vi "Lab Panel V2.8.vi"() -> ()   [LabVIEW 2013]
uses:
  <vilib>/Platform/TimedLoop/XDataNode/timing_clust.ctl
  <vilib>/Platform/TimedLoop/XDataNode/nitl_modes.ctl
  <vilib>/Platform/TimedLoop/XDataNode/wakeup.ctl
  <vilib>/platform/TimedLoop/XDataNode/XDataNode.xnode
  <vilib>/Platform/TimedLoop/XDataNode/XDNodeRunTimeDep.lvlib
panel:
  out "TEMP update":bool
  out "AI update":bool
  in  "stop":bool
  in  "Tab Control 2":T1(tab)
  out "LAB05-2 (SIG)":T2 {"PF" format="%.2f"; "AMPS" format="%.1f"}
  out "LAB05-1 (SIG)":T2 {"PF" format="%.2f"; "AMPS" format="%.1f"}
  out "LAB04-2 (SIG)":T2 {"PF" format="%.2f"; "AMPS" format="%.1f"}
  out "LAB04-1 (SIG)":T2 {"PF" format="%.2f"; "AMPS" format="%.1f"}
  out "LAB03-2 (SIG)":T2 {"PF" format="%.2f"; "AMPS" format="%.1f"}
  out "LAB03-1 (SIG)":T2 {"PF" format="%.2f"; "AMPS" format="%.1f"}
  out "LAB02-2 (SIG)":T2 {"PF" format="%.2f"; "AMPS" format="%.1f"}
  in  "LAB01-1RUN":bool
  in  "LAB05-1 (O/I)":bool
  in  "LAB05-2 (O/I)":bool
  in  "LAB04-1 (O/I)":bool
  in  "LAB04-2 (O/I)":bool
  in  "LAB02-1 (O/I)":bool
  in  "LAB02-2 (O/I)":bool
  in  "LAB01-2 (O/I)":bool
  in  "LAB01-1 (O/I)":bool
  in  "LAB03-1 (O/I)":bool
  in  "LAB05-2 RUN":bool
  in  "LAB05-1 RUN":bool
  in  "LAB04-2 RUN":bool
  in  "LAB04-1 RUN":bool
  in  "LAB03-2 RUN":bool
  in  "LAB03-1 RUN":bool
  in  "LAB02-2 RUN":bool
  in  "LAB02-1 RUN":bool
  in  "LAB01-2 RUN":bool
  in  "LAB05-2 SELECT":T3(radio)
  in  "LAB05-1 SELECT":T3(radio)
  in  "LAB04-2 SELECT":T3(radio)
  in  "LAB04-1 SELECT":T3(radio)
  in  "LAB03-2 SELECT":T3(radio)
  in  "LAB03-1 SELECT":T3(radio)
  in  "LAB02-2 SELECT":T3(radio)
  in  "LAB02-1 SELECT":T3(radio)
  in  "LAB01-2 SELECT":T3(radio)
  in  "LAB01-1 SELECT":T3(radio)
  in  "LAB03-2 (O/I)":bool
  out "LAB01-1 (SIG)":T2 {"PF" format="%.2f"; "AMPS" format="%.1f"}
  out "LAB01-2 (SIG)":T2 {"PF" format="%.2f"; "AMPS" format="%.1f"}
  out "LAB02-1 (SIG)":T2 {"PF" format="%.2f"; "AMPS" format="%.1f"}
  out "LAB05-2 (DISP)":T4 {"MINS" format="%.2g"}
  out "LAB05-1 (DISP)":T4 {"MINS" format="%.2g"}
  out "LAB04-2 (DISP)":T4 {"MINS" format="%.2g"}
  out "LAB04-1 (DISP)":T4 {"MINS" format="%.2g"}
  out "LAB03-2 (DISP)":T4 {"MINS" format="%.2g"}
  out "LAB03-1 (DISP)":T4 {"MINS" format="%.2g"}
  in  "LAB05-2 (SET)":T5
  in  "LAB05-1 (SET)":T5
  in  "LAB04-2 (SET)":T5
  in  "LAB04-1 (SET)":T5
  in  "LAB03-2 (SET)":T5
  in  "LAB03-1 (SET)":T5
  out "LAB02-2 (DISP)":T4 {"MINS" format="%.2g"}
  out "LAB02-1 (DISP)":T4 {"MINS" format="%.2g"}
  in  "LAB02-2 (SET)":T5
  in  "LAB02-1 (SET)":T5
  out "LAB05-2 (RESULT)":bool
  out "LAB05-1 (RESULT)":bool
  out "LAB04-2 (RESULT)":bool
  out "LAB04-1 (RESULT)":bool
  out "LAB03-2 (RESULT)":bool
  out "LAB03-1 (RESULT)":bool
  out "LAB02-2 (RESULT)":bool
  out "LAB02-1 (RESULT)":bool
  out "LAB01-2 (RESULT)":bool
  out "LAB01-1 (RESULT)":bool
  in  "LAB01-1 (SET)":T5
  in  "LAB01-2(SET)":T5
  out "LAB01-1 (DISP)":T4 {"MINS" format="%.2g"}
  out "LAB01-2 (DISP)":T4 {"MINS" format="%.2f"}
  out "LAB05-2 (TEMP START)":cluster{"TL":dbl, "TN":dbl}
  out "LAB04-2 (TEMP START)":cluster{"TL":dbl, "TN":dbl}
  out "LAB03-2 (TEMP START)":cluster{"TL":dbl, "TN":dbl}
  out "LAB02-2 (TEMP START)":cluster{"TL":dbl, "TN":dbl}
  out "LAB01-2 (TEMP START)":cluster{"TL":dbl, "TN":dbl}
  out "LAB05-1 (TEMP START)":cluster{"TL":dbl, "TN":dbl}
  out "LAB04-1 (TEMP START)":cluster{"TL":dbl, "TN":dbl}
  out "LAB03-1 (TEMP START)":cluster{"TL":dbl, "TN":dbl}
  out "LAB02-1 (TEMP START)":cluster{"TL":dbl, "TN":dbl}
  out "LAB01-1 (TEMP START)":cluster{"TL":dbl, "TN":dbl}
  in  "JIG ON TIME (S)":dbl=1.0 min=1.0 max=10.0 step=0.5 format="%.1g"
  in  "JIG OFF TIME (S)":dbl=2.0 min=2.0 max=10.0 step=0.5 format="%.1g"
  out "LAB01-1 (JIG)":bool
  out "LAB01-2 (JIG)":bool
  out "LAB02-1 (JIG)":bool
  out "LAB02-2 (JIG)":bool
  out "LAB03-1 (JIG)":bool
  out "LAB03-2 (JIG)":bool
  out "LAB04-1 (JIG)":bool
  out "LAB04-2 (JIG)":bool
  out "LAB05-1 (JIG)":bool
  out "LAB05-2 (JIG)":bool
  out "LAB01 (CAL)":T6 {"2 (TN) cal" min=0.0 step=0.01 format="%.2f"; "2 (TL) cal" min=0.0 step=0.01 format="%.2f"; "2 (PF) cal" min=0.0 step=0.01 format="%.2f"; "2 (V) cal" min=0.0 step=0.01 format="%.2f"; "2 (A) cal" min=0.0 step=0.01 format="%.2f"; "1 (TN) cal" min=0.0 step=0.01 format="%.2f"; "1 (TL) cal" min=0.0 step=0.01 format="%.2f"; "1 (PF) cal" min=0.0 step=0.01 format="%.2f"; "1 (V) cal" min=0.0 step=0.01 format="%.2f"; "1  (A) cal" min=0.0 step=0.01 format="%.2f"}
  out "LAB03 (CAL)":T6 {"2 (TN) cal" min=0.0 step=0.01 format="%.2f"; "2 (TL) cal" min=0.0 step=0.01 format="%.2f"; "2 (PF) cal" min=0.0 step=0.01 format="%.2f"; "2 (V) cal" min=0.0 step=0.01 format="%.2f"; "2 (A) cal" min=0.0 step=0.01 format="%.2f"; "1 (TN) cal" min=0.0 step=0.01 format="%.2f"; "1 (TL) cal" min=0.0 step=0.01 format="%.2f"; "1 (PF) cal" min=0.0 step=0.01 format="%.2f"; "1 (V) cal" min=0.0 step=0.01 format="%.2f"; "1  (A) cal" min=0.0 step=0.01 format="%.2f"}
  out "LAB02 (CAL)":T7 {"2 (TN) cal" min=0.0 step=0.01 format="%.2f"; "2 (TL) cal" min=0.0 step=0.01 format="%.2f"; "2 (PF) cal" min=0.0 step=0.01 format="%.2f"; "2 (V) cal" min=0.0 step=0.01 format="%.2f"; "2 (A) cal" min=0.0 step=0.01 format="%.2f"; "1 (TN) cal" min=0.0 step=0.01 format="%.2f"; "1 (TL) cal" min=0.0 step=0.01 format="%.2f"; "1 (PF) cal" min=0.0 step=0.01 format="%.2f"; "1 (V) cal" min=0.0 step=0.01 format="%.2f"; "1 (A) cal" min=0.0 step=0.01 format="%.2f"}
  out "LAB05 (CAL)":T6 {"2 (TN) cal" min=0.0 step=0.01 format="%.2f"; "2 (TL) cal" min=0.0 step=0.01 format="%.2f"; "2 (PF) cal" min=0.0 step=0.01 format="%.2f"; "2 (V) cal" min=0.0 step=0.01 format="%.2f"; "2 (A) cal" min=0.0 step=0.01 format="%.2f"; "1 (TN) cal" min=0.0 step=0.01 format="%.2f"; "1 (TL) cal" min=0.0 step=0.01 format="%.2f"; "1 (PF) cal" min=0.0 step=0.01 format="%.2f"; "1 (V) cal" min=0.0 step=0.01 format="%.2f"; "1  (A) cal" min=0.0 step=0.01 format="%.2f"}
  out "LAB04 (CAL)":T6 {"2 (TN) cal" min=0.0 step=0.01 format="%.2f"; "2 (TL) cal" min=0.0 step=0.01 format="%.2f"; "2 (PF) cal" min=0.0 step=0.01 format="%.2f"; "2 (V) cal" min=0.0 step=0.01 format="%.2f"; "2 (A) cal" min=0.0 step=0.01 format="%.2f"; "1 (TN) cal" min=0.0 step=0.01 format="%.2f"; "1 (TL) cal" min=0.0 step=0.01 format="%.2f"; "1 (PF) cal" min=0.0 step=0.01 format="%.2f"; "1 (V) cal" min=0.0 step=0.01 format="%.2f"; "1  (A) cal" min=0.0 step=0.01 format="%.2f"}
  out "calibration file error out":errorcluster
  in  "CALIBRATE":bool
  out "LAB01-1 (FAIL HI)":dbl
  out "LAB01-1 (FAIL LO)":dbl
  in  "Amps fail level":dbl=1.0 min=1.0 max=100.0 step=1.0
  in  "Tab Control":T8(tab)
  out "LAB01-2 (GRAPH)":dynamicdata(graph)
  out "LAB01-1 (GRAPH)":dynamicdata(graph)
  out "LAB02-2 (GRAPH)":dynamicdata(graph)
  out "LAB02-1 (GRAPH)":dynamicdata(graph)
  out "LAB03-2 (GRAPH)":dynamicdata(graph)
  out "LAB03-1 (GRAPH)":dynamicdata(graph)
  out "LAB04-2 (GRAPH)":dynamicdata(graph)
  out "LAB04-1 (GRAPH)":dynamicdata(graph)
  out "LAB05-2 (GRAPH)":dynamicdata(graph)
  out "LAB05-1 (GRAPH)":dynamicdata(graph)
  out "LAB05 TEMP":T9
  out "LAB04 TEMP":T9
  out "LAB02 TEMP":T9
  out "LAB01 TEMP":T9
  out "LAB03 TEMP":T9
  out "Analog Error Array":errorcluster[](array[cluster])
  out "AI loop time":dbl format="%.6g"
  out "loops":dbl
  in  "loop  delay(mS)":dbl
  out "on loops":dbl
  out "off loops":dbl
  out "jig cycle":dbl
  out "LAB01-1 (TDMS)":refnum<k34>
  out "data file error":errorcluster
  out "LAB02-1 (TDMS)":refnum<k34>
  out "LAB01-2 (TDMS)":refnum<k34>
  out "LAB02-2 (TDMS)":refnum<k34>
  out "LAB03-1 (TDMS)":refnum<k34>
  out "LAB03-2 (TDMS)":refnum<k34>
  out "LAB04-1 (TDMS)":refnum<k34>
  out "LAB04-2 (TDMS)":refnum<k34>
  out "LAB05-1 (TDMS)":refnum<k34>
  out "LAB05-2 (TDMS)":refnum<k34>
  # "LAB01"
  # "LAB02"
  # "LAB05"
  # "LAB03"
  # "LAB04"
  # "LAB01"
  # "LAB02"
  # "LAB03"
  # "LAB04"
  # "LAB05"
  # "JIG SET"
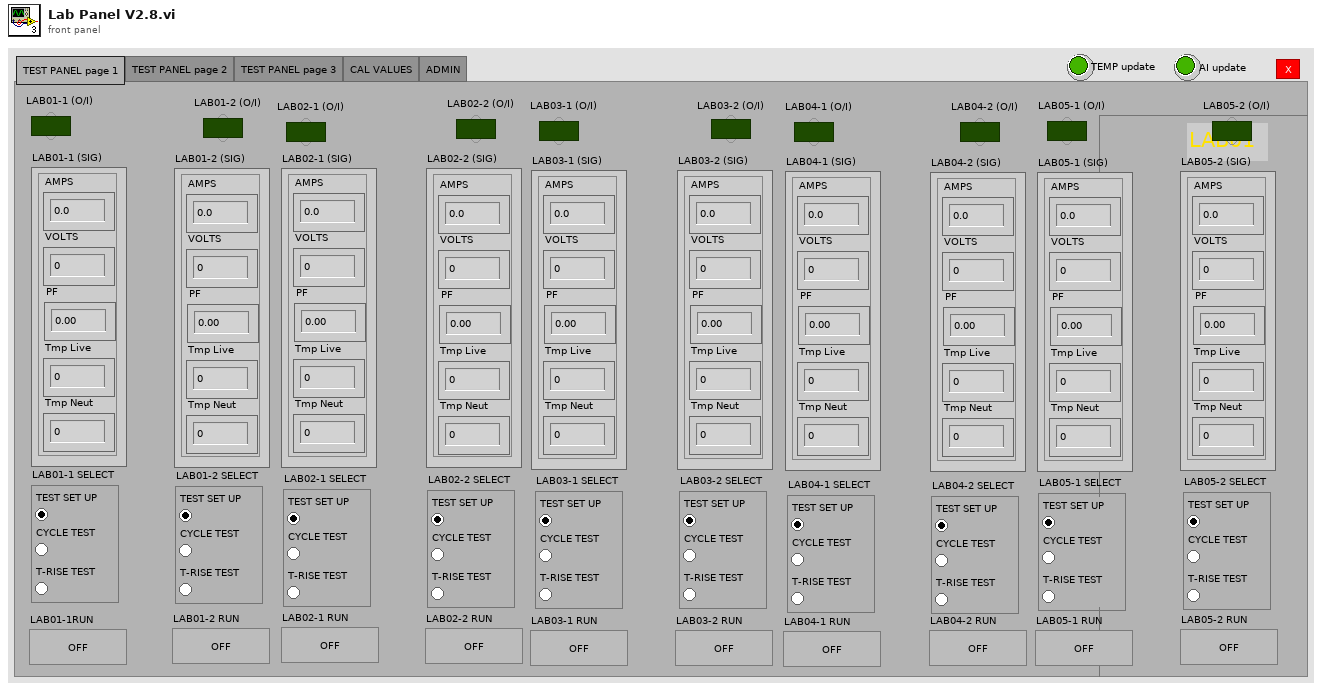
[diagram p1: front panel]
types:
  T1 = enum32{"TEST PANEL page 1", "TEST PANEL page 2", "TEST PANEL page 3", "CAL VALUES", "ADMIN"}
  T2 = cluster{"AMPS":dbl, "VOLTS":dbl, "PF":dbl, "Tmp Live":dbl, "Tmp Neut":dbl}
  T3 = enum32{"TEST SET UP", "CYCLE TEST", "T-RISE TEST"}
  T4 = cluster{"CYCLE":dbl, "MINS":dbl, "STATUS":string}
  T5 = cluster{"NAME":string, "DESCRIPTION":string, "CYCLES":dbl, "T-RISE mins":dbl, "T-RISE deg C":dbl}
  T6 = cluster{"1  (A) cal":dbl, "1 (V) cal":dbl, "1 (PF) cal":dbl, "1 (TL) cal":dbl, "1 (TN) cal":dbl, "2 (A) cal":dbl, "2 (V) cal":dbl, "2 (PF) cal":dbl, "2 (TL) cal":dbl, "2 (TN) cal":dbl}
  T7 = cluster{"1 (A) cal":dbl, "1 (V) cal":dbl, "1 (PF) cal":dbl, "1 (TL) cal":dbl, "1 (TN) cal":dbl, "2 (A) cal":dbl, "2 (V) cal":dbl, "2 (PF) cal":dbl, "2 (TL) cal":dbl, "2 (TN) cal":dbl}
  T8 = enum32{"LAB01", "LAB02", "LAB03", "LAB04", "LAB05", "TEMPERATURE", "ERROR"}
  T9 = cluster{"T1 Live":dbl, "T1 Neut":dbl, "T2 Live":dbl, "T2 Neut":dbl, "ID":dbl, "ER":dbl}
  T10 = typedef "XDNodeRunTimeDep.lvlib/timing_clust.ctl" = cluster{"Expected End [f-1]":u64, "Actual End [f-1]":u64, "Finished Late? [f-1]":bool, "Expected End [i-1]":u64, "Actual End [i-1]":u64, "Finished Late? [i-1]":bool, "Expected Start [i]":u64, "Actual Start [i]":u64, "Expected Start [f]":u64, "Actual Start [f]":u64, "Source Name":string, "Structure Name":string, "Period":i64, "Deadline":i64, "Offset":i64, "Start":i64, "Priority":i32, "Timeout":i32, "Mode":T11, "Wakeup Reason":T12, "Error":errorcluster, "Source Type":string, "Secondary Source Type":string, "Global End Time":u64, "Global Start Time":u64, "Frame Duration":u64, "Iteration Duration":u64, "Assigned CPU":i32, "I/O Scan Engine Mode":u32}
  T11 = typedef "XDNodeRunTimeDep.lvlib/nitl_modes.ctl" = enum32{"No Change", "Process missed periods, maintain original phase", "Discard missed periods, maintain original phase", "Process missed periods, ignore original phase", "Discard missed periods, ignore original phase"}
  T12 = typedef "XDNodeRunTimeDep.lvlib/wakeup.ctl" = enum32{"Normal", "Aborted", "Asynchronous wakeup", "Timing source error", "Timed loop error", "Timeout"}
  T13 = enum16{"open", "open or create", "create or replace", "create", "open (read-only)"}
  T14 = cluster{"T1":dbl, "T2":dbl, "T3":dbl, "T4":dbl, "ID":dbl, "ER":dbl}
  T15 = cluster{"LAB01-1 (A)":dbl, "LAB01-1 (V)":dbl, "LAB01-1 (PF)":dbl, "LAB01-2 (A)":dbl, "LAB01-2 (V)":dbl, "LAB01-2 (PF)":dbl}
  T16 = cluster{"LAB02-1 (A)":dbl, "LAB02-1 (V)":dbl, "LAB02-1 (PF)":dbl, "LAB02-2 (A)":dbl, "LAB02-2 (V)":dbl, "LAB02-2 (PF)":dbl}
  T17 = cluster{"LAB03-1 (A)":dbl, "LAB03-1 (V)":dbl, "LAB03-1 (PF)":dbl, "LAB03-2 (A)":dbl, "LAB03-2 (V)":dbl, "LAB03-2 (PF)":dbl}
  T18 = cluster{"LAB04-1 (A)":dbl, "LAB04-1 (V)":dbl, "LAB04-1 (PF)":dbl, "LAB04-2 (A)":dbl, "LAB04-2 (V)":dbl, "LAB04-2 (PF)":dbl}
  T19 = cluster{"LAB05-1 (A)":dbl, "LAB05-1 (V)":dbl, "LAB05-1 (PF)":dbl, "LAB05-2 (A)":dbl, "LAB05-2 (V)":dbl, "LAB05-2 (PF)":dbl}
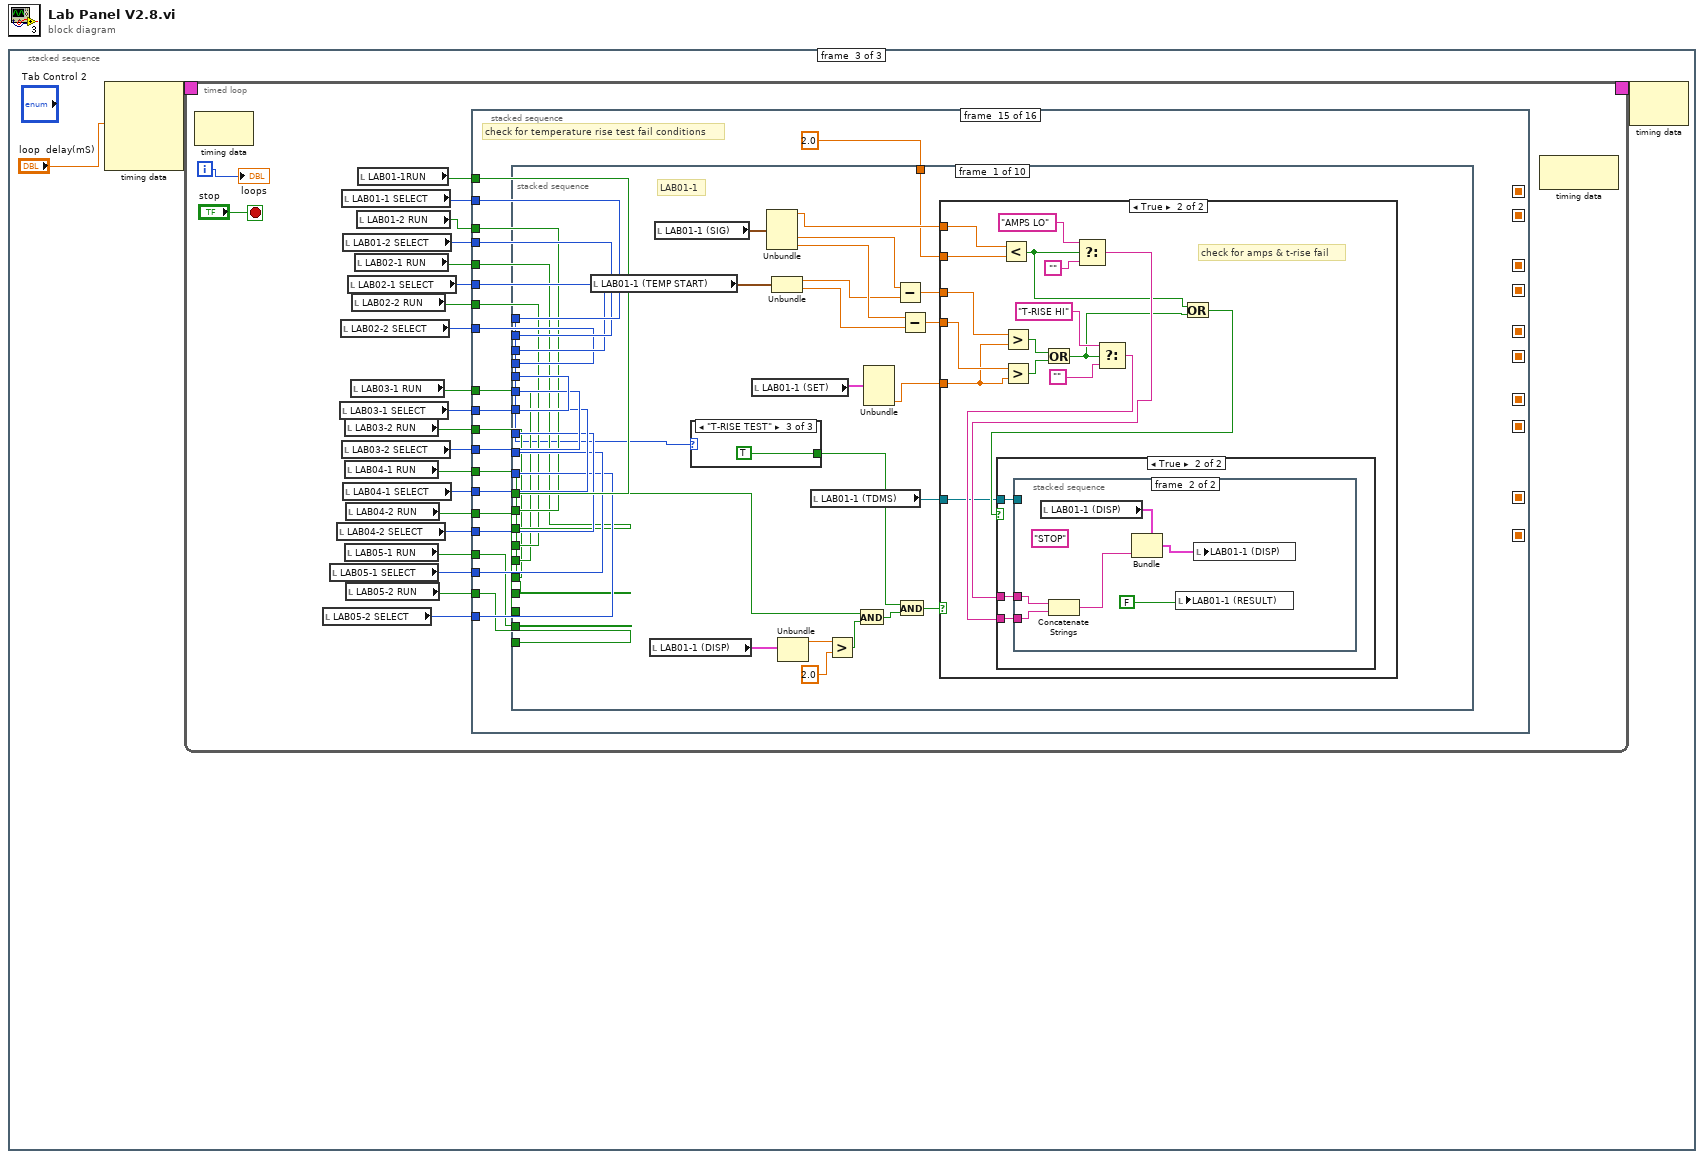
[diagram p0: block diagram]
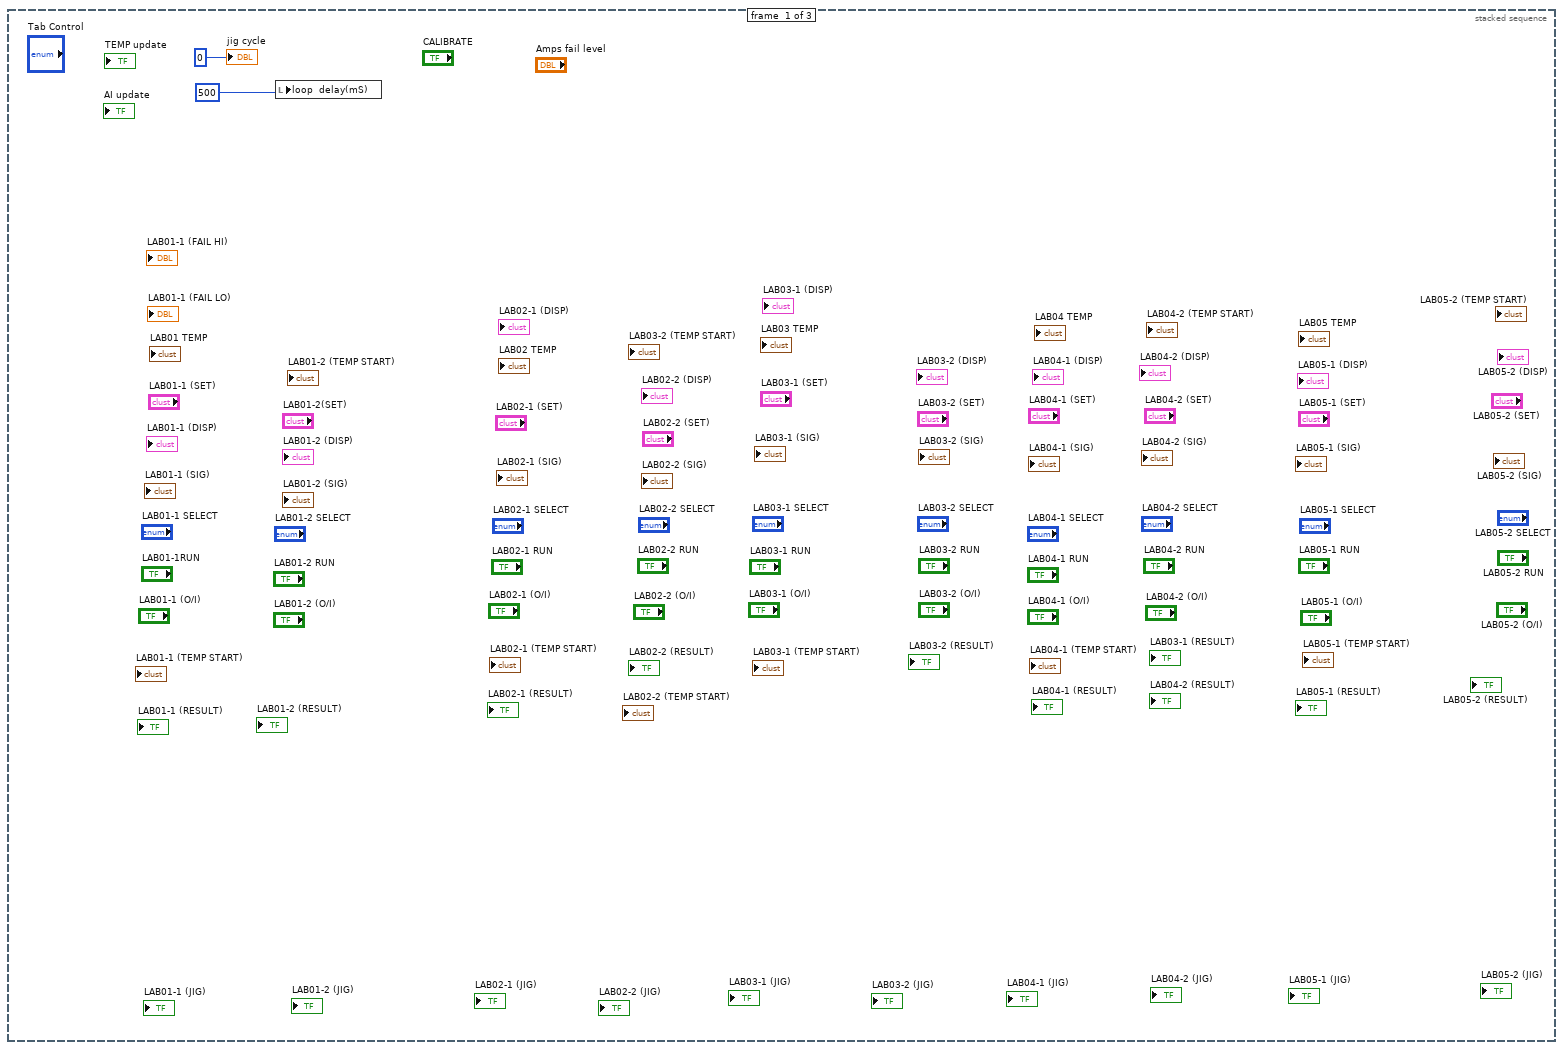
[diagram p2: hidden frame]
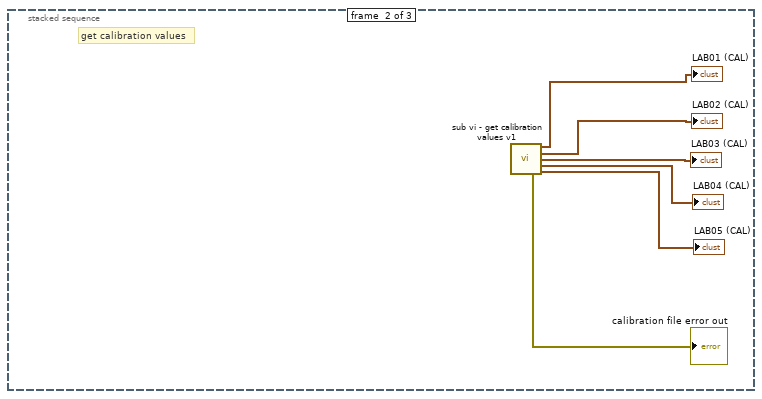
[diagram p3: hidden frame]
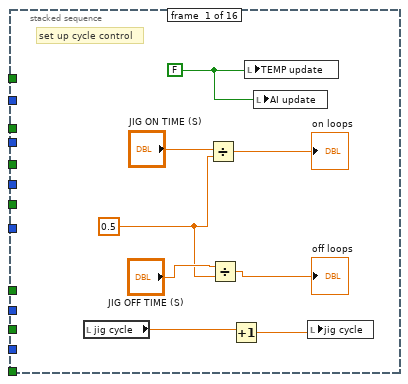
[diagram p4: hidden frame]
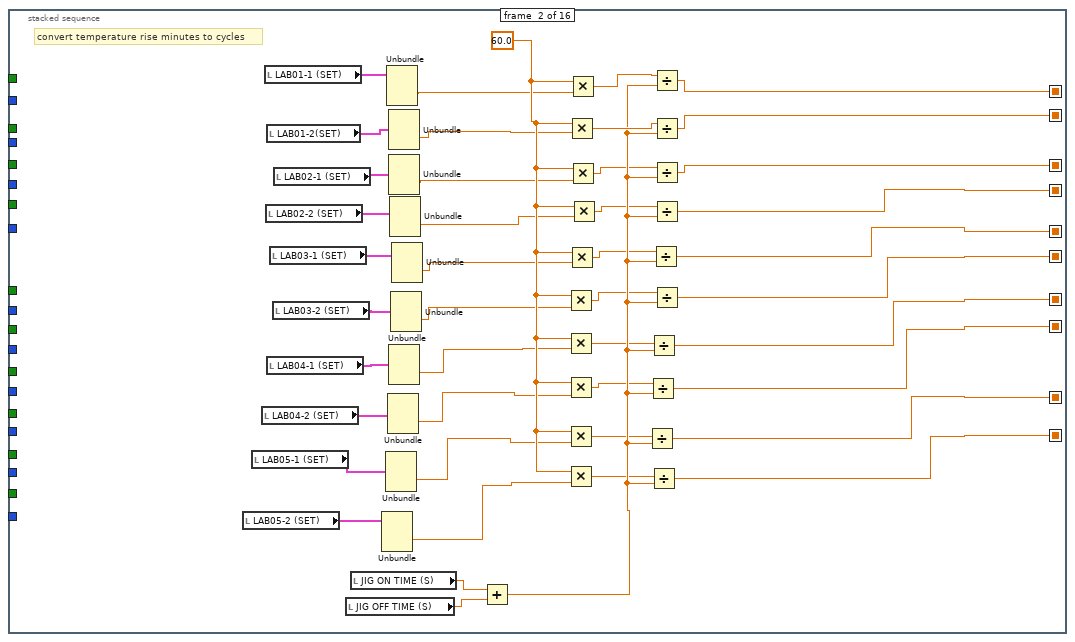
[diagram p5: hidden frame]
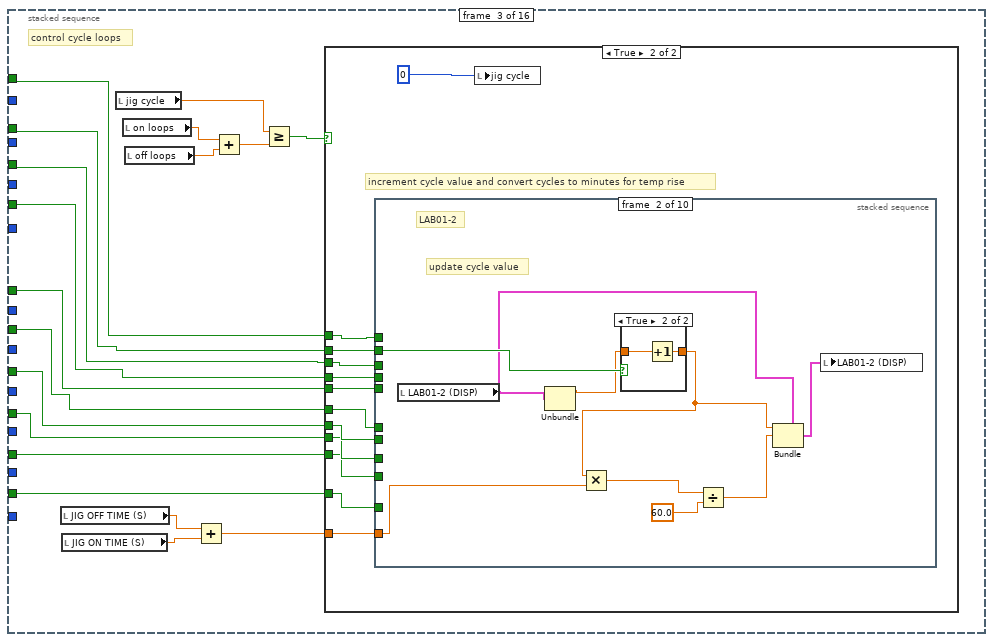
[diagram p6: hidden frame]
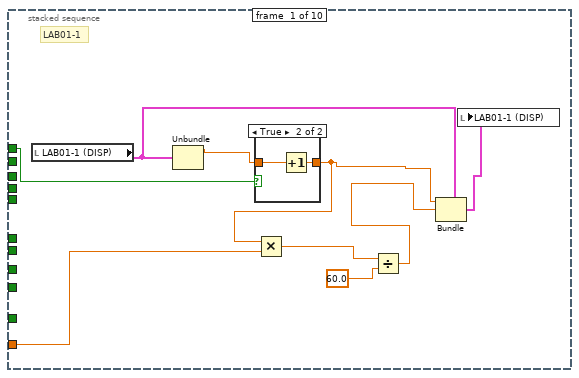
[diagram p8: hidden frame]
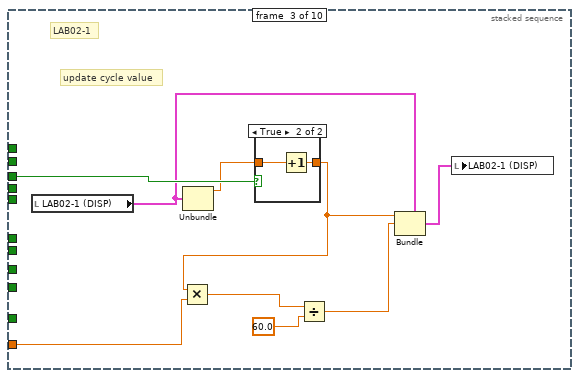
[diagram p11: hidden frame]
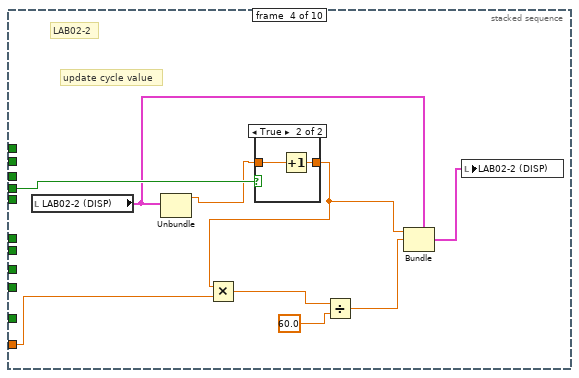
[diagram p13: hidden frame]
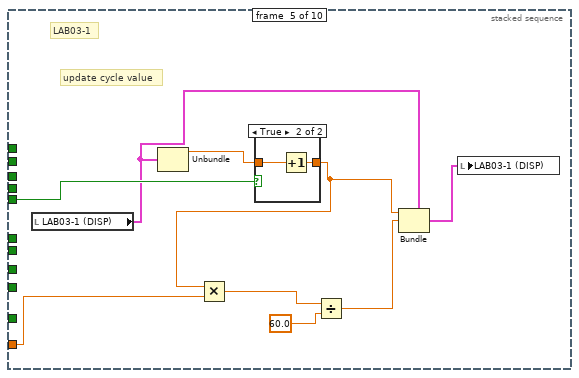
[diagram p15: hidden frame]
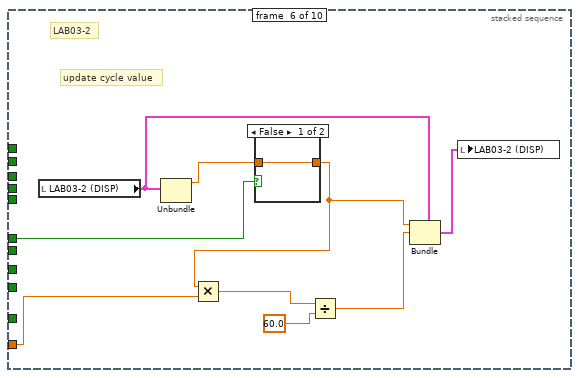
[diagram p17: hidden frame]
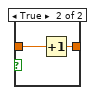
[diagram p18: hidden frame]
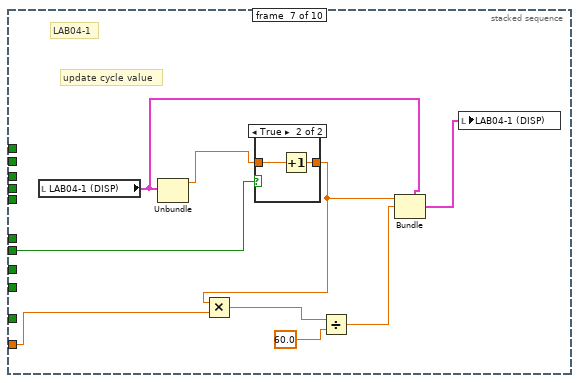
[diagram p19: hidden frame]
diagram:
  n1 = stacked-sequence {
    frame #0 {
      n2 = local write "loop  delay(mS)"(500) -> ()
      "jig cycle" <- 0
    }
    frame #1 {
      # "get calibration values"
      n3 = call "sub vi - get calibration values v1.vi"() -> ("LAB01 (CAL)"=→"LAB01 (CAL)":T6, "LAB02 (CAL)"=→"LAB02 (CAL)":T7, "LAB03 (CAL)"=→"LAB03 (CAL)":T6, "LAB04 (CAL)"=→"LAB04 (CAL)":T6, "calibration file error out"=→"calibration file error out":errorcluster, "LAB05 (CAL)"=→"LAB05 (CAL)":T6)  [unwired: 10 in]
    }
    frame #2 {
      n4 = node-c288("loop  delay(mS)") -> (w11:T10)  [unwired: 3 in]
      n5 = timed-loop {
        timing: w11 -> [_]
        timing-out: [_] -> w10
        i -> [w33]
        stop <- "stop" stop-if-true
        n6 = node-c288() -> ()  [unwired: 1 in, 1 out]
        n7 = local read "LAB05-2 SELECT"() -> (w12:T3)
        n8 = local read "LAB05-1 SELECT"() -> (w13:T3)
        n9 = local read "LAB04-2 SELECT"() -> (w14:T3)
        n10 = local read "LAB03-1 SELECT"() -> (w17:T3)
        n11 = local read "LAB02-2 SELECT"() -> (w18:T3)
        n12 = local read "LAB01-1 SELECT"() -> (w21:T3)
        n13 = local read "LAB03-2 SELECT"() -> (w16:T3)
        n14 = local read "LAB01-2 SELECT"() -> (w20:T3)
        n15 = local read "LAB04-1 SELECT"() -> (w15:T3)
        n16 = local read "LAB03-2 RUN"() -> (w26:bool)
        n17 = local read "LAB04-1 RUN"() -> (w25:bool)
        n18 = local read "LAB05-1 RUN"() -> (w23:bool)
        n19 = local read "LAB04-2 RUN"() -> (w24:bool)
        n20 = local read "LAB05-2 RUN"() -> (w22:bool)
        n21 = local read "LAB02-1 SELECT"() -> (w19:T3)
        n22 = local read "LAB03-1 RUN"() -> (w27:bool)
        n23 = local read "LAB02-2 RUN"() -> (w28:bool)
        n24 = local read "LAB02-1 RUN"() -> (w29:bool)
        n25 = local read "LAB01-2 RUN"() -> (w30:bool)
        n26 = local read "LAB01-1RUN"() -> (w31:bool)
        n27 = stacked-sequence {
          seq-local: [_ w85 _ _ _ _ _ _ _ _ _ _ _ _ _ _] -> [_ _ _ _ _ w1464 _ _ _ _ _ _ _ _ _ _]
          seq-local: [_ w84 _ _ _ _ _ _ _ _ _ _ _ _ _ _] -> [_ _ _ _ _ _ _ _ _ _ _ _ _ _ _ _]
          seq-local: [_ w71 _ _ _ _ _ _ _ _ _ _ _ _ _ _] -> [_ _ _ _ _ _ _ _ _ _ _ _ _ _ _ _]
          seq-local: [_ w70 _ _ _ _ _ _ _ _ _ _ _ _ _ _] -> [_ _ _ _ _ _ _ _ _ _ _ _ _ _ _ _]
          seq-local: [_ w69 _ _ _ _ _ _ _ _ _ _ _ _ _ _] -> [_ _ _ _ _ _ _ _ _ _ _ _ _ _ _ _]
          seq-local: [_ w68 _ _ _ _ _ _ _ _ _ _ _ _ _ _] -> [_ _ _ _ _ _ _ _ _ _ _ _ _ _ _ _]
          seq-local: [_ w67 _ _ _ _ _ _ _ _ _ _ _ _ _ _] -> [_ _ _ _ _ _ _ _ _ _ _ _ _ _ _ _]
          seq-local: [_ w66 _ _ _ _ _ _ _ _ _ _ _ _ _ _] -> [_ _ _ _ _ _ _ _ _ _ _ _ _ _ _ _]
          seq-local: [_ w65 _ _ _ _ _ _ _ _ _ _ _ _ _ _] -> [_ _ _ _ _ _ _ _ _ _ _ _ _ _ _ _]
          seq-local: [_ w64 _ _ _ _ _ _ _ _ _ _ _ _ _ _] -> [_ _ _ _ _ _ _ _ _ _ _ _ _ _ _ _]
          tunnel: w31 -> [_ _ w101 w257 w1064 w1475 w1785 w1848 _ _ _ _ w2351 w2840 w3390 _]
          tunnel: w30 -> [_ _ w100 w255 w1063 w1474 w1784 _ _ _ _ _ w2350 w2838 w3380 _]
          tunnel: w29 -> [_ _ w99 w253 w1062 w1473 w1783 _ _ _ _ _ w2349 w2836 w3379 _]
          tunnel: w28 -> [_ _ w98 w251 w1061 w1472 w1782 _ _ _ _ _ w2348 w2834 w3378 _]
          tunnel: w27 -> [_ _ w97 w249 w1060 w1471 w1781 _ _ _ _ _ w2347 w2832 w3377 _]
          tunnel: w26 -> [_ _ w96 w247 w1059 w1470 w1780 _ _ _ _ _ w2346 w2830 w3376 _]
          tunnel: w25 -> [_ _ w95 w245 w1058 w1469 w1779 _ _ _ _ _ w2345 w2828 w3372 _]
          tunnel: w24 -> [_ _ w94 w243 w1057 w1468 w1778 _ _ _ _ _ w2344 w2826 w3375 _]
          tunnel: w23 -> [_ _ w93 w241 w1056 w1467 w1777 _ _ _ _ _ w2343 w2824 w3374 _]
          tunnel: w22 -> [_ _ w92 w239 w1055 w1466 w1776 _ _ _ _ _ w2342 w2822 w3373 _]
          tunnel: w21 -> [_ _ _ w256 w1054 w1465 _ _ _ _ _ _ _ w2842 w3391 _]
          tunnel: w20 -> [_ _ _ w254 w1053 w1463 _ _ _ _ _ _ _ w2837 w3389 _]
          tunnel: w19 -> [_ _ _ w252 w1052 w1462 _ _ _ _ _ _ _ w2835 w3388 _]
          tunnel: w18 -> [_ _ _ w250 w1051 w1461 _ _ _ _ _ _ _ w2833 w3387 _]
          tunnel: w17 -> [_ _ _ w248 w1050 w1460 _ _ _ _ _ _ _ w2831 w3386 _]
          tunnel: w16 -> [_ _ _ w246 w1049 w1459 _ _ _ _ _ _ _ w2829 w3385 _]
          tunnel: w15 -> [_ _ _ w244 w1048 w1458 _ _ _ _ _ _ _ w2827 w3384 _]
          tunnel: w14 -> [_ _ _ w242 w1047 w1457 _ _ _ _ _ _ _ w2825 w3383 _]
          tunnel: w13 -> [_ _ _ w240 w1046 w1456 _ _ _ _ _ _ _ w2823 w3382 _]
          tunnel: w12 -> [_ _ _ w238 w1045 w1455 _ _ _ _ _ _ _ w2821 w3381 _]
          frame #0 {
            w36 = FALSE
            w41 = 0.5
            # "set up cycle control"
            n28 = local read "jig cycle"() -> (w40:dbl)
            n29 = Divide(x="JIG ON TIME (S)", y=w41) -> (x/y=→"on loops":dbl)
            n30 = Divide(x="JIG OFF TIME (S)", y=w41) -> (x/y=→"off loops":dbl)
            n31 = Increment(x=w40) -> (x+1=w39:dbl)
            n32 = local write "TEMP update"(w36) -> ()
            n33 = local write "AI update"(w36) -> ()
            n34 = local write "jig cycle"(w39) -> ()
          }
          frame #1 {
            w81 = 60.0
            # "convert temperature rise minutes to cycles"
            n35 = local read "LAB05-2 (SET)"() -> (w45:T5)
            n36 = local read "LAB05-1 (SET)"() -> (w47:T5)
            n37 = local read "LAB04-2 (SET)"() -> (w49:T5)
            n38 = local read "LAB01-1 (SET)"() -> (w63:T5)
            n39 = local read "LAB02-2 (SET)"() -> (w57:T5)
            n40 = local read "LAB01-2(SET)"() -> (w61:T5)
            n41 = local read "LAB04-1 (SET)"() -> (w51:T5)
            n42 = local read "LAB03-1 (SET)"() -> (w55:T5)
            n43 = local read "LAB03-2 (SET)"() -> (w53:T5)
            n44 = local read "LAB02-1 (SET)"() -> (w59:T5)
            n45 = local read "JIG OFF TIME (S)"() -> (w86:dbl)
            n46 = local read "JIG ON TIME (S)"() -> (w87:dbl)
            n47 = Unbundle(w45) -> ("T-RISE mins"=w44:dbl)  [unwired: 4 out]
            n48 = Unbundle(w47) -> ("T-RISE mins"=w46:dbl)  [unwired: 4 out]
            n49 = Unbundle(w63) -> ("T-RISE mins"=w62:dbl)  [unwired: 4 out]
            n50 = Unbundle(w49) -> ("T-RISE mins"=w48:dbl)  [unwired: 4 out]
            n51 = Unbundle(w61) -> ("T-RISE mins"=w60:dbl)  [unwired: 4 out]
            n52 = Unbundle(w59) -> ("T-RISE mins"=w58:dbl)  [unwired: 4 out]
            n53 = Unbundle(w51) -> ("T-RISE mins"=w50:dbl)  [unwired: 4 out]
            n54 = Unbundle(w57) -> ("T-RISE mins"=w56:dbl)  [unwired: 4 out]
            n55 = Unbundle(w53) -> ("T-RISE mins"=w52:dbl)  [unwired: 4 out]
            n56 = Unbundle(w55) -> ("T-RISE mins"=w54:dbl)  [unwired: 4 out]
            n57 = Add(x=w87, y=w86) -> (x+y=w80:dbl)
            n58 = Multiply(x=w81, y=w52) -> (x*y=w76:dbl)
            n59 = Multiply(x=w81, y=w50) -> (x*y=w75:dbl)
            n60 = Multiply(x=w81, y=w48) -> (x*y=w74:dbl)
            n61 = Multiply(x=w81, y=w46) -> (x*y=w73:dbl)
            n62 = Multiply(x=w81, y=w44) -> (x*y=w72:dbl)
            n63 = Multiply(x=w81, y=w60) -> (x*y=w82:dbl)
            n64 = Multiply(x=w81, y=w54) -> (x*y=w77:dbl)
            n65 = Multiply(x=w81, y=w62) -> (x*y=w83:dbl)
            n66 = Multiply(x=w81, y=w58) -> (x*y=w79:dbl)
            n67 = Multiply(x=w81, y=w56) -> (x*y=w78:dbl)
            n68 = Divide(x=w73, y=w80) -> (x/y=w65:dbl)
            n69 = Divide(x=w74, y=w80) -> (x/y=w66:dbl)
            n70 = Divide(x=w75, y=w80) -> (x/y=w67:dbl)
            n71 = Divide(x=w72, y=w80) -> (x/y=w64:dbl)
            n72 = Divide(x=w77, y=w80) -> (x/y=w69:dbl)
            n73 = Divide(x=w83, y=w80) -> (x/y=w85:dbl)
            n74 = Divide(x=w82, y=w80) -> (x/y=w84:dbl)
            n75 = Divide(x=w79, y=w80) -> (x/y=w71:dbl)
            n76 = Divide(x=w78, y=w80) -> (x/y=w70:dbl)
            n77 = Divide(x=w76, y=w80) -> (x/y=w68:dbl)
          }
          frame #2 {
            # "control cycle loops"
            n78 = local read "JIG OFF TIME (S)"() -> (w90:dbl)
            n79 = local read "JIG ON TIME (S)"() -> (w89:dbl)
            n80 = local read "jig cycle"() -> (w103:dbl)
            n81 = local read "on loops"() -> (w105:dbl)
            n82 = local read "off loops"() -> (w104:dbl)
            n83 = Add(x=w90, y=w89) -> (x+y=w88:dbl)
            n84 = Add(x=w105, y=w104) -> (x+y=w91:dbl)
            n85 = Greater Or Equal?(x=w103, y=w91) -> (x >= y?=w102:bool)
            n86 = case shown="True" w102 {
              tunnel: w101 -> [_ w116]
              tunnel: w100 -> [_ w115]
              tunnel: w99 -> [_ w114]
              tunnel: w98 -> [_ w113]
              tunnel: w97 -> [_ w112]
              tunnel: w96 -> [_ w111]
              tunnel: w95 -> [_ w110]
              tunnel: w94 -> [_ w109]
              tunnel: w93 -> [_ w108]
              tunnel: w92 -> [_ w107]
              tunnel: w88 -> [_ w106]
              frame False {
              }
              frame True {
                # "increment cycle value and convert cycles to minutes for temp rise"
                n87 = stacked-sequence {
                  tunnel: w116 -> [w126 _ _ _ _ _ _ _ _ _]
                  tunnel: w115 -> [_ w138 _ _ _ _ _ _ _ _]
                  tunnel: w114 -> [_ _ w150 _ _ _ _ _ _ _]
                  tunnel: w113 -> [_ _ _ w162 _ _ _ _ _ _]
                  tunnel: w112 -> [_ _ _ _ w174 _ _ _ _ _]
                  tunnel: w111 -> [_ _ _ _ _ w186 _ _ _ _]
                  tunnel: w110 -> [_ _ _ _ _ _ w198 _ _ _]
                  tunnel: w109 -> [_ _ _ _ _ _ _ w210 _ _]
                  tunnel: w108 -> [_ _ _ _ _ _ _ _ w222 _]
                  tunnel: w107 -> [_ _ _ _ _ _ _ _ _ w234]
                  tunnel: w106 -> [w123 w135 w147 w159 w171 w183 w195 w207 w219 w231]
                  frame #0 {
                    # "LAB01-1"
                    n88 = local read "LAB01-1 (DISP)"() -> (w121:T4)
                    n89 = Unbundle(w121) -> ("CYCLE"=w122:dbl)  [unwired: 2 out]
                    n90 = case shown="True" w126 {
                      tunnel: w122 -> [w127 w129]
                      tunnel: [w127 w128] -> w120
                      frame False {
                      }
                      frame True {
                        n91 = Increment(x=w129) -> (x+1=w128:dbl)
                      }
                    }
                    n92 = Multiply(x=w120, y=w123) -> (x*y=w124:dbl)
                    n93 = Divide(x=w124, y=60.0) -> (x/y=w119:dbl)
                    n94 = Bundle(cluster=w121, "CYCLE"=w120, "MINS"=w119) -> (w118:T4)  [unwired: 1 in]
                    n95 = local write "LAB01-1 (DISP)"(w118) -> ()
                  }
                  frame #1 {
                    # "update cycle value"
                    # "LAB01-2"
                    n96 = local read "LAB01-2 (DISP)"() -> (w133:T4)
                    n97 = Unbundle(w133) -> ("CYCLE"=w134:dbl)  [unwired: 2 out]
                    n98 = case shown="True" w138 {
                      tunnel: w134 -> [w139 w141]
                      tunnel: [w139 w140] -> w131
                      frame False {
                      }
                      frame True {
                        n99 = Increment(x=w141) -> (x+1=w140:dbl)
                      }
                    }
                    n100 = Multiply(x=w131, y=w135) -> (x*y=w136:dbl)
                    n101 = Divide(x=w136, y=60.0) -> (x/y=w130:dbl)
                    n102 = Bundle(cluster=w133, "CYCLE"=w131, "MINS"=w130) -> (w132:T4)  [unwired: 1 in]
                    n103 = local write "LAB01-2 (DISP)"(w132) -> ()
                  }
                  frame #2 {
                    # "update cycle value"
                    # "LAB02-1"
                    n104 = local read "LAB02-1 (DISP)"() -> (w145:T4)
                    n105 = Unbundle(w145) -> ("CYCLE"=w146:dbl)  [unwired: 2 out]
                    n106 = case shown="True" w150 {
                      tunnel: [w151 w153] -> w143
                      tunnel: w146 -> [w151 w152]
                      frame False {
                      }
                      frame True {
                        n107 = Increment(x=w152) -> (x+1=w153:dbl)
                      }
                    }
                    n108 = Multiply(x=w143, y=w147) -> (x*y=w148:dbl)
                    n109 = Divide(x=w148, y=60.0) -> (x/y=w142:dbl)
                    n110 = Bundle(cluster=w145, "CYCLE"=w143, "MINS"=w142) -> (w144:T4)  [unwired: 1 in]
                    n111 = local write "LAB02-1 (DISP)"(w144) -> ()
                  }
                  frame #3 {
                    # "update cycle value"
                    # "LAB02-2"
                    n112 = local read "LAB02-2 (DISP)"() -> (w157:T4)
                    n113 = Unbundle(w157) -> ("CYCLE"=w158:dbl)  [unwired: 2 out]
                    n114 = case shown="True" w162 {
                      tunnel: [w163 w165] -> w156
                      tunnel: w158 -> [w163 w164]
                      frame False {
                      }
                      frame True {
                        n115 = Increment(x=w164) -> (x+1=w165:dbl)
                      }
                    }
                    n116 = Multiply(x=w156, y=w159) -> (x*y=w160:dbl)
                    n117 = Divide(x=w160, y=60.0) -> (x/y=w155:dbl)
                    n118 = Bundle(cluster=w157, "CYCLE"=w156, "MINS"=w155) -> (w154:T4)  [unwired: 1 in]
                    n119 = local write "LAB02-2 (DISP)"(w154) -> ()
                  }
                  frame #4 {
                    # "update cycle value"
                    # "LAB03-1"
                    n120 = local read "LAB03-1 (DISP)"() -> (w169:T4)
                    n121 = Unbundle(w169) -> ("CYCLE"=w170:dbl)  [unwired: 2 out]
                    n122 = case shown="True" w174 {
                      tunnel: [w175 w177] -> w166
                      tunnel: w170 -> [w175 w176]
                      frame False {
                      }
                      frame True {
                        n123 = Increment(x=w176) -> (x+1=w177:dbl)
                      }
                    }
                    n124 = Multiply(x=w166, y=w171) -> (x*y=w172:dbl)
                    n125 = Divide(x=w172, y=60.0) -> (x/y=w167:dbl)
                    n126 = Bundle(cluster=w169, "CYCLE"=w166, "MINS"=w167) -> (w168:T4)  [unwired: 1 in]
                    n127 = local write "LAB03-1 (DISP)"(w168) -> ()
                  }
                  frame #5 {
                    # "update cycle value"
                    # "LAB03-2"
                    n128 = local read "LAB03-2 (DISP)"() -> (w181:T4)
                    n129 = Unbundle(w181) -> ("CYCLE"=w182:dbl)  [unwired: 2 out]
                    n130 = case shown="False" w186 {
                      tunnel: [w187 w189] -> w180
                      tunnel: w182 -> [w187 w188]
                      frame False {
                      }
                      frame True {
                        n131 = Increment(x=w188) -> (x+1=w189:dbl)
                      }
                    }
                    n132 = Multiply(x=w180, y=w183) -> (x*y=w184:dbl)
                    n133 = Divide(x=w184, y=60.0) -> (x/y=w179:dbl)
                    n134 = Bundle(cluster=w181, "CYCLE"=w180, "MINS"=w179) -> (w178:T4)  [unwired: 1 in]
                    n135 = local write "LAB03-2 (DISP)"(w178) -> ()
                  }
                  frame #6 {
                    # "update cycle value"
                    # "LAB04-1"
                    n136 = local read "LAB04-1 (DISP)"() -> (w193:T4)
                    n137 = Unbundle(w193) -> ("CYCLE"=w194:dbl)  [unwired: 2 out]
                    n138 = case shown="True" w198 {
                      tunnel: [w199 w201] -> w191
                      tunnel: w194 -> [w199 w200]
                      frame False {
                      }
                      frame True {
                        n139 = Increment(x=w200) -> (x+1=w201:dbl)
                      }
                    }
                    n140 = Multiply(x=w191, y=w195) -> (x*y=w196:dbl)
                    n141 = Divide(x=w196, y=60.0) -> (x/y=w190:dbl)
                    n142 = Bundle(cluster=w193, "CYCLE"=w191, "MINS"=w190) -> (w192:T4)  [unwired: 1 in]
                    n143 = local write "LAB04-1 (DISP)"(w192) -> ()
                  }
                  frame #7 {
                    # "update cycle value"
                    # "LAB04-2"
                    n144 = local read "LAB04-2 (DISP)"() -> (w205:T4)
                    n145 = Unbundle(w205) -> ("CYCLE"=w206:dbl)  [unwired: 2 out]
                    n146 = case shown="True" w210 {
                      tunnel: [w211 w213] -> w203
                      tunnel: w206 -> [w211 w212]
                      frame False {
                      }
                      frame True {
                        n147 = Increment(x=w212) -> (x+1=w213:dbl)
                      }
                    }
                    n148 = Multiply(x=w203, y=w207) -> (x*y=w209:dbl)
                    n149 = Divide(x=w209, y=60.0) -> (x/y=w202:dbl)
                    n150 = Bundle(cluster=w205, "CYCLE"=w203, "MINS"=w202) -> (w204:T4)  [unwired: 1 in]
                    n151 = local write "LAB04-2 (DISP)"(w204) -> ()
                  }
                  frame #8 {
                    # "update cycle value"
                    # "LAB05-1"
                    n152 = local read "LAB05-1 (DISP)"() -> (w217:T4)
                    n153 = Unbundle(w217) -> ("CYCLE"=w218:dbl)  [unwired: 2 out]
                    n154 = case shown="True" w222 {
                      tunnel: [w223 w225] -> w215
                      tunnel: w218 -> [w223 w224]
                      frame False {
                      }
                      frame True {
                        n155 = Increment(x=w224) -> (x+1=w225:dbl)
                      }
                    }
                    n156 = Multiply(x=w215, y=w219) -> (x*y=w220:dbl)
                    n157 = Divide(x=w220, y=60.0) -> (x/y=w214:dbl)
                    n158 = Bundle(cluster=w217, "CYCLE"=w215, "MINS"=w214) -> (w216:T4)  [unwired: 1 in]
                    n159 = local write "LAB05-1 (DISP)"(w216) -> ()
                  }
                  frame #9 {
                    # "update cycle value"
                    # "LAB05-2"
                    n160 = local read "LAB05-2 (DISP)"() -> (w230:T4)
                    n161 = Unbundle(w230) -> ("CYCLE"=w229:dbl)  [unwired: 2 out]
                    n162 = case shown="True" w234 {
                      tunnel: [w235 w237] -> w228
                      tunnel: w229 -> [w235 w236]
                      frame False {
                      }
                      frame True {
                        n163 = Increment(x=w236) -> (x+1=w237:dbl)
                      }
                    }
                    n164 = Multiply(x=w228, y=w231) -> (x*y=w232:dbl)
                    n165 = Divide(x=w232, y=60.0) -> (x/y=w227:dbl)
                    n166 = Bundle(cluster=w230, "CYCLE"=w228, "MINS"=w227) -> (w226:T4)  [unwired: 1 in]
                    n167 = local write "LAB05-2 (DISP)"(w226) -> ()
                  }
                }
                n168 = local write "jig cycle"(0) -> ()
              }
            }
          }
          frame #3 {
            # "START & STOP test RUN switch change, start test if true and stop test if false"
            n169 = Get Date/Time In Seconds() -> (seconds since 1Jan1904=w260:timestamp)
            n170 = Format Date/Time String(time format string (%c)="%Y%m%d", seconds (now)=w260) -> (date/time string=w261:string)  [unwired: 1 in]
            n171 = Format Date/Time String(time format string (%c)="%H%M", seconds (now)=w260) -> (date/time string=w258:string)  [unwired: 1 in]
            n172 = event shown="[1] \"LAB01-1RUN\": Value Change" {
              selector: _ -> [_ _ _ _ _ _ _ _ _ _ _]
              dyn-events: _ -> [_ _ _ _ _ _ _ _ _ _ _]
              timeout: 10 -> [_ _ _ _ _ _ _ _ _ _ _]
              tunnel: "c:\\crabtree\\Test Data\\" -> [_ w269 w347 w425 w503 w581 w659 w737 w815 w893 w971]
              tunnel: w261 -> [_ w268 w346 w424 w502 w580 w658 w736 w814 w892 w970]
              tunnel: w258 -> [_ w266 w345 w423 w501 w579 w657 w735 w813 w891 w969]
              tunnel: w256 -> [_ w267 _ _ _ _ _ _ _ _ _]
              tunnel: w257 -> [_ _ _ _ _ _ _ _ _ _ _]
              tunnel: w255 -> [_ _ w344 _ _ _ _ _ _ _ _]
              tunnel: w254 -> [_ _ w343 _ _ _ _ _ _ _ _]
              tunnel: w253 -> [_ _ _ w422 _ _ _ _ _ _ _]
              tunnel: w252 -> [_ _ _ w421 _ _ _ _ _ _ _]
              tunnel: w251 -> [_ _ _ _ w500 _ _ _ _ _ _]
              tunnel: w250 -> [_ _ _ _ w499 _ _ _ _ _ _]
              tunnel: w249 -> [_ _ _ _ _ w578 _ _ _ _ _]
              tunnel: w248 -> [_ _ _ _ _ w577 _ _ _ _ _]
              tunnel: w247 -> [_ _ _ _ _ _ w656 _ _ _ _]
              tunnel: w246 -> [_ _ _ _ _ _ w655 _ _ _ _]
              tunnel: w245 -> [_ _ _ _ _ _ _ w734 _ _ _]
              tunnel: w244 -> [_ _ _ _ _ _ _ w733 _ _ _]
              tunnel: w243 -> [_ _ _ _ _ _ _ _ w812 _ _]
              tunnel: w242 -> [_ _ _ _ _ _ _ _ w811 _ _]
              tunnel: w241 -> [_ _ _ _ _ _ _ _ _ w890 _]
              tunnel: w240 -> [_ _ _ _ _ _ _ _ _ w889 _]
              tunnel: w239 -> [_ _ _ _ _ _ _ _ _ _ w968]
              tunnel: w238 -> [_ _ _ _ _ _ _ _ _ _ w967]
              event Timeout {
                n173 = event-data() -> ()  [unwired: 1 in, 3 out]
              }
              event "LAB01-1RUN": Value Change {
                n174 = event-data() -> ("NewVal"=w265:bool)  [unwired: 1 in, 5 out]
                n175 = case shown="False" w265 {
                  tunnel: w269 -> [_ w291]
                  tunnel: w268 -> [_ w290]
                  tunnel: w267 -> [w270 w289]
                  tunnel: w266 -> [_ w288]
                  frame False {
                    # "stop test"
                    n176 = stacked-sequence {
                      tunnel: w270 -> [w276 _]
                      frame #0 {
                        n177 = local read "LAB01-1 (DISP)"() -> (w275:T4)
                        n178 = Unbundle(w275) -> ("CYCLE"=w273:dbl, "MINS"=w274:dbl)  [unwired: 1 out]
                        n179 = case shown="\"CYCLE TEST\"" w276 {
                          tunnel: w274 -> [_ _ w283]
                          tunnel: w273 -> [w281 w282 _]
                          tunnel: [w281 w282 w283] -> w272
                          frame "TEST SET UP", Default {
                          }
                          frame "CYCLE TEST" {
                          }
                          frame "T-RISE TEST" {
                          }
                        }
                        n180 = local read "LAB01-1 (TDMS)"() -> (w280:refnum<k34>)
                        n181 = Build Array("STOPPED") -> (w277:string[])
                        n182 = Build Array(w272) -> (w271:dbl[])
                        n183 = TDMS Write(0:w280, 5:"TEST RESULT", 7:w277, 9:w271) -> ()  [unwired: 2 in, 4 out]
                      }
                      frame #1 {
                        n184 = local read "LAB01-1 (DISP)"() -> (w287:T4)
                        n185 = Bundle(cluster=w287, "STATUS"="STOP") -> (w285:T4)  [unwired: 2 in]
                        n186 = local write "LAB01-1 (RESULT)"(FALSE) -> ()
                        n187 = local write "LAB01-1 (DISP)"(w285) -> ()
                      }
                    }
                  }
                  frame True {
                    # "start new test and create test file"
                    n188 = stacked-sequence {
                      seq-local: [w297 _ _ _ _] -> [_ w316 _ _ _]
                      tunnel: w291 -> [w306 _ _ _ _]
                      tunnel: w290 -> [w304 _ _ _ _]
                      tunnel: w289 -> [w303 _ _ _ _]
                      tunnel: w288 -> [w294 _ _ _ _]
                      frame #0 {
                        n189 = local read "LAB01-1 (SET)"() -> (w296:T5)
                        n190 = case shown="\"TEST SET UP\", Default" w303 {
                          tunnel: ["TEST SET UP-" "CYCLE TEST-" "T-RISE TEST-"] -> w299
                          frame "TEST SET UP", Default {
                          }
                          frame "CYCLE TEST" {
                          }
                          frame "T-RISE TEST" {
                          }
                        }
                        n191 = Unbundle(w296) -> ("DESCRIPTION"=w295:string)  [unwired: 4 out]
                        n192 = Concatenate Strings(w306, "LAB01-1\\", w304, "\\") -> (w300:string)
                        n193 = String To Path(string=w300) -> (path=w302:path)
                        n194 = Concatenate Strings(w300, w299, w295, "-", w294, ".tdms") -> (w297:string)
                        n195 = Create Folder(path (use dialog)=w302) -> (error out=w301:errorcluster)  [unwired: 2 in, 2 out]
                        n196 = call <vilib>:"Clear Errors.vi"("error in (no error)"=w301) -> ()  [unwired: 6 in, 1 out]
                      }
                      frame #1 {
                        n197 = String To Path(string=w316) -> (path=w310:path)
                        n198 = TDMS Open(5:FALSE, 6:FALSE, 10:T13."create or replace" ("operation (0:open)"), 11:w310) -> (0:w312:errorcluster, 3:→"LAB01-1 (TDMS)":refnum<k34>)  [unwired: 3 in]
                        n199 = local write "data file error"(w312) -> ()
                      }
                      frame #2 {
                        n200 = local read "LAB01-1 (SET)"() -> (w322:T5)
                        n201 = local read "LAB01-1 (TDMS)"() -> (w333:refnum<k34>)
                        n202 = Build Array("Testers Name", "Description", "Set Test Cycles", "T-Rise minutes", "T-Rise Deg C") -> (w323:string[])
                        n203 = Unbundle(w322) -> ("NAME"=w321:string, "DESCRIPTION"=w320:string, "CYCLES"=w319:dbl, "T-RISE mins"=w318:dbl, "T-RISE deg C"=w317:dbl)
                        n204 = Number To Decimal String(number=w319) -> (decimal integer string=w332:string)  [unwired: 1 in]
                        n205 = Number To Decimal String(number=w318) -> (decimal integer string=w331:string)  [unwired: 1 in]
                        n206 = Number To Decimal String(number=w317) -> (decimal integer string=w330:string)  [unwired: 1 in]
                        n207 = Build Array(w321, w320, w332, w331, w330) -> (w329:string[])
                        n208 = TDMS Set Properties(5:w329, 7:w323, 11:w333) -> ()  [unwired: 3 in, 4 out]
                      }
                      frame #3 {
                        w334 = 0.0
                        n209 = local read "LAB01-1 (DISP)"() -> (w337:T4)
                        n210 = Bundle(cluster=w337, "CYCLE"=w334, "MINS"=w334, "STATUS"="RUN") -> (w336:T4)
                        n211 = local write "LAB01-1 (FAIL LO)"(w334) -> ()
                        n212 = local write "LAB01-1 (FAIL HI)"(w334) -> ()
                        n213 = local write "LAB01-1 (DISP)"(w336) -> ()
                      }
                      frame #4 {
                        n214 = local read "LAB01-1 (SIG)"() -> (w340:T2)
                        n215 = local read "LAB01-1 (TEMP START)"() -> (w342:cluster{"TL":dbl, "TN":dbl})
                        n216 = Unbundle(w340) -> ("Tmp Live"=w339:dbl, "Tmp Neut"=w338:dbl)  [unwired: 3 out]
                        n217 = Bundle(cluster=w342, "TL"=w339, "TN"=w338) -> (w341:cluster{"TL":dbl, "TN":dbl})
                        n218 = local write "LAB01-1 (TEMP START)"(w341) -> ()
                      }
                    }
                  }
                }
              }
              event "LAB01-2 RUN": Value Change {
                n219 = event-data() -> ()  [unwired: 1 in, 6 out]
                n220 = case shown="True" w344 {
                  tunnel: w347 -> [_ w369]
                  tunnel: w346 -> [_ w368]
                  tunnel: w343 -> [w348 w367]
                  tunnel: w345 -> [_ w366]
                  frame False {
                    # "stop test"
                    n221 = stacked-sequence {
                      tunnel: w348 -> [w354 _]
                      frame #0 {
                        n222 = local read "LAB01-2 (DISP)"() -> (w353:T4)
                        n223 = Unbundle(w353) -> ("CYCLE"=w351:dbl, "MINS"=w352:dbl)  [unwired: 1 out]
                        n224 = case shown="\"CYCLE TEST\"" w354 {
                          tunnel: w352 -> [_ _ w361]
                          tunnel: w351 -> [w359 w360 _]
                          tunnel: [w359 w360 w361] -> w350
                          frame "TEST SET UP", Default {
                          }
                          frame "CYCLE TEST" {
                          }
                          frame "T-RISE TEST" {
                          }
                        }
                        n225 = local read "LAB01-2 (TDMS)"() -> (w358:refnum<k34>)
                        n226 = Build Array("STOPPED") -> (w355:string[])
                        n227 = Build Array(w350) -> (w349:dbl[])
                        n228 = TDMS Write(0:w358, 5:"TEST RESULT", 7:w355, 9:w349) -> ()  [unwired: 2 in, 4 out]
                      }
                      frame #1 {
                        n229 = local read "LAB01-2 (DISP)"() -> (w365:T4)
                        n230 = Bundle(cluster=w365, "STATUS"="STOP") -> (w363:T4)  [unwired: 2 in]
                        n231 = local write "LAB01-2 (RESULT)"(FALSE) -> ()
                        n232 = local write "LAB01-2 (DISP)"(w363) -> ()
                      }
                    }
                  }
                  frame True {
                    # "start new test and create test file"
                    n233 = stacked-sequence {
                      seq-local: [w375 _ _ _ _] -> [_ w394 _ _ _]
                      tunnel: w369 -> [w384 _ _ _ _]
                      tunnel: w368 -> [w382 _ _ _ _]
                      tunnel: w367 -> [w381 _ _ _ _]
                      tunnel: w366 -> [w372 _ _ _ _]
                      frame #0 {
                        n234 = local read "LAB01-2(SET)"() -> (w374:T5)
                        n235 = case shown="\"TEST SET UP\", Default" w381 {
                          tunnel: ["TEST SET UP-" "CYCLE TEST-" "T-RISE TEST-"] -> w377
                          frame "TEST SET UP", Default {
                          }
                          frame "CYCLE TEST" {
                          }
                          frame "T-RISE TEST" {
                          }
                        }
                        n236 = Unbundle(w374) -> ("DESCRIPTION"=w373:string)  [unwired: 4 out]
                        n237 = Concatenate Strings(w384, "LAB01-2\\", w382, "\\") -> (w378:string)
                        n238 = String To Path(string=w378) -> (path=w380:path)
                        n239 = Concatenate Strings(w378, w377, w373, "-", w372, ".tdms") -> (w375:string)
                        n240 = Create Folder(path (use dialog)=w380) -> (error out=w379:errorcluster)  [unwired: 2 in, 2 out]
                        n241 = call <vilib>:"Clear Errors.vi"("error in (no error)"=w379) -> ()  [unwired: 6 in, 1 out]
                      }
                      frame #1 {
                        n242 = String To Path(string=w394) -> (path=w388:path)
                        n243 = TDMS Open(5:FALSE, 6:FALSE, 10:T13."create or replace" ("operation (0:open)"), 11:w388) -> (0:w390:errorcluster, 3:→"LAB01-2 (TDMS)":refnum<k34>)  [unwired: 3 in]
                        n244 = local write "data file error"(w390) -> ()
                      }
                      frame #2 {
                        n245 = local read "LAB01-2(SET)"() -> (w400:T5)
                        n246 = local read "LAB01-2 (TDMS)"() -> (w411:refnum<k34>)
                        n247 = Build Array("Testers Name", "Description", "Set Test Cycles", "T-Rise minutes", "T-Rise Deg C") -> (w401:string[])
                        n248 = Unbundle(w400) -> ("NAME"=w399:string, "DESCRIPTION"=w398:string, "CYCLES"=w397:dbl, "T-RISE mins"=w396:dbl, "T-RISE deg C"=w395:dbl)
                        n249 = Number To Decimal String(number=w397) -> (decimal integer string=w410:string)  [unwired: 1 in]
                        n250 = Number To Decimal String(number=w396) -> (decimal integer string=w409:string)  [unwired: 1 in]
                        n251 = Number To Decimal String(number=w395) -> (decimal integer string=w408:string)  [unwired: 1 in]
                        n252 = Build Array(w399, w398, w410, w409, w408) -> (w407:string[])
                        n253 = TDMS Set Properties(5:w407, 7:w401, 11:w411) -> ()  [unwired: 3 in, 4 out]
                      }
                      frame #3 {
                        w413 = 0.0
                        n254 = local read "LAB01-2 (DISP)"() -> (w415:T4)
                        n255 = Bundle(cluster=w415, "CYCLE"=w413, "MINS"=w413, "STATUS"="RUN") -> (w414:T4)
                        n256 = local write "LAB01-2 (DISP)"(w414) -> ()
                      }
                      frame #4 {
                        n257 = local read "LAB01-2 (SIG)"() -> (w418:T2)
                        n258 = local read "LAB01-2 (TEMP START)"() -> (w420:cluster{"TL":dbl, "TN":dbl})
                        n259 = Unbundle(w418) -> ("Tmp Live"=w417:dbl, "Tmp Neut"=w416:dbl)  [unwired: 3 out]
                        n260 = Bundle(cluster=w420, "TL"=w417, "TN"=w416) -> (w419:cluster{"TL":dbl, "TN":dbl})
                        n261 = local write "LAB01-2 (TEMP START)"(w419) -> ()
                      }
                    }
                  }
                }
              }
              event "LAB02-1 RUN": Value Change {
                n262 = event-data() -> ()  [unwired: 1 in, 6 out]
                n263 = case shown="True" w422 {
                  tunnel: w425 -> [_ w447]
                  tunnel: w424 -> [_ w446]
                  tunnel: w421 -> [w426 w445]
                  tunnel: w423 -> [_ w444]
                  frame False {
                    # "stop test"
                    n264 = stacked-sequence {
                      tunnel: w426 -> [w432 _]
                      frame #0 {
                        n265 = local read "LAB02-1 (DISP)"() -> (w431:T4)
                        n266 = Unbundle(w431) -> ("CYCLE"=w429:dbl, "MINS"=w430:dbl)  [unwired: 1 out]
                        n267 = case shown="\"CYCLE TEST\"" w432 {
                          tunnel: w430 -> [_ _ w439]
                          tunnel: w429 -> [w437 w438 _]
                          tunnel: [w437 w438 w439] -> w428
                          frame "TEST SET UP", Default {
                          }
                          frame "CYCLE TEST" {
                          }
                          frame "T-RISE TEST" {
                          }
                        }
                        n268 = local read "LAB02-1 (TDMS)"() -> (w436:refnum<k34>)
                        n269 = Build Array("STOPPED") -> (w433:string[])
                        n270 = Build Array(w428) -> (w427:dbl[])
                        n271 = TDMS Write(0:w436, 5:"TEST RESULT", 7:w433, 9:w427) -> ()  [unwired: 2 in, 4 out]
                      }
                      frame #1 {
                        n272 = local read "LAB02-1 (DISP)"() -> (w443:T4)
                        n273 = Bundle(cluster=w443, "STATUS"="STOPPED") -> (w441:T4)  [unwired: 2 in]
                        n274 = local write "LAB02-1 (RESULT)"(FALSE) -> ()
                        n275 = local write "LAB02-1 (DISP)"(w441) -> ()
                      }
                    }
                  }
                  frame True {
                    # "start new test and create test file"
                    n276 = stacked-sequence {
                      seq-local: [w453 _ _ _ _] -> [_ w472 _ _ _]
                      tunnel: w447 -> [w462 _ _ _ _]
                      tunnel: w446 -> [w460 _ _ _ _]
                      tunnel: w445 -> [w459 _ _ _ _]
                      tunnel: w444 -> [w450 _ _ _ _]
                      frame #0 {
                        n277 = local read "LAB02-1 (SET)"() -> (w452:T5)
                        n278 = case shown="\"TEST SET UP\", Default" w459 {
                          tunnel: ["TEST SET UP-" "CYCLE TEST-" "T-RISE TEST-"] -> w455
                          frame "TEST SET UP", Default {
                          }
                          frame "CYCLE TEST" {
                          }
                          frame "T-RISE TEST" {
                          }
                        }
                        n279 = Unbundle(w452) -> ("DESCRIPTION"=w451:string)  [unwired: 4 out]
                        n280 = Concatenate Strings(w462, "LAB02-1\\", w460, "\\") -> (w456:string)
                        n281 = String To Path(string=w456) -> (path=w458:path)
                        n282 = Concatenate Strings(w456, w455, w451, "-", w450, ".tdms") -> (w453:string)
                        n283 = Create Folder(path (use dialog)=w458) -> (error out=w457:errorcluster)  [unwired: 2 in, 2 out]
                        n284 = call <vilib>:"Clear Errors.vi"("error in (no error)"=w457) -> ()  [unwired: 6 in, 1 out]
                      }
                      frame #1 {
                        n285 = String To Path(string=w472) -> (path=w466:path)
                        n286 = TDMS Open(5:FALSE, 6:FALSE, 10:T13."create or replace" ("operation (0:open)"), 11:w466) -> (0:w468:errorcluster, 3:→"LAB02-1 (TDMS)":refnum<k34>)  [unwired: 3 in]
                        n287 = local write "data file error"(w468) -> ()
                      }
                      frame #2 {
                        n288 = local read "LAB02-1 (SET)"() -> (w478:T5)
                        n289 = local read "LAB02-1 (TDMS)"() -> (w489:refnum<k34>)
                        n290 = Build Array("Testers Name", "Description", "Set Test Cycles", "T-Rise minutes", "T-Rise Deg C") -> (w479:string[])
                        n291 = Unbundle(w478) -> ("NAME"=w477:string, "DESCRIPTION"=w476:string, "CYCLES"=w475:dbl, "T-RISE mins"=w474:dbl, "T-RISE deg C"=w473:dbl)
                        n292 = Number To Decimal String(number=w475) -> (decimal integer string=w488:string)  [unwired: 1 in]
                        n293 = Number To Decimal String(number=w474) -> (decimal integer string=w487:string)  [unwired: 1 in]
                        n294 = Number To Decimal String(number=w473) -> (decimal integer string=w486:string)  [unwired: 1 in]
                        n295 = Build Array(w477, w476, w488, w487, w486) -> (w485:string[])
                        n296 = TDMS Set Properties(5:w485, 7:w479, 11:w489) -> ()  [unwired: 3 in, 4 out]
                      }
                      frame #3 {
                        w491 = 0.0
                        n297 = local read "LAB02-1 (DISP)"() -> (w493:T4)
                        n298 = Bundle(cluster=w493, "CYCLE"=w491, "MINS"=w491, "STATUS"="RUN") -> (w492:T4)
                        n299 = local write "LAB02-1 (DISP)"(w492) -> ()
                      }
                      frame #4 {
                        n300 = local read "LAB02-1 (SIG)"() -> (w496:T2)
                        n301 = local read "LAB02-1 (TEMP START)"() -> (w498:cluster{"TL":dbl, "TN":dbl})
                        n302 = Unbundle(w496) -> ("Tmp Live"=w495:dbl, "Tmp Neut"=w494:dbl)  [unwired: 3 out]
                        n303 = Bundle(cluster=w498, "TL"=w495, "TN"=w494) -> (w497:cluster{"TL":dbl, "TN":dbl})
                        n304 = local write "LAB02-1 (TEMP START)"(w497) -> ()
                      }
                    }
                  }
                }
              }
              event "LAB02-2 RUN": Value Change {
                n305 = event-data() -> ()  [unwired: 1 in, 6 out]
                n306 = case shown="True" w500 {
                  tunnel: w503 -> [_ w525]
                  tunnel: w502 -> [_ w524]
                  tunnel: w499 -> [w504 w523]
                  tunnel: w501 -> [_ w522]
                  frame False {
                    # "stop test"
                    n307 = stacked-sequence {
                      tunnel: w504 -> [w510 _]
                      frame #0 {
                        n308 = local read "LAB02-2 (DISP)"() -> (w509:T4)
                        n309 = Unbundle(w509) -> ("CYCLE"=w507:dbl, "MINS"=w508:dbl)  [unwired: 1 out]
                        n310 = case shown="\"CYCLE TEST\"" w510 {
                          tunnel: w508 -> [_ _ w517]
                          tunnel: w507 -> [w515 w516 _]
                          tunnel: [w515 w516 w517] -> w506
                          frame "TEST SET UP", Default {
                          }
                          frame "CYCLE TEST" {
                          }
                          frame "T-RISE TEST" {
                          }
                        }
                        n311 = local read "LAB02-2 (TDMS)"() -> (w514:refnum<k34>)
                        n312 = Build Array("STOPPED") -> (w511:string[])
                        n313 = Build Array(w506) -> (w505:dbl[])
                        n314 = TDMS Write(0:w514, 5:"TEST RESULT", 7:w511, 9:w505) -> ()  [unwired: 2 in, 4 out]
                      }
                      frame #1 {
                        n315 = local read "LAB02-2 (DISP)"() -> (w521:T4)
                        n316 = Bundle(cluster=w521, "STATUS"="STOP") -> (w519:T4)  [unwired: 2 in]
                        n317 = local write "LAB02-2 (RESULT)"(FALSE) -> ()
                        n318 = local write "LAB02-2 (DISP)"(w519) -> ()
                      }
                    }
                  }
                  frame True {
                    # "start new test and create test file"
                    n319 = stacked-sequence {
                      seq-local: [w531 _ _ _ _] -> [_ w550 _ _ _]
                      tunnel: w525 -> [w540 _ _ _ _]
                      tunnel: w524 -> [w538 _ _ _ _]
                      tunnel: w523 -> [w537 _ _ _ _]
                      tunnel: w522 -> [w528 _ _ _ _]
                      frame #0 {
                        n320 = local read "LAB02-2 (SET)"() -> (w530:T5)
                        n321 = case shown="\"TEST SET UP\", Default" w537 {
                          tunnel: ["TEST SET UP-" "CYCLE TEST-" "T-RISE TEST-"] -> w533
                          frame "TEST SET UP", Default {
                          }
                          frame "CYCLE TEST" {
                          }
                          frame "T-RISE TEST" {
                          }
                        }
                        n322 = Unbundle(w530) -> ("DESCRIPTION"=w529:string)  [unwired: 4 out]
                        n323 = Concatenate Strings(w540, "LAB02-2\\", w538, "\\") -> (w534:string)
                        n324 = String To Path(string=w534) -> (path=w536:path)
                        n325 = Concatenate Strings(w534, w533, w529, "-", w528, ".tdms") -> (w531:string)
                        n326 = Create Folder(path (use dialog)=w536) -> (error out=w535:errorcluster)  [unwired: 2 in, 2 out]
                        n327 = call <vilib>:"Clear Errors.vi"("error in (no error)"=w535) -> ()  [unwired: 6 in, 1 out]
                      }
                      frame #1 {
                        n328 = String To Path(string=w550) -> (path=w544:path)
                        n329 = TDMS Open(5:FALSE, 6:FALSE, 10:T13."create or replace" ("operation (0:open)"), 11:w544) -> (0:w546:errorcluster, 3:→"LAB02-2 (TDMS)":refnum<k34>)  [unwired: 3 in]
                        n330 = local write "data file error"(w546) -> ()
                      }
                      frame #2 {
                        n331 = local read "LAB02-2 (SET)"() -> (w556:T5)
                        n332 = local read "LAB02-2 (TDMS)"() -> (w567:refnum<k34>)
                        n333 = Build Array("Testers Name", "Description", "Set Test Cycles", "T-Rise minutes", "T-Rise Deg C") -> (w557:string[])
                        n334 = Unbundle(w556) -> ("NAME"=w555:string, "DESCRIPTION"=w554:string, "CYCLES"=w553:dbl, "T-RISE mins"=w552:dbl, "T-RISE deg C"=w551:dbl)
                        n335 = Number To Decimal String(number=w553) -> (decimal integer string=w566:string)  [unwired: 1 in]
                        n336 = Number To Decimal String(number=w552) -> (decimal integer string=w565:string)  [unwired: 1 in]
                        n337 = Number To Decimal String(number=w551) -> (decimal integer string=w564:string)  [unwired: 1 in]
                        n338 = Build Array(w555, w554, w566, w565, w564) -> (w563:string[])
                        n339 = TDMS Set Properties(5:w563, 7:w557, 11:w567) -> ()  [unwired: 3 in, 4 out]
                      }
                      frame #3 {
                        w569 = 0.0
                        n340 = local read "LAB02-2 (DISP)"() -> (w571:T4)
                        n341 = Bundle(cluster=w571, "CYCLE"=w569, "MINS"=w569, "STATUS"="RUN") -> (w570:T4)
                        n342 = local write "LAB02-2 (DISP)"(w570) -> ()
                      }
                      frame #4 {
                        n343 = local read "LAB02-2 (SIG)"() -> (w574:T2)
                        n344 = local read "LAB02-2 (TEMP START)"() -> (w576:cluster{"TL":dbl, "TN":dbl})
                        n345 = Unbundle(w574) -> ("Tmp Live"=w573:dbl, "Tmp Neut"=w572:dbl)  [unwired: 3 out]
                        n346 = Bundle(cluster=w576, "TL"=w573, "TN"=w572) -> (w575:cluster{"TL":dbl, "TN":dbl})
                        n347 = local write "LAB02-2 (TEMP START)"(w575) -> ()
                      }
                    }
                  }
                }
              }
              event "LAB03-1 RUN": Value Change {
                n348 = event-data() -> ()  [unwired: 1 in, 6 out]
                n349 = case shown="True" w578 {
                  tunnel: w581 -> [_ w603]
                  tunnel: w580 -> [_ w602]
                  tunnel: w577 -> [w582 w601]
                  tunnel: w579 -> [_ w600]
                  frame False {
                    # "stop test"
                    n350 = stacked-sequence {
                      tunnel: w582 -> [w588 _]
                      frame #0 {
                        n351 = local read "LAB03-1 (DISP)"() -> (w587:T4)
                        n352 = Unbundle(w587) -> ("CYCLE"=w585:dbl, "MINS"=w586:dbl)  [unwired: 1 out]
                        n353 = case shown="\"CYCLE TEST\"" w588 {
                          tunnel: w586 -> [_ _ w595]
                          tunnel: w585 -> [w593 w594 _]
                          tunnel: [w593 w594 w595] -> w584
                          frame "TEST SET UP", Default {
                          }
                          frame "CYCLE TEST" {
                          }
                          frame "T-RISE TEST" {
                          }
                        }
                        n354 = local read "LAB03-1 (TDMS)"() -> (w592:refnum<k34>)
                        n355 = Build Array("STOPPED") -> (w589:string[])
                        n356 = Build Array(w584) -> (w583:dbl[])
                        n357 = TDMS Write(0:w592, 5:"TEST RESULT", 7:w589, 9:w583) -> ()  [unwired: 2 in, 4 out]
                      }
                      frame #1 {
                        n358 = local read "LAB03-1 (DISP)"() -> (w599:T4)
                        n359 = Bundle(cluster=w599, "STATUS"="STOP") -> (w597:T4)  [unwired: 2 in]
                        n360 = local write "LAB03-1 (RESULT)"(FALSE) -> ()
                        n361 = local write "LAB03-1 (DISP)"(w597) -> ()
                      }
                    }
                  }
                  frame True {
                    # "start new test and create test file"
                    n362 = stacked-sequence {
                      seq-local: [w609 _ _ _ _] -> [_ w628 _ _ _]
                      tunnel: w603 -> [w618 _ _ _ _]
                      tunnel: w602 -> [w616 _ _ _ _]
                      tunnel: w601 -> [w615 _ _ _ _]
                      tunnel: w600 -> [w606 _ _ _ _]
                      frame #0 {
                        n363 = local read "LAB03-1 (SET)"() -> (w608:T5)
                        n364 = case shown="\"TEST SET UP\", Default" w615 {
                          tunnel: ["TEST SET UP-" "CYCLE TEST-" "T-RISE TEST-"] -> w611
                          frame "TEST SET UP", Default {
                          }
                          frame "CYCLE TEST" {
                          }
                          frame "T-RISE TEST" {
                          }
                        }
                        n365 = Unbundle(w608) -> ("DESCRIPTION"=w607:string)  [unwired: 4 out]
                        n366 = Concatenate Strings(w618, "LAB03-1\\", w616, "\\") -> (w612:string)
                        n367 = String To Path(string=w612) -> (path=w614:path)
                        n368 = Concatenate Strings(w612, w611, w607, "-", w606, ".tdms") -> (w609:string)
                        n369 = Create Folder(path (use dialog)=w614) -> (error out=w613:errorcluster)  [unwired: 2 in, 2 out]
                        n370 = call <vilib>:"Clear Errors.vi"("error in (no error)"=w613) -> ()  [unwired: 6 in, 1 out]
                      }
                      frame #1 {
                        n371 = String To Path(string=w628) -> (path=w622:path)
                        n372 = TDMS Open(5:FALSE, 6:FALSE, 10:T13."create or replace" ("operation (0:open)"), 11:w622) -> (0:w624:errorcluster, 3:→"LAB03-1 (TDMS)":refnum<k34>)  [unwired: 3 in]
                        n373 = local write "data file error"(w624) -> ()
                      }
                      frame #2 {
                        n374 = local read "LAB03-1 (SET)"() -> (w634:T5)
                        n375 = local read "LAB03-1 (TDMS)"() -> (w645:refnum<k34>)
                        n376 = Build Array("Testers Name", "Description", "Set Test Cycles", "T-Rise minutes", "T-Rise Deg C") -> (w635:string[])
                        n377 = Unbundle(w634) -> ("NAME"=w633:string, "DESCRIPTION"=w632:string, "CYCLES"=w631:dbl, "T-RISE mins"=w630:dbl, "T-RISE deg C"=w629:dbl)
                        n378 = Number To Decimal String(number=w631) -> (decimal integer string=w644:string)  [unwired: 1 in]
                        n379 = Number To Decimal String(number=w630) -> (decimal integer string=w643:string)  [unwired: 1 in]
                        n380 = Number To Decimal String(number=w629) -> (decimal integer string=w642:string)  [unwired: 1 in]
                        n381 = Build Array(w633, w632, w644, w643, w642) -> (w641:string[])
                        n382 = TDMS Set Properties(5:w641, 7:w635, 11:w645) -> ()  [unwired: 3 in, 4 out]
                      }
                      frame #3 {
                        w647 = 0.0
                        n383 = local read "LAB03-1 (DISP)"() -> (w649:T4)
                        n384 = Bundle(cluster=w649, "CYCLE"=w647, "MINS"=w647, "STATUS"="RUN") -> (w648:T4)
                        n385 = local write "LAB03-1 (DISP)"(w648) -> ()
                      }
                      frame #4 {
                        n386 = local read "LAB03-1 (SIG)"() -> (w652:T2)
                        n387 = local read "LAB03-1 (TEMP START)"() -> (w654:cluster{"TL":dbl, "TN":dbl})
                        n388 = Unbundle(w652) -> ("Tmp Live"=w651:dbl, "Tmp Neut"=w650:dbl)  [unwired: 3 out]
                        n389 = Bundle(cluster=w654, "TL"=w651, "TN"=w650) -> (w653:cluster{"TL":dbl, "TN":dbl})
                        n390 = local write "LAB03-1 (TEMP START)"(w653) -> ()
                      }
                    }
                  }
                }
              }
              event "LAB03-2 RUN": Value Change {
                n391 = event-data() -> ()  [unwired: 1 in, 6 out]
                n392 = case shown="True" w656 {
                  tunnel: w659 -> [_ w681]
                  tunnel: w658 -> [_ w680]
                  tunnel: w655 -> [w660 w679]
                  tunnel: w657 -> [_ w678]
                  frame False {
                    # "stop test"
                    n393 = stacked-sequence {
                      tunnel: w660 -> [w666 _]
                      frame #0 {
                        n394 = local read "LAB03-2 (DISP)"() -> (w665:T4)
                        n395 = Unbundle(w665) -> ("CYCLE"=w663:dbl, "MINS"=w664:dbl)  [unwired: 1 out]
                        n396 = case shown="\"CYCLE TEST\"" w666 {
                          tunnel: w664 -> [_ _ w673]
                          tunnel: w663 -> [w671 w672 _]
                          tunnel: [w671 w672 w673] -> w662
                          frame "TEST SET UP", Default {
                          }
                          frame "CYCLE TEST" {
                          }
                          frame "T-RISE TEST" {
                          }
                        }
                        n397 = local read "LAB03-2 (TDMS)"() -> (w670:refnum<k34>)
                        n398 = Build Array("STOPPED") -> (w667:string[])
                        n399 = Build Array(w662) -> (w661:dbl[])
                        n400 = TDMS Write(0:w670, 5:"TEST RESULT", 7:w667, 9:w661) -> ()  [unwired: 2 in, 4 out]
                      }
                      frame #1 {
                        n401 = local read "LAB03-2 (DISP)"() -> (w677:T4)
                        n402 = Bundle(cluster=w677, "STATUS"="STOP") -> (w675:T4)  [unwired: 2 in]
                        n403 = local write "LAB03-2 (RESULT)"(FALSE) -> ()
                        n404 = local write "LAB03-2 (DISP)"(w675) -> ()
                      }
                    }
                  }
                  frame True {
                    # "start new test and create test file"
                    n405 = stacked-sequence {
                      seq-local: [w687 _ _ _ _] -> [_ w706 _ _ _]
                      tunnel: w681 -> [w696 _ _ _ _]
                      tunnel: w680 -> [w694 _ _ _ _]
                      tunnel: w679 -> [w693 _ _ _ _]
                      tunnel: w678 -> [w684 _ _ _ _]
                      frame #0 {
                        n406 = local read "LAB03-2 (SET)"() -> (w686:T5)
                        n407 = case shown="\"TEST SET UP\", Default" w693 {
                          tunnel: ["TEST SET UP-" "CYCLE TEST-" "T-RISE TEST-"] -> w689
                          frame "TEST SET UP", Default {
                          }
                          frame "CYCLE TEST" {
                          }
                          frame "T-RISE TEST" {
                          }
                        }
                        n408 = Unbundle(w686) -> ("DESCRIPTION"=w685:string)  [unwired: 4 out]
                        n409 = Concatenate Strings(w696, "LAB03-2\\", w694, "\\") -> (w690:string)
                        n410 = String To Path(string=w690) -> (path=w692:path)
                        n411 = Concatenate Strings(w690, w689, w685, "-", w684, ".tdms") -> (w687:string)
                        n412 = Create Folder(path (use dialog)=w692) -> (error out=w691:errorcluster)  [unwired: 2 in, 2 out]
                        n413 = call <vilib>:"Clear Errors.vi"("error in (no error)"=w691) -> ()  [unwired: 6 in, 1 out]
                      }
                      frame #1 {
                        n414 = String To Path(string=w706) -> (path=w700:path)
                        n415 = TDMS Open(5:FALSE, 6:FALSE, 10:T13."create or replace" ("operation (0:open)"), 11:w700) -> (0:w702:errorcluster, 3:→"LAB03-2 (TDMS)":refnum<k34>)  [unwired: 3 in]
                        n416 = local write "data file error"(w702) -> ()
                      }
                      frame #2 {
                        n417 = local read "LAB03-2 (SET)"() -> (w712:T5)
                        n418 = local read "LAB03-2 (TDMS)"() -> (w723:refnum<k34>)
                        n419 = Build Array("Testers Name", "Description", "Set Test Cycles", "T-Rise minutes", "T-Rise Deg C") -> (w713:string[])
                        n420 = Unbundle(w712) -> ("NAME"=w711:string, "DESCRIPTION"=w710:string, "CYCLES"=w709:dbl, "T-RISE mins"=w708:dbl, "T-RISE deg C"=w707:dbl)
                        n421 = Number To Decimal String(number=w709) -> (decimal integer string=w722:string)  [unwired: 1 in]
                        n422 = Number To Decimal String(number=w708) -> (decimal integer string=w721:string)  [unwired: 1 in]
                        n423 = Number To Decimal String(number=w707) -> (decimal integer string=w720:string)  [unwired: 1 in]
                        n424 = Build Array(w711, w710, w722, w721, w720) -> (w719:string[])
                        n425 = TDMS Set Properties(5:w719, 7:w713, 11:w723) -> ()  [unwired: 3 in, 4 out]
                      }
                      frame #3 {
                        w725 = 0.0
                        n426 = local read "LAB03-2 (DISP)"() -> (w727:T4)
                        n427 = Bundle(cluster=w727, "CYCLE"=w725, "MINS"=w725, "STATUS"="RUN") -> (w726:T4)
                        n428 = local write "LAB03-2 (DISP)"(w726) -> ()
                      }
                      frame #4 {
                        n429 = local read "LAB03-2 (SIG)"() -> (w730:T2)
                        n430 = local read "LAB03-2 (TEMP START)"() -> (w732:cluster{"TL":dbl, "TN":dbl})
                        n431 = Unbundle(w730) -> ("Tmp Live"=w729:dbl, "Tmp Neut"=w728:dbl)  [unwired: 3 out]
                        n432 = Bundle(cluster=w732, "TL"=w729, "TN"=w728) -> (w731:cluster{"TL":dbl, "TN":dbl})
                        n433 = local write "LAB03-2 (TEMP START)"(w731) -> ()
                      }
                    }
                  }
                }
              }
              event "LAB04-1 RUN": Value Change {
                n434 = event-data() -> ()  [unwired: 1 in, 6 out]
                n435 = case shown="True" w734 {
                  tunnel: w737 -> [_ w759]
                  tunnel: w736 -> [_ w758]
                  tunnel: w733 -> [w738 w757]
                  tunnel: w735 -> [_ w756]
                  frame False {
                    # "stop test"
                    n436 = stacked-sequence {
                      tunnel: w738 -> [w744 _]
                      frame #0 {
                        n437 = local read "LAB04-1 (DISP)"() -> (w743:T4)
                        n438 = Unbundle(w743) -> ("CYCLE"=w741:dbl, "MINS"=w742:dbl)  [unwired: 1 out]
                        n439 = case shown="\"CYCLE TEST\"" w744 {
                          tunnel: w742 -> [_ _ w751]
                          tunnel: w741 -> [w749 w750 _]
                          tunnel: [w749 w750 w751] -> w740
                          frame "TEST SET UP", Default {
                          }
                          frame "CYCLE TEST" {
                          }
                          frame "T-RISE TEST" {
                          }
                        }
                        n440 = local read "LAB04-1 (TDMS)"() -> (w748:refnum<k34>)
                        n441 = Build Array("STOPPED") -> (w745:string[])
                        n442 = Build Array(w740) -> (w739:dbl[])
                        n443 = TDMS Write(0:w748, 5:"TEST RESULT", 7:w745, 9:w739) -> ()  [unwired: 2 in, 4 out]
                      }
                      frame #1 {
                        n444 = local read "LAB04-1 (DISP)"() -> (w755:T4)
                        n445 = Bundle(cluster=w755, "STATUS"="STOP") -> (w753:T4)  [unwired: 2 in]
                        n446 = local write "LAB04-1 (RESULT)"(FALSE) -> ()
                        n447 = local write "LAB04-1 (DISP)"(w753) -> ()
                      }
                    }
                  }
                  frame True {
                    # "start new test and create test file"
                    n448 = stacked-sequence {
                      seq-local: [w765 _ _ _ _] -> [_ w784 _ _ _]
                      tunnel: w759 -> [w774 _ _ _ _]
                      tunnel: w758 -> [w772 _ _ _ _]
                      tunnel: w757 -> [w771 _ _ _ _]
                      tunnel: w756 -> [w762 _ _ _ _]
                      frame #0 {
                        n449 = local read "LAB04-1 (SET)"() -> (w764:T5)
                        n450 = case shown="\"TEST SET UP\", Default" w771 {
                          tunnel: ["TEST SET UP-" "CYCLE TEST-" "T-RISE TEST-"] -> w767
                          frame "TEST SET UP", Default {
                          }
                          frame "CYCLE TEST" {
                          }
                          frame "T-RISE TEST" {
                          }
                        }
                        n451 = Unbundle(w764) -> ("DESCRIPTION"=w763:string)  [unwired: 4 out]
                        n452 = Concatenate Strings(w774, "LAB04-1\\", w772, "\\") -> (w768:string)
                        n453 = String To Path(string=w768) -> (path=w770:path)
                        n454 = Concatenate Strings(w768, w767, w763, "-", w762, ".tdms") -> (w765:string)
                        n455 = Create Folder(path (use dialog)=w770) -> (error out=w769:errorcluster)  [unwired: 2 in, 2 out]
                        n456 = call <vilib>:"Clear Errors.vi"("error in (no error)"=w769) -> ()  [unwired: 6 in, 1 out]
                      }
                      frame #1 {
                        n457 = String To Path(string=w784) -> (path=w778:path)
                        n458 = TDMS Open(5:FALSE, 6:FALSE, 10:T13."create or replace" ("operation (0:open)"), 11:w778) -> (0:w780:errorcluster, 3:→"LAB04-1 (TDMS)":refnum<k34>)  [unwired: 3 in]
                        n459 = local write "data file error"(w780) -> ()
                      }
                      frame #2 {
                        n460 = local read "LAB04-1 (SET)"() -> (w790:T5)
                        n461 = local read "LAB04-1 (TDMS)"() -> (w801:refnum<k34>)
                        n462 = Build Array("Testers Name", "Description", "Set Test Cycles", "T-Rise minutes", "T-Rise Deg C") -> (w791:string[])
                        n463 = Unbundle(w790) -> ("NAME"=w789:string, "DESCRIPTION"=w788:string, "CYCLES"=w787:dbl, "T-RISE mins"=w786:dbl, "T-RISE deg C"=w785:dbl)
                        n464 = Number To Decimal String(number=w787) -> (decimal integer string=w800:string)  [unwired: 1 in]
                        n465 = Number To Decimal String(number=w786) -> (decimal integer string=w799:string)  [unwired: 1 in]
                        n466 = Number To Decimal String(number=w785) -> (decimal integer string=w798:string)  [unwired: 1 in]
                        n467 = Build Array(w789, w788, w800, w799, w798) -> (w797:string[])
                        n468 = TDMS Set Properties(5:w797, 7:w791, 11:w801) -> ()  [unwired: 3 in, 4 out]
                      }
                      frame #3 {
                        w803 = 0.0
                        n469 = local read "LAB04-1 (DISP)"() -> (w805:T4)
                        n470 = Bundle(cluster=w805, "CYCLE"=w803, "MINS"=w803, "STATUS"="RUN") -> (w804:T4)
                        n471 = local write "LAB04-1 (DISP)"(w804) -> ()
                      }
                      frame #4 {
                        n472 = local read "LAB04-1 (SIG)"() -> (w808:T2)
                        n473 = local read "LAB04-1 (TEMP START)"() -> (w810:cluster{"TL":dbl, "TN":dbl})
                        n474 = Unbundle(w808) -> ("Tmp Live"=w807:dbl, "Tmp Neut"=w806:dbl)  [unwired: 3 out]
                        n475 = Bundle(cluster=w810, "TL"=w807, "TN"=w806) -> (w809:cluster{"TL":dbl, "TN":dbl})
                        n476 = local write "LAB04-1 (TEMP START)"(w809) -> ()
                      }
                    }
                  }
                }
              }
              event "LAB04-2 RUN": Value Change {
                n477 = event-data() -> ()  [unwired: 1 in, 6 out]
                n478 = case shown="True" w812 {
                  tunnel: w815 -> [_ w837]
                  tunnel: w814 -> [_ w836]
                  tunnel: w811 -> [w816 w835]
                  tunnel: w813 -> [_ w834]
                  frame False {
                    # "stop test"
                    n479 = stacked-sequence {
                      tunnel: w816 -> [w822 _]
                      frame #0 {
                        n480 = local read "LAB04-2 (DISP)"() -> (w821:T4)
                        n481 = Unbundle(w821) -> ("CYCLE"=w819:dbl, "MINS"=w820:dbl)  [unwired: 1 out]
                        n482 = case shown="\"CYCLE TEST\"" w822 {
                          tunnel: w820 -> [_ _ w829]
                          tunnel: w819 -> [w827 w828 _]
                          tunnel: [w827 w828 w829] -> w818
                          frame "TEST SET UP", Default {
                          }
                          frame "CYCLE TEST" {
                          }
                          frame "T-RISE TEST" {
                          }
                        }
                        n483 = local read "LAB04-2 (TDMS)"() -> (w826:refnum<k34>)
                        n484 = Build Array("STOPPED") -> (w823:string[])
                        n485 = Build Array(w818) -> (w817:dbl[])
                        n486 = TDMS Write(0:w826, 5:"TEST RESULT", 7:w823, 9:w817) -> ()  [unwired: 2 in, 4 out]
                      }
                      frame #1 {
                        n487 = local read "LAB04-2 (DISP)"() -> (w833:T4)
                        n488 = Bundle(cluster=w833, "STATUS"="STOP") -> (w831:T4)  [unwired: 2 in]
                        n489 = local write "LAB04-2 (RESULT)"(FALSE) -> ()
                        n490 = local write "LAB04-2 (DISP)"(w831) -> ()
                      }
                    }
                  }
                  frame True {
                    # "start new test and create test file"
                    n491 = stacked-sequence {
                      seq-local: [w843 _ _ _ _] -> [_ w862 _ _ _]
                      tunnel: w837 -> [w852 _ _ _ _]
                      tunnel: w836 -> [w850 _ _ _ _]
                      tunnel: w835 -> [w849 _ _ _ _]
                      tunnel: w834 -> [w840 _ _ _ _]
                      frame #0 {
                        n492 = local read "LAB04-2 (SET)"() -> (w842:T5)
                        n493 = case shown="\"TEST SET UP\", Default" w849 {
                          tunnel: ["TEST SET UP-" "CYCLE TEST-" "T-RISE TEST-"] -> w845
                          frame "TEST SET UP", Default {
                          }
                          frame "CYCLE TEST" {
                          }
                          frame "T-RISE TEST" {
                          }
                        }
                        n494 = Unbundle(w842) -> ("DESCRIPTION"=w841:string)  [unwired: 4 out]
                        n495 = Concatenate Strings(w852, "LAB04-2\\", w850, "\\") -> (w846:string)
                        n496 = String To Path(string=w846) -> (path=w848:path)
                        n497 = Concatenate Strings(w846, w845, w841, "-", w840, ".tdms") -> (w843:string)
                        n498 = Create Folder(path (use dialog)=w848) -> (error out=w847:errorcluster)  [unwired: 2 in, 2 out]
                        n499 = call <vilib>:"Clear Errors.vi"("error in (no error)"=w847) -> ()  [unwired: 6 in, 1 out]
                      }
                      frame #1 {
                        n500 = String To Path(string=w862) -> (path=w856:path)
                        n501 = TDMS Open(5:FALSE, 6:FALSE, 10:T13."create or replace" ("operation (0:open)"), 11:w856) -> (0:w858:errorcluster, 3:→"LAB04-2 (TDMS)":refnum<k34>)  [unwired: 3 in]
                        n502 = local write "data file error"(w858) -> ()
                      }
                      frame #2 {
                        n503 = local read "LAB04-2 (SET)"() -> (w868:T5)
                        n504 = local read "LAB04-2 (TDMS)"() -> (w879:refnum<k34>)
                        n505 = Build Array("Testers Name", "Description", "Set Test Cycles", "T-Rise minutes", "T-Rise Deg C") -> (w869:string[])
                        n506 = Unbundle(w868) -> ("NAME"=w867:string, "DESCRIPTION"=w866:string, "CYCLES"=w865:dbl, "T-RISE mins"=w864:dbl, "T-RISE deg C"=w863:dbl)
                        n507 = Number To Decimal String(number=w865) -> (decimal integer string=w878:string)  [unwired: 1 in]
                        n508 = Number To Decimal String(number=w864) -> (decimal integer string=w877:string)  [unwired: 1 in]
                        n509 = Number To Decimal String(number=w863) -> (decimal integer string=w876:string)  [unwired: 1 in]
                        n510 = Build Array(w867, w866, w878, w877, w876) -> (w875:string[])
                        n511 = TDMS Set Properties(5:w875, 7:w869, 11:w879) -> ()  [unwired: 3 in, 4 out]
                      }
                      frame #3 {
                        w881 = 0.0
                        n512 = local read "LAB04-2 (DISP)"() -> (w883:T4)
                        n513 = Bundle(cluster=w883, "CYCLE"=w881, "MINS"=w881, "STATUS"="RUN") -> (w882:T4)
                        n514 = local write "LAB04-2 (DISP)"(w882) -> ()
                      }
                      frame #4 {
                        n515 = local read "LAB04-2 (SIG)"() -> (w886:T2)
                        n516 = local read "LAB04-2 (TEMP START)"() -> (w888:cluster{"TL":dbl, "TN":dbl})
                        n517 = Unbundle(w886) -> ("Tmp Live"=w885:dbl, "Tmp Neut"=w884:dbl)  [unwired: 3 out]
                        n518 = Bundle(cluster=w888, "TL"=w885, "TN"=w884) -> (w887:cluster{"TL":dbl, "TN":dbl})
                        n519 = local write "LAB04-2 (TEMP START)"(w887) -> ()
                      }
                    }
                  }
                }
              }
              event "LAB05-1 RUN": Value Change {
                n520 = event-data() -> ()  [unwired: 1 in, 6 out]
                n521 = case shown="True" w890 {
                  tunnel: w893 -> [_ w915]
                  tunnel: w892 -> [_ w914]
                  tunnel: w889 -> [w894 w913]
                  tunnel: w891 -> [_ w912]
                  frame False {
                    # "stop test"
                    n522 = stacked-sequence {
                      tunnel: w894 -> [w900 _]
                      frame #0 {
                        n523 = local read "LAB05-1 (DISP)"() -> (w899:T4)
                        n524 = Unbundle(w899) -> ("CYCLE"=w897:dbl, "MINS"=w898:dbl)  [unwired: 1 out]
                        n525 = case shown="\"CYCLE TEST\"" w900 {
                          tunnel: w898 -> [_ _ w907]
                          tunnel: w897 -> [w905 w906 _]
                          tunnel: [w905 w906 w907] -> w896
                          frame "TEST SET UP", Default {
                          }
                          frame "CYCLE TEST" {
                          }
                          frame "T-RISE TEST" {
                          }
                        }
                        n526 = local read "LAB05-1 (TDMS)"() -> (w904:refnum<k34>)
                        n527 = Build Array("STOPPED") -> (w901:string[])
                        n528 = Build Array(w896) -> (w895:dbl[])
                        n529 = TDMS Write(0:w904, 5:"TEST RESULT", 7:w901, 9:w895) -> ()  [unwired: 2 in, 4 out]
                      }
                      frame #1 {
                        n530 = local read "LAB05-1 (DISP)"() -> (w911:T4)
                        n531 = Bundle(cluster=w911, "STATUS"="STOP") -> (w909:T4)  [unwired: 2 in]
                        n532 = local write "LAB05-1 (RESULT)"(FALSE) -> ()
                        n533 = local write "LAB05-1 (DISP)"(w909) -> ()
                      }
                    }
                  }
                  frame True {
                    # "start new test and create test file"
                    n534 = stacked-sequence {
                      seq-local: [w921 _ _ _ _] -> [_ w940 _ _ _]
                      tunnel: w915 -> [w930 _ _ _ _]
                      tunnel: w914 -> [w928 _ _ _ _]
                      tunnel: w913 -> [w927 _ _ _ _]
                      tunnel: w912 -> [w918 _ _ _ _]
                      frame #0 {
                        n535 = local read "LAB05-1 (SET)"() -> (w920:T5)
                        n536 = case shown="\"TEST SET UP\", Default" w927 {
                          tunnel: ["TEST SET UP-" "CYCLE TEST-" "T-RISE TEST-"] -> w923
                          frame "TEST SET UP", Default {
                          }
                          frame "CYCLE TEST" {
                          }
                          frame "T-RISE TEST" {
                          }
                        }
                        n537 = Unbundle(w920) -> ("DESCRIPTION"=w919:string)  [unwired: 4 out]
                        n538 = Concatenate Strings(w930, "LAB05-1\\", w928, "\\") -> (w924:string)
                        n539 = String To Path(string=w924) -> (path=w926:path)
                        n540 = Concatenate Strings(w924, w923, w919, "-", w918, ".tdms") -> (w921:string)
                        n541 = Create Folder(path (use dialog)=w926) -> (error out=w925:errorcluster)  [unwired: 2 in, 2 out]
                        n542 = call <vilib>:"Clear Errors.vi"("error in (no error)"=w925) -> ()  [unwired: 6 in, 1 out]
                      }
                      frame #1 {
                        n543 = String To Path(string=w940) -> (path=w934:path)
                        n544 = TDMS Open(5:FALSE, 6:FALSE, 10:T13."create or replace" ("operation (0:open)"), 11:w934) -> (0:w936:errorcluster, 3:→"LAB05-1 (TDMS)":refnum<k34>)  [unwired: 3 in]
                        n545 = local write "data file error"(w936) -> ()
                      }
                      frame #2 {
                        n546 = local read "LAB05-1 (SET)"() -> (w946:T5)
                        n547 = local read "LAB05-1 (TDMS)"() -> (w957:refnum<k34>)
                        n548 = Build Array("Testers Name", "Description", "Set Test Cycles", "T-Rise minutes", "T-Rise Deg C") -> (w947:string[])
                        n549 = Unbundle(w946) -> ("NAME"=w945:string, "DESCRIPTION"=w944:string, "CYCLES"=w943:dbl, "T-RISE mins"=w942:dbl, "T-RISE deg C"=w941:dbl)
                        n550 = Number To Decimal String(number=w943) -> (decimal integer string=w956:string)  [unwired: 1 in]
                        n551 = Number To Decimal String(number=w942) -> (decimal integer string=w955:string)  [unwired: 1 in]
                        n552 = Number To Decimal String(number=w941) -> (decimal integer string=w954:string)  [unwired: 1 in]
                        n553 = Build Array(w945, w944, w956, w955, w954) -> (w953:string[])
                        n554 = TDMS Set Properties(5:w953, 7:w947, 11:w957) -> ()  [unwired: 3 in, 4 out]
                      }
                      frame #3 {
                        w959 = 0.0
                        n555 = local read "LAB05-1 (DISP)"() -> (w961:T4)
                        n556 = Bundle(cluster=w961, "CYCLE"=w959, "MINS"=w959, "STATUS"="RUN") -> (w960:T4)
                        n557 = local write "LAB05-1 (DISP)"(w960) -> ()
                      }
                      frame #4 {
                        n558 = local read "LAB05-1 (SIG)"() -> (w964:T2)
                        n559 = local read "LAB05-1 (TEMP START)"() -> (w966:cluster{"TL":dbl, "TN":dbl})
                        n560 = Unbundle(w964) -> ("Tmp Live"=w963:dbl, "Tmp Neut"=w962:dbl)  [unwired: 3 out]
                        n561 = Bundle(cluster=w966, "TL"=w963, "TN"=w962) -> (w965:cluster{"TL":dbl, "TN":dbl})
                        n562 = local write "LAB05-1 (TEMP START)"(w965) -> ()
                      }
                    }
                  }
                }
              }
              event "LAB05-2 RUN": Value Change {
                n563 = event-data() -> ()  [unwired: 1 in, 6 out]
                n564 = case shown="True" w968 {
                  tunnel: w971 -> [_ w993]
                  tunnel: w970 -> [_ w992]
                  tunnel: w967 -> [w972 w991]
                  tunnel: w969 -> [_ w990]
                  frame False {
                    # "stop test"
                    n565 = stacked-sequence {
                      tunnel: w972 -> [w978 _]
                      frame #0 {
                        n566 = local read "LAB05-2 (DISP)"() -> (w977:T4)
                        n567 = Unbundle(w977) -> ("CYCLE"=w975:dbl, "MINS"=w976:dbl)  [unwired: 1 out]
                        n568 = case shown="\"CYCLE TEST\"" w978 {
                          tunnel: w976 -> [_ _ w985]
                          tunnel: w975 -> [w983 w984 _]
                          tunnel: [w983 w984 w985] -> w974
                          frame "TEST SET UP", Default {
                          }
                          frame "CYCLE TEST" {
                          }
                          frame "T-RISE TEST" {
                          }
                        }
                        n569 = local read "LAB05-2 (TDMS)"() -> (w982:refnum<k34>)
                        n570 = Build Array("STOPPED") -> (w979:string[])
                        n571 = Build Array(w974) -> (w973:dbl[])
                        n572 = TDMS Write(0:w982, 5:"TEST RESULT", 7:w979, 9:w973) -> ()  [unwired: 2 in, 4 out]
                      }
                      frame #1 {
                        n573 = local read "LAB05-2 (DISP)"() -> (w989:T4)
                        n574 = Bundle(cluster=w989, "STATUS"="STOP") -> (w987:T4)  [unwired: 2 in]
                        n575 = local write "LAB05-2 (RESULT)"(FALSE) -> ()
                        n576 = local write "LAB05-2 (DISP)"(w987) -> ()
                      }
                    }
                  }
                  frame True {
                    # "start new test and create test file"
                    n577 = stacked-sequence {
                      seq-local: [w999 _ _ _ _] -> [_ w1018 _ _ _]
                      tunnel: w993 -> [w1008 _ _ _ _]
                      tunnel: w992 -> [w1006 _ _ _ _]
                      tunnel: w991 -> [w1005 _ _ _ _]
                      tunnel: w990 -> [w996 _ _ _ _]
                      frame #0 {
                        n578 = local read "LAB05-2 (SET)"() -> (w998:T5)
                        n579 = case shown="\"TEST SET UP\", Default" w1005 {
                          tunnel: ["TEST SET UP-" "CYCLE TEST-" "T-RISE TEST-"] -> w1001
                          frame "TEST SET UP", Default {
                          }
                          frame "CYCLE TEST" {
                          }
                          frame "T-RISE TEST" {
                          }
                        }
                        n580 = Unbundle(w998) -> ("DESCRIPTION"=w997:string)  [unwired: 4 out]
                        n581 = Concatenate Strings(w1008, "LAB05-2\\", w1006, "\\") -> (w1002:string)
                        n582 = String To Path(string=w1002) -> (path=w1004:path)
                        n583 = Concatenate Strings(w1002, w1001, w997, "-", w996, ".tdms") -> (w999:string)
                        n584 = Create Folder(path (use dialog)=w1004) -> (error out=w1003:errorcluster)  [unwired: 2 in, 2 out]
                        n585 = call <vilib>:"Clear Errors.vi"("error in (no error)"=w1003) -> ()  [unwired: 6 in, 1 out]
                      }
                      frame #1 {
                        n586 = String To Path(string=w1018) -> (path=w1012:path)
                        n587 = TDMS Open(5:FALSE, 6:FALSE, 10:T13."create or replace" ("operation (0:open)"), 11:w1012) -> (0:w1014:errorcluster, 3:→"LAB05-2 (TDMS)":refnum<k34>)  [unwired: 3 in]
                        n588 = local write "data file error"(w1014) -> ()
                      }
                      frame #2 {
                        n589 = local read "LAB05-2 (SET)"() -> (w1024:T5)
                        n590 = local read "LAB05-2 (TDMS)"() -> (w1035:refnum<k34>)
                        n591 = Build Array("Testers Name", "Description", "Set Test Cycles", "T-Rise minutes", "T-Rise Deg C") -> (w1025:string[])
                        n592 = Unbundle(w1024) -> ("NAME"=w1023:string, "DESCRIPTION"=w1022:string, "CYCLES"=w1021:dbl, "T-RISE mins"=w1020:dbl, "T-RISE deg C"=w1019:dbl)
                        n593 = Number To Decimal String(number=w1021) -> (decimal integer string=w1034:string)  [unwired: 1 in]
                        n594 = Number To Decimal String(number=w1020) -> (decimal integer string=w1033:string)  [unwired: 1 in]
                        n595 = Number To Decimal String(number=w1019) -> (decimal integer string=w1032:string)  [unwired: 1 in]
                        n596 = Build Array(w1023, w1022, w1034, w1033, w1032) -> (w1031:string[])
                        n597 = TDMS Set Properties(5:w1031, 7:w1025, 11:w1035) -> ()  [unwired: 3 in, 4 out]
                      }
                      frame #3 {
                        w1037 = 0.0
                        n598 = local read "LAB05-2 (DISP)"() -> (w1039:T4)
                        n599 = Bundle(cluster=w1039, "CYCLE"=w1037, "MINS"=w1037, "STATUS"="RUN") -> (w1038:T4)
                        n600 = local write "LAB05-2 (DISP)"(w1038) -> ()
                      }
                      frame #4 {
                        n601 = local read "LAB05-2 (SIG)"() -> (w1042:T2)
                        n602 = local read "LAB05-2 (TEMP START)"() -> (w1044:cluster{"TL":dbl, "TN":dbl})
                        n603 = Unbundle(w1042) -> ("Tmp Live"=w1041:dbl, "Tmp Neut"=w1040:dbl)  [unwired: 3 out]
                        n604 = Bundle(cluster=w1044, "TL"=w1041, "TN"=w1040) -> (w1043:cluster{"TL":dbl, "TN":dbl})
                        n605 = local write "LAB05-2 (TEMP START)"(w1043) -> ()
                      }
                    }
                  }
                }
              }
            }
          }
          frame #4 {
            # "check if test cycles reached for cycle tests, if so then test pass"
            n606 = stacked-sequence {
              tunnel: w1064 -> [_ _ _ _ _ _ _ _ _ _]
              tunnel: w1063 -> [_ _ _ _ _ _ _ _ _ _]
              tunnel: w1062 -> [_ _ _ _ _ _ _ _ _ _]
              tunnel: w1061 -> [_ _ _ _ _ _ _ _ _ _]
              tunnel: w1060 -> [_ _ _ _ _ _ _ _ _ _]
              tunnel: w1059 -> [_ _ _ _ _ _ _ _ _ _]
              tunnel: w1058 -> [_ _ _ _ _ _ _ _ _ _]
              tunnel: w1057 -> [_ _ _ _ _ _ _ _ _ _]
              tunnel: w1056 -> [_ _ _ _ _ _ _ _ _ _]
              tunnel: w1055 -> [_ _ _ _ _ _ _ _ _ _]
              tunnel: w1054 -> [w1069 _ _ _ _ _ _ _ _ _]
              tunnel: w1053 -> [_ w1104 _ _ _ _ _ _ _ _]
              tunnel: w1052 -> [_ _ w1143 _ _ _ _ _ _ _]
              tunnel: w1051 -> [_ _ _ w1182 _ _ _ _ _ _]
              tunnel: w1050 -> [_ _ _ _ w1221 _ _ _ _ _]
              tunnel: w1049 -> [_ _ _ _ _ w1260 _ _ _ _]
              tunnel: w1048 -> [_ _ _ _ _ _ w1299 _ _ _]
              tunnel: w1047 -> [_ _ _ _ _ _ _ w1338 _ _]
              tunnel: w1046 -> [_ _ _ _ _ _ _ _ w1377 _]
              tunnel: w1045 -> [_ _ _ _ _ _ _ _ _ w1416]
              frame #0 {
                # "LAB01-1"
                n607 = Less?(x=w1069, y=2) -> (x < y?=w1067:bool)
                n608 = local read "LAB01-1 (DISP)"() -> (w1070:T4)
                n609 = Unbundle(w1070) -> ("STATUS"=w1071:string)  [unwired: 2 out]
                n610 = Equal?(x=w1071, y="RUN") -> (x = y?=w1066:bool)
                n611 = And(x=w1066, y=w1067) -> (x .and. y?=w1065:bool)
                n612 = case shown="True" w1065 {
                  tunnel: w1070 -> [_ w1074]
                  tunnel: w1069 -> [_ w1079]
                  frame False {
                  }
                  frame True {
                    n613 = local read "LAB01-1 (SET)"() -> (w1081:T5)
                    n614 = local read "LAB01-1 (TDMS)"() -> (w1073:refnum<k34>)
                    n615 = Unbundle(w1074) -> ("CYCLE"=w1080:dbl)  [unwired: 2 out]
                    n616 = Unbundle(w1081) -> ("CYCLES"=w1076:dbl, "T-RISE mins"=w1078:dbl)  [unwired: 3 out]
                    n617 = case shown="\"TEST SET UP\", Default" w1079 {
                      tunnel: w1078 -> [_ _ w1088]
                      tunnel: [w1083 w1085 w1088] -> w1077
                      tunnel: w1076 -> [w1083 w1085 _]
                      tunnel: ["TEST SET UP CYCLES" "CYCLES" "T-RISE TEST"] -> w1075
                      frame "TEST SET UP", Default {
                      }
                      frame "CYCLE TEST" {
                      }
                      frame "T-RISE TEST" {
                      }
                    }
                    n618 = Greater Or Equal?(x=w1080, y=w1076) -> (x >= y?=w1082:bool)
                    n619 = case shown="True" w1082 {
                      tunnel: w1077 -> [w1092 _]
                      tunnel: w1075 -> [w1091 _]
                      tunnel: w1074 -> [w1090 _]
                      tunnel: w1073 -> [w1089 _]
                      frame True {
                        n620 = stacked-sequence {
                          tunnel: w1092 -> [w1096 _]
                          tunnel: w1091 -> [w1094 _]
                          tunnel: w1090 -> [_ w1102]
                          tunnel: w1089 -> [w1093 _]
                          frame #0 {
                            n621 = Build Array(w1094) -> (w1097:string[])
                            n622 = Build Array(w1096) -> (w1095:dbl[])
                            n623 = TDMS Write(0:w1093, 5:"TEST PASS", 7:w1097, 9:w1095) -> (15:w1099:errorcluster)  [unwired: 2 in, 3 out]
                            n624 = local write "data file error"(w1099) -> ()
                          }
                          frame #1 {
                            n625 = Bundle(cluster=w1102, "STATUS"="CYCLE PASS") -> (w1100:T4)  [unwired: 2 in]
                            n626 = local write "LAB01-1 (RESULT)"(TRUE) -> ()
                            n627 = local write "LAB01-1 (DISP)"(w1100) -> ()
                          }
                        }
                      }
                      frame False {
                      }
                    }
                  }
                }
              }
              frame #1 {
                # "LAB01-2"
                n628 = Less?(x=w1104, y=2) -> (x < y?=w1107:bool)
                n629 = local read "LAB01-2 (DISP)"() -> (w1109:T4)
                n630 = Unbundle(w1109) -> ("STATUS"=w1110:string)  [unwired: 2 out]
                n631 = Equal?(x=w1110, y="RUN") -> (x = y?=w1106:bool)
                n632 = And(x=w1106, y=w1107) -> (x .and. y?=w1105:bool)
                n633 = case shown="True" w1105 {
                  tunnel: w1109 -> [_ w1113]
                  tunnel: w1104 -> [_ w1118]
                  frame False {
                  }
                  frame True {
                    n634 = local read "LAB01-2 (TDMS)"() -> (w1112:refnum<k34>)
                    n635 = local read "LAB01-2(SET)"() -> (w1120:T5)
                    n636 = Unbundle(w1113) -> ("CYCLE"=w1119:dbl)  [unwired: 2 out]
                    n637 = Unbundle(w1120) -> ("CYCLES"=w1115:dbl, "T-RISE mins"=w1117:dbl)  [unwired: 3 out]
                    n638 = case shown="\"TEST SET UP\", Default" w1118 {
                      tunnel: w1117 -> [_ _ w1127]
                      tunnel: [w1122 w1124 w1127] -> w1116
                      tunnel: w1115 -> [w1122 w1124 _]
                      tunnel: ["TEST SET UP CYCLES" "CYCLES" "T-RISE TEST"] -> w1114
                      frame "TEST SET UP", Default {
                      }
                      frame "CYCLE TEST" {
                      }
                      frame "T-RISE TEST" {
                      }
                    }
                    n639 = Greater Or Equal?(x=w1119, y=w1115) -> (x >= y?=w1121:bool)
                    n640 = case shown="True" w1121 {
                      tunnel: w1116 -> [w1131 _]
                      tunnel: w1114 -> [w1130 _]
                      tunnel: w1113 -> [w1129 _]
                      tunnel: w1112 -> [w1128 _]
                      frame True {
                        n641 = stacked-sequence {
                          tunnel: w1131 -> [w1135 _]
                          tunnel: w1130 -> [w1133 _]
                          tunnel: w1129 -> [_ w1141]
                          tunnel: w1128 -> [w1132 _]
                          frame #0 {
                            n642 = Build Array(w1133) -> (w1136:string[])
                            n643 = Build Array(w1135) -> (w1134:dbl[])
                            n644 = TDMS Write(0:w1132, 5:"TEST PASS", 7:w1136, 9:w1134) -> (15:w1138:errorcluster)  [unwired: 2 in, 3 out]
                            n645 = local write "data file error"(w1138) -> ()
                          }
                          frame #1 {
                            n646 = Bundle(cluster=w1141, "STATUS"="STOP") -> (w1139:T4)  [unwired: 2 in]
                            n647 = local write "LAB01-2 (RESULT)"(TRUE) -> ()
                            n648 = local write "LAB01-2 (DISP)"(w1139) -> ()
                          }
                        }
                      }
                      frame False {
                      }
                    }
                  }
                }
              }
              frame #2 {
                # "LAB02-1"
                n649 = Less?(x=w1143, y=2) -> (x < y?=w1146:bool)
                n650 = local read "LAB02-1 (DISP)"() -> (w1148:T4)
                n651 = Unbundle(w1148) -> ("STATUS"=w1149:string)  [unwired: 2 out]
                n652 = Equal?(x=w1149, y="RUN") -> (x = y?=w1145:bool)
                n653 = And(x=w1145, y=w1146) -> (x .and. y?=w1144:bool)
                n654 = case shown="True" w1144 {
                  tunnel: w1148 -> [_ w1152]
                  tunnel: w1143 -> [_ w1157]
                  frame False {
                  }
                  frame True {
                    n655 = local read "LAB02-1 (SET)"() -> (w1159:T5)
                    n656 = local read "LAB02-1 (TDMS)"() -> (w1151:refnum<k34>)
                    n657 = Unbundle(w1152) -> ("CYCLE"=w1158:dbl)  [unwired: 2 out]
                    n658 = Unbundle(w1159) -> ("CYCLES"=w1154:dbl, "T-RISE mins"=w1156:dbl)  [unwired: 3 out]
                    n659 = case shown="\"TEST SET UP\", Default" w1157 {
                      tunnel: w1156 -> [_ _ w1166]
                      tunnel: [w1161 w1163 w1166] -> w1155
                      tunnel: w1154 -> [w1161 w1163 _]
                      tunnel: ["TEST SET UP CYCLES" "CYCLES" "T-RISE TEST"] -> w1153
                      frame "TEST SET UP", Default {
                      }
                      frame "CYCLE TEST" {
                      }
                      frame "T-RISE TEST" {
                      }
                    }
                    n660 = Greater Or Equal?(x=w1158, y=w1154) -> (x >= y?=w1160:bool)
                    n661 = case shown="True" w1160 {
                      tunnel: w1155 -> [w1170 _]
                      tunnel: w1153 -> [w1169 _]
                      tunnel: w1152 -> [w1168 _]
                      tunnel: w1151 -> [w1167 _]
                      frame True {
                        n662 = stacked-sequence {
                          tunnel: w1170 -> [w1174 _]
                          tunnel: w1169 -> [w1172 _]
                          tunnel: w1168 -> [_ w1180]
                          tunnel: w1167 -> [w1171 _]
                          frame #0 {
                            n663 = Build Array(w1172) -> (w1175:string[])
                            n664 = Build Array(w1174) -> (w1173:dbl[])
                            n665 = TDMS Write(0:w1171, 5:"TEST PASS", 7:w1175, 9:w1173) -> (15:w1177:errorcluster)  [unwired: 2 in, 3 out]
                            n666 = local write "data file error"(w1177) -> ()
                          }
                          frame #1 {
                            n667 = Bundle(cluster=w1180, "STATUS"="STOP") -> (w1178:T4)  [unwired: 2 in]
                            n668 = local write "LAB02-1 (RESULT)"(TRUE) -> ()
                            n669 = local write "LAB02-1 (DISP)"(w1178) -> ()
                          }
                        }
                      }
                      frame False {
                      }
                    }
                  }
                }
              }
              frame #3 {
                # "LAB02-2"
                n670 = Less?(x=w1182, y=2) -> (x < y?=w1185:bool)
                n671 = local read "LAB02-2 (DISP)"() -> (w1187:T4)
                n672 = Unbundle(w1187) -> ("STATUS"=w1188:string)  [unwired: 2 out]
                n673 = Equal?(x=w1188, y="RUN") -> (x = y?=w1184:bool)
                n674 = And(x=w1184, y=w1185) -> (x .and. y?=w1183:bool)
                n675 = case shown="True" w1183 {
                  tunnel: w1187 -> [_ w1191]
                  tunnel: w1182 -> [_ w1196]
                  frame False {
                  }
                  frame True {
                    n676 = local read "LAB02-2 (SET)"() -> (w1198:T5)
                    n677 = local read "LAB02-2 (TDMS)"() -> (w1190:refnum<k34>)
                    n678 = Unbundle(w1191) -> ("CYCLE"=w1197:dbl)  [unwired: 2 out]
                    n679 = Unbundle(w1198) -> ("CYCLES"=w1193:dbl, "T-RISE mins"=w1195:dbl)  [unwired: 3 out]
                    n680 = case shown="\"TEST SET UP\", Default" w1196 {
                      tunnel: w1195 -> [_ _ w1205]
                      tunnel: [w1200 w1202 w1205] -> w1194
                      tunnel: w1193 -> [w1200 w1202 _]
                      tunnel: ["TEST SET UP CYCLES" "CYCLES" "T-RISE TEST"] -> w1192
                      frame "TEST SET UP", Default {
                      }
                      frame "CYCLE TEST" {
                      }
                      frame "T-RISE TEST" {
                      }
                    }
                    n681 = Greater Or Equal?(x=w1197, y=w1193) -> (x >= y?=w1199:bool)
                    n682 = case shown="True" w1199 {
                      tunnel: w1194 -> [w1209 _]
                      tunnel: w1192 -> [w1208 _]
                      tunnel: w1191 -> [w1207 _]
                      tunnel: w1190 -> [w1206 _]
                      frame True {
                        n683 = stacked-sequence {
                          tunnel: w1209 -> [w1213 _]
                          tunnel: w1208 -> [w1211 _]
                          tunnel: w1207 -> [_ w1219]
                          tunnel: w1206 -> [w1210 _]
                          frame #0 {
                            n684 = Build Array(w1211) -> (w1214:string[])
                            n685 = Build Array(w1213) -> (w1212:dbl[])
                            n686 = TDMS Write(0:w1210, 5:"TEST PASS", 7:w1214, 9:w1212) -> (15:w1216:errorcluster)  [unwired: 2 in, 3 out]
                            n687 = local write "data file error"(w1216) -> ()
                          }
                          frame #1 {
                            n688 = Bundle(cluster=w1219, "STATUS"="STOP") -> (w1217:T4)  [unwired: 2 in]
                            n689 = local write "LAB02-2 (RESULT)"(TRUE) -> ()
                            n690 = local write "LAB02-2 (DISP)"(w1217) -> ()
                          }
                        }
                      }
                      frame False {
                      }
                    }
                  }
                }
              }
              frame #4 {
                # "LAB03-1"
                n691 = Less?(x=w1221, y=2) -> (x < y?=w1224:bool)
                n692 = local read "LAB03-1 (DISP)"() -> (w1226:T4)
                n693 = Unbundle(w1226) -> ("STATUS"=w1227:string)  [unwired: 2 out]
                n694 = Equal?(x=w1227, y="RUN") -> (x = y?=w1223:bool)
                n695 = And(x=w1223, y=w1224) -> (x .and. y?=w1222:bool)
                n696 = case shown="True" w1222 {
                  tunnel: w1226 -> [_ w1230]
                  tunnel: w1221 -> [_ w1235]
                  frame False {
                  }
                  frame True {
                    n697 = local read "LAB03-1 (SET)"() -> (w1237:T5)
                    n698 = local read "LAB03-1 (TDMS)"() -> (w1229:refnum<k34>)
                    n699 = Unbundle(w1230) -> ("CYCLE"=w1236:dbl)  [unwired: 2 out]
                    n700 = Unbundle(w1237) -> ("CYCLES"=w1232:dbl, "T-RISE mins"=w1234:dbl)  [unwired: 3 out]
                    n701 = case shown="\"TEST SET UP\", Default" w1235 {
                      tunnel: w1234 -> [_ _ w1244]
                      tunnel: [w1239 w1241 w1244] -> w1233
                      tunnel: w1232 -> [w1239 w1241 _]
                      tunnel: ["TEST SET UP CYCLES" "CYCLES" "T-RISE TEST"] -> w1231
                      frame "TEST SET UP", Default {
                      }
                      frame "CYCLE TEST" {
                      }
                      frame "T-RISE TEST" {
                      }
                    }
                    n702 = Greater Or Equal?(x=w1236, y=w1232) -> (x >= y?=w1238:bool)
                    n703 = case shown="True" w1238 {
                      tunnel: w1233 -> [w1248 _]
                      tunnel: w1231 -> [w1247 _]
                      tunnel: w1230 -> [w1246 _]
                      tunnel: w1229 -> [w1245 _]
                      frame True {
                        n704 = stacked-sequence {
                          tunnel: w1248 -> [w1252 _]
                          tunnel: w1247 -> [w1250 _]
                          tunnel: w1246 -> [_ w1258]
                          tunnel: w1245 -> [w1249 _]
                          frame #0 {
                            n705 = Build Array(w1250) -> (w1253:string[])
                            n706 = Build Array(w1252) -> (w1251:dbl[])
                            n707 = TDMS Write(0:w1249, 5:"TEST PASS", 7:w1253, 9:w1251) -> (15:w1255:errorcluster)  [unwired: 2 in, 3 out]
                            n708 = local write "data file error"(w1255) -> ()
                          }
                          frame #1 {
                            n709 = Bundle(cluster=w1258, "STATUS"="STOP") -> (w1256:T4)  [unwired: 2 in]
                            n710 = local write "LAB03-1 (RESULT)"(TRUE) -> ()
                            n711 = local write "LAB03-1 (DISP)"(w1256) -> ()
                          }
                        }
                      }
                      frame False {
                      }
                    }
                  }
                }
              }
              frame #5 {
                # "LAB03-2"
                n712 = Less?(x=w1260, y=2) -> (x < y?=w1263:bool)
                n713 = local read "LAB03-2 (DISP)"() -> (w1265:T4)
                n714 = Unbundle(w1265) -> ("STATUS"=w1266:string)  [unwired: 2 out]
                n715 = Equal?(x=w1266, y="RUN") -> (x = y?=w1262:bool)
                n716 = And(x=w1262, y=w1263) -> (x .and. y?=w1261:bool)
                n717 = case shown="True" w1261 {
                  tunnel: w1265 -> [_ w1269]
                  tunnel: w1260 -> [_ w1274]
                  frame False {
                  }
                  frame True {
                    n718 = local read "LAB03-2 (SET)"() -> (w1276:T5)
                    n719 = local read "LAB03-2 (TDMS)"() -> (w1268:refnum<k34>)
                    n720 = Unbundle(w1269) -> ("CYCLE"=w1275:dbl)  [unwired: 2 out]
                    n721 = Unbundle(w1276) -> ("CYCLES"=w1271:dbl, "T-RISE mins"=w1273:dbl)  [unwired: 3 out]
                    n722 = case shown="\"TEST SET UP\", Default" w1274 {
                      tunnel: w1273 -> [_ _ w1283]
                      tunnel: [w1278 w1280 w1283] -> w1272
                      tunnel: w1271 -> [w1278 w1280 _]
                      tunnel: ["TEST SET UP CYCLES" "CYCLES" "T-RISE TEST"] -> w1270
                      frame "TEST SET UP", Default {
                      }
                      frame "CYCLE TEST" {
                      }
                      frame "T-RISE TEST" {
                      }
                    }
                    n723 = Greater Or Equal?(x=w1275, y=w1271) -> (x >= y?=w1277:bool)
                    n724 = case shown="True" w1277 {
                      tunnel: w1272 -> [w1287 _]
                      tunnel: w1270 -> [w1286 _]
                      tunnel: w1269 -> [w1285 _]
                      tunnel: w1268 -> [w1284 _]
                      frame True {
                        n725 = stacked-sequence {
                          tunnel: w1287 -> [w1291 _]
                          tunnel: w1286 -> [w1289 _]
                          tunnel: w1285 -> [_ w1297]
                          tunnel: w1284 -> [w1288 _]
                          frame #0 {
                            n726 = Build Array(w1289) -> (w1292:string[])
                            n727 = Build Array(w1291) -> (w1290:dbl[])
                            n728 = TDMS Write(0:w1288, 5:"TEST PASS", 7:w1292, 9:w1290) -> (15:w1294:errorcluster)  [unwired: 2 in, 3 out]
                            n729 = local write "data file error"(w1294) -> ()
                          }
                          frame #1 {
                            n730 = Bundle(cluster=w1297, "STATUS"="STOP") -> (w1295:T4)  [unwired: 2 in]
                            n731 = local write "LAB03-2 (RESULT)"(TRUE) -> ()
                            n732 = local write "LAB03-2 (DISP)"(w1295) -> ()
                          }
                        }
                      }
                      frame False {
                      }
                    }
                  }
                }
              }
              frame #6 {
                # "LAB04-1"
                n733 = Less?(x=w1299, y=2) -> (x < y?=w1302:bool)
                n734 = local read "LAB04-1 (DISP)"() -> (w1304:T4)
                n735 = Unbundle(w1304) -> ("STATUS"=w1305:string)  [unwired: 2 out]
                n736 = Equal?(x=w1305, y="RUN") -> (x = y?=w1301:bool)
                n737 = And(x=w1301, y=w1302) -> (x .and. y?=w1300:bool)
                n738 = case shown="True" w1300 {
                  tunnel: w1304 -> [_ w1308]
                  tunnel: w1299 -> [_ w1313]
                  frame False {
                  }
                  frame True {
                    n739 = local read "LAB04-1 (SET)"() -> (w1315:T5)
                    n740 = local read "LAB04-1 (TDMS)"() -> (w1307:refnum<k34>)
                    n741 = Unbundle(w1308) -> ("CYCLE"=w1314:dbl)  [unwired: 2 out]
                    n742 = Unbundle(w1315) -> ("CYCLES"=w1310:dbl, "T-RISE mins"=w1312:dbl)  [unwired: 3 out]
                    n743 = case shown="\"TEST SET UP\", Default" w1313 {
                      tunnel: w1312 -> [_ _ w1322]
                      tunnel: [w1317 w1319 w1322] -> w1311
                      tunnel: w1310 -> [w1317 w1319 _]
                      tunnel: ["TEST SET UP CYCLES" "CYCLES" "T-RISE TEST"] -> w1309
                      frame "TEST SET UP", Default {
                      }
                      frame "CYCLE TEST" {
                      }
                      frame "T-RISE TEST" {
                      }
                    }
                    n744 = Greater Or Equal?(x=w1314, y=w1310) -> (x >= y?=w1316:bool)
                    n745 = case shown="True" w1316 {
                      tunnel: w1311 -> [w1326 _]
                      tunnel: w1309 -> [w1325 _]
                      tunnel: w1308 -> [w1324 _]
                      tunnel: w1307 -> [w1323 _]
                      frame True {
                        n746 = stacked-sequence {
                          tunnel: w1326 -> [w1330 _]
                          tunnel: w1325 -> [w1328 _]
                          tunnel: w1324 -> [_ w1336]
                          tunnel: w1323 -> [w1327 _]
                          frame #0 {
                            n747 = Build Array(w1328) -> (w1331:string[])
                            n748 = Build Array(w1330) -> (w1329:dbl[])
                            n749 = TDMS Write(0:w1327, 5:"TEST PASS", 7:w1331, 9:w1329) -> (15:w1333:errorcluster)  [unwired: 2 in, 3 out]
                            n750 = local write "data file error"(w1333) -> ()
                          }
                          frame #1 {
                            n751 = Bundle(cluster=w1336, "STATUS"="STOP") -> (w1334:T4)  [unwired: 2 in]
                            n752 = local write "LAB04-1 (RESULT)"(TRUE) -> ()
                            n753 = local write "LAB04-1 (DISP)"(w1334) -> ()
                          }
                        }
                      }
                      frame False {
                      }
                    }
                  }
                }
              }
              frame #7 {
                # "LAB04-2"
                n754 = Less?(x=w1338, y=2) -> (x < y?=w1341:bool)
                n755 = local read "LAB04-2 (DISP)"() -> (w1343:T4)
                n756 = Unbundle(w1343) -> ("STATUS"=w1344:string)  [unwired: 2 out]
                n757 = Equal?(x=w1344, y="RUN") -> (x = y?=w1340:bool)
                n758 = And(x=w1340, y=w1341) -> (x .and. y?=w1339:bool)
                n759 = case shown="True" w1339 {
                  tunnel: w1343 -> [_ w1347]
                  tunnel: w1338 -> [_ w1352]
                  frame False {
                  }
                  frame True {
                    n760 = local read "LAB04-2 (SET)"() -> (w1354:T5)
                    n761 = local read "LAB04-2 (TDMS)"() -> (w1346:refnum<k34>)
                    n762 = Unbundle(w1347) -> ("CYCLE"=w1353:dbl)  [unwired: 2 out]
                    n763 = Unbundle(w1354) -> ("CYCLES"=w1349:dbl, "T-RISE mins"=w1351:dbl)  [unwired: 3 out]
                    n764 = case shown="\"TEST SET UP\", Default" w1352 {
                      tunnel: w1351 -> [_ _ w1361]
                      tunnel: [w1356 w1358 w1361] -> w1350
                      tunnel: w1349 -> [w1356 w1358 _]
                      tunnel: ["TEST SET UP CYCLES" "CYCLES" "T-RISE TEST"] -> w1348
                      frame "TEST SET UP", Default {
                      }
                      frame "CYCLE TEST" {
                      }
                      frame "T-RISE TEST" {
                      }
                    }
                    n765 = Greater Or Equal?(x=w1353, y=w1349) -> (x >= y?=w1355:bool)
                    n766 = case shown="True" w1355 {
                      tunnel: w1350 -> [w1365 _]
                      tunnel: w1348 -> [w1364 _]
                      tunnel: w1347 -> [w1363 _]
                      tunnel: w1346 -> [w1362 _]
                      frame True {
                        n767 = stacked-sequence {
                          tunnel: w1365 -> [w1369 _]
                          tunnel: w1364 -> [w1367 _]
                          tunnel: w1363 -> [_ w1375]
                          tunnel: w1362 -> [w1366 _]
                          frame #0 {
                            n768 = Build Array(w1367) -> (w1370:string[])
                            n769 = Build Array(w1369) -> (w1368:dbl[])
                            n770 = TDMS Write(0:w1366, 5:"TEST PASS", 7:w1370, 9:w1368) -> (15:w1372:errorcluster)  [unwired: 2 in, 3 out]
                            n771 = local write "data file error"(w1372) -> ()
                          }
                          frame #1 {
                            n772 = Bundle(cluster=w1375, "STATUS"="STOP") -> (w1373:T4)  [unwired: 2 in]
                            n773 = local write "LAB04-2 (RESULT)"(TRUE) -> ()
                            n774 = local write "LAB04-2 (DISP)"(w1373) -> ()
                          }
                        }
                      }
                      frame False {
                      }
                    }
                  }
                }
              }
              frame #8 {
                # "LAB05-1"
                n775 = Less?(x=w1377, y=2) -> (x < y?=w1380:bool)
                n776 = local read "LAB05-1 (DISP)"() -> (w1382:T4)
                n777 = Unbundle(w1382) -> ("STATUS"=w1383:string)  [unwired: 2 out]
                n778 = Equal?(x=w1383, y="RUN") -> (x = y?=w1379:bool)
                n779 = And(x=w1379, y=w1380) -> (x .and. y?=w1378:bool)
                n780 = case shown="True" w1378 {
                  tunnel: w1382 -> [_ w1386]
                  tunnel: w1377 -> [_ w1391]
                  frame False {
                  }
                  frame True {
                    n781 = local read "LAB05-1 (SET)"() -> (w1393:T5)
                    n782 = local read "LAB05-1 (TDMS)"() -> (w1385:refnum<k34>)
                    n783 = Unbundle(w1386) -> ("CYCLE"=w1392:dbl)  [unwired: 2 out]
                    n784 = Unbundle(w1393) -> ("CYCLES"=w1388:dbl, "T-RISE mins"=w1390:dbl)  [unwired: 3 out]
                    n785 = case shown="\"TEST SET UP\", Default" w1391 {
                      tunnel: w1390 -> [_ _ w1400]
                      tunnel: [w1395 w1397 w1400] -> w1389
                      tunnel: w1388 -> [w1395 w1397 _]
                      tunnel: ["TEST SET UP CYCLES" "CYCLES" "T-RISE TEST"] -> w1387
                      frame "TEST SET UP", Default {
                      }
                      frame "CYCLE TEST" {
                      }
                      frame "T-RISE TEST" {
                      }
                    }
                    n786 = Greater Or Equal?(x=w1392, y=w1388) -> (x >= y?=w1394:bool)
                    n787 = case shown="True" w1394 {
                      tunnel: w1389 -> [w1404 _]
                      tunnel: w1387 -> [w1403 _]
                      tunnel: w1386 -> [w1402 _]
                      tunnel: w1385 -> [w1401 _]
                      frame True {
                        n788 = stacked-sequence {
                          tunnel: w1404 -> [w1408 _]
                          tunnel: w1403 -> [w1406 _]
                          tunnel: w1402 -> [_ w1414]
                          tunnel: w1401 -> [w1405 _]
                          frame #0 {
                            n789 = Build Array(w1406) -> (w1409:string[])
                            n790 = Build Array(w1408) -> (w1407:dbl[])
                            n791 = TDMS Write(0:w1405, 5:"TEST PASS", 7:w1409, 9:w1407) -> (15:w1411:errorcluster)  [unwired: 2 in, 3 out]
                            n792 = local write "data file error"(w1411) -> ()
                          }
                          frame #1 {
                            n793 = Bundle(cluster=w1414, "STATUS"="STOP") -> (w1412:T4)  [unwired: 2 in]
                            n794 = local write "LAB05-1 (RESULT)"(TRUE) -> ()
                            n795 = local write "LAB05-1 (DISP)"(w1412) -> ()
                          }
                        }
                      }
                      frame False {
                      }
                    }
                  }
                }
              }
              frame #9 {
                # "LAB05-2"
                n796 = Less?(x=w1416, y=2) -> (x < y?=w1419:bool)
                n797 = local read "LAB05-2 (DISP)"() -> (w1421:T4)
                n798 = Unbundle(w1421) -> ("STATUS"=w1422:string)  [unwired: 2 out]
                n799 = Equal?(x=w1422, y="RUN") -> (x = y?=w1418:bool)
                n800 = And(x=w1418, y=w1419) -> (x .and. y?=w1417:bool)
                n801 = case shown="True" w1417 {
                  tunnel: w1421 -> [_ w1425]
                  tunnel: w1416 -> [_ w1430]
                  frame False {
                  }
                  frame True {
                    n802 = local read "LAB05-2 (SET)"() -> (w1432:T5)
                    n803 = local read "LAB05-1 (TDMS)"() -> (w1424:refnum<k34>)
                    n804 = Unbundle(w1425) -> ("CYCLE"=w1431:dbl)  [unwired: 2 out]
                    n805 = Unbundle(w1432) -> ("CYCLES"=w1427:dbl, "T-RISE mins"=w1429:dbl)  [unwired: 3 out]
                    n806 = case shown="\"TEST SET UP\", Default" w1430 {
                      tunnel: w1429 -> [_ _ w1439]
                      tunnel: [w1434 w1436 w1439] -> w1428
                      tunnel: w1427 -> [w1434 w1436 _]
                      tunnel: ["TEST SET UP CYCLES" "CYCLES" "T-RISE TEST"] -> w1426
                      frame "TEST SET UP", Default {
                      }
                      frame "CYCLE TEST" {
                      }
                      frame "T-RISE TEST" {
                      }
                    }
                    n807 = Greater Or Equal?(x=w1431, y=w1427) -> (x >= y?=w1433:bool)
                    n808 = case shown="True" w1433 {
                      tunnel: w1428 -> [w1443 _]
                      tunnel: w1426 -> [w1442 _]
                      tunnel: w1425 -> [w1441 _]
                      tunnel: w1424 -> [w1440 _]
                      frame True {
                        n809 = stacked-sequence {
                          tunnel: w1443 -> [w1447 _]
                          tunnel: w1442 -> [w1445 _]
                          tunnel: w1441 -> [_ w1453]
                          tunnel: w1440 -> [w1444 _]
                          frame #0 {
                            n810 = Build Array(w1445) -> (w1448:string[])
                            n811 = Build Array(w1447) -> (w1446:dbl[])
                            n812 = TDMS Write(0:w1444, 5:"TEST PASS", 7:w1448, 9:w1446) -> (15:w1450:errorcluster)  [unwired: 2 in, 3 out]
                            n813 = local write "data file error"(w1450) -> ()
                          }
                          frame #1 {
                            n814 = Bundle(cluster=w1453, "STATUS"="STOP") -> (w1451:T4)  [unwired: 2 in]
                            n815 = local write "LAB05-2 (RESULT)"(TRUE) -> ()
                            n816 = local write "LAB05-2 (DISP)"(w1451) -> ()
                          }
                        }
                      }
                      frame False {
                      }
                    }
                  }
                }
              }
            }
          }
          frame #5 {
            # "check if test cycles reached for temperature rise test"
            n817 = stacked-sequence {
              tunnel: w1475 -> [_ _ _ _ _ _ _ _ _ _]
              tunnel: w1474 -> [_ _ _ _ _ _ _ _ _ _]
              tunnel: w1473 -> [_ _ _ _ _ _ _ _ _ _]
              tunnel: w1472 -> [_ _ _ _ _ _ _ _ _ _]
              tunnel: w1471 -> [_ _ _ _ _ _ _ _ _ _]
              tunnel: w1470 -> [_ _ _ _ _ _ _ _ _ _]
              tunnel: w1469 -> [_ _ _ _ _ _ _ _ _ _]
              tunnel: w1468 -> [_ _ _ _ _ _ _ _ _ _]
              tunnel: w1467 -> [_ _ _ _ _ _ _ _ _ _]
              tunnel: w1466 -> [_ _ _ _ _ _ _ _ _ _]
              tunnel: w1465 -> [w1481 _ _ _ _ _ _ _ _ _]
              tunnel: w1464 -> [w1476 w1507 w1537 w1567 w1597 w1627 w1657 w1687 w1717 w1747]
              tunnel: w1463 -> [_ w1506 _ _ _ _ _ _ _ _]
              tunnel: w1462 -> [_ _ w1536 _ _ _ _ _ _ _]
              tunnel: w1461 -> [_ _ _ w1566 _ _ _ _ _ _]
              tunnel: w1460 -> [_ _ _ _ w1596 _ _ _ _ _]
              tunnel: w1459 -> [_ _ _ _ _ w1626 _ _ _ _]
              tunnel: w1458 -> [_ _ _ _ _ _ w1656 _ _ _]
              tunnel: w1457 -> [_ _ _ _ _ _ _ w1686 _ _]
              tunnel: w1456 -> [_ _ _ _ _ _ _ _ w1716 _]
              tunnel: w1455 -> [_ _ _ _ _ _ _ _ _ w1746]
              frame #0 {
                # "LAB01-1"
                n818 = Equal?(x=w1481, y=2) -> (x = y?=w1479:bool)
                n819 = local read "LAB01-1 (DISP)"() -> (w1482:T4)
                n820 = Unbundle(w1482) -> ("STATUS"=w1483:string)  [unwired: 2 out]
                n821 = Equal?(x=w1483, y="RUN") -> (x = y?=w1478:bool)
                n822 = And(x=w1478, y=w1479) -> (x .and. y?=w1477:bool)
                n823 = case shown="True" w1477 {
                  tunnel: w1482 -> [_ w1486]
                  tunnel: w1476 -> [_ w1489]
                  frame False {
                  }
                  frame True {
                    n824 = local read "LAB01-1 (SET)"() -> (w1488:T5)
                    n825 = local read "LAB01-1 (TDMS)"() -> (w1485:refnum<k34>)
                    n826 = Unbundle(w1486) -> ("CYCLE"=w1490:dbl)  [unwired: 2 out]
                    n827 = Unbundle(w1488) -> ("T-RISE mins"=w1487:dbl)  [unwired: 4 out]
                    n828 = Greater Or Equal?(x=w1490, y=w1489) -> (x >= y?=w1491:bool)
                    n829 = case shown="True" w1491 {
                      tunnel: w1487 -> [w1494 _]
                      tunnel: w1486 -> [w1493 _]
                      tunnel: w1485 -> [w1492 _]
                      frame True {
                        n830 = stacked-sequence {
                          tunnel: w1494 -> [w1497 _]
                          tunnel: w1493 -> [_ w1502]
                          tunnel: w1492 -> [w1495 _]
                          frame #0 {
                            n831 = Build Array("T-RISE") -> (w1499:string[])
                            n832 = Build Array(w1497) -> (w1498:dbl[])
                            n833 = TDMS Write(0:w1495, 5:"TEST PASS", 7:w1499, 9:w1498) -> (15:w1501:errorcluster)  [unwired: 2 in, 3 out]
                            n834 = local write "data file error"(w1501) -> ()
                          }
                          frame #1 {
                            n835 = Bundle(cluster=w1502, "STATUS"="T-RISE PASS") -> (w1504:T4)  [unwired: 2 in]
                            n836 = local write "LAB01-1 (RESULT)"(TRUE) -> ()
                            n837 = local write "LAB01-1 (DISP)"(w1504) -> ()
                          }
                        }
                      }
                      frame False {
                      }
                    }
                  }
                }
              }
              frame #1 {
                # "LAB01-2"
                n838 = Equal?(x=w1506, y=2) -> (x = y?=w1510:bool)
                n839 = local read "LAB01-2 (DISP)"() -> (w1512:T4)
                n840 = Unbundle(w1512) -> ("STATUS"=w1513:string)  [unwired: 2 out]
                n841 = Equal?(x=w1513, y="RUN") -> (x = y?=w1509:bool)
                n842 = And(x=w1509, y=w1510) -> (x .and. y?=w1508:bool)
                n843 = case shown="True" w1508 {
                  tunnel: w1512 -> [_ w1516]
                  tunnel: w1507 -> [_ w1519]
                  frame False {
                  }
                  frame True {
                    n844 = local read "LAB01-2(SET)"() -> (w1518:T5)
                    n845 = local read "LAB01-2 (TDMS)"() -> (w1515:refnum<k34>)
                    n846 = Unbundle(w1516) -> ("CYCLE"=w1520:dbl)  [unwired: 2 out]
                    n847 = Unbundle(w1518) -> ("T-RISE mins"=w1517:dbl)  [unwired: 4 out]
                    n848 = Greater Or Equal?(x=w1520, y=w1519) -> (x >= y?=w1521:bool)
                    n849 = case shown="True" w1521 {
                      tunnel: w1517 -> [w1524 _]
                      tunnel: w1516 -> [w1523 _]
                      tunnel: w1515 -> [w1522 _]
                      frame True {
                        n850 = stacked-sequence {
                          tunnel: w1524 -> [w1527 _]
                          tunnel: w1523 -> [_ w1532]
                          tunnel: w1522 -> [w1525 _]
                          frame #0 {
                            n851 = Build Array("T-RISE") -> (w1529:string[])
                            n852 = Build Array(w1527) -> (w1528:dbl[])
                            n853 = TDMS Write(0:w1525, 5:"TEST PASS", 7:w1529, 9:w1528) -> (15:w1531:errorcluster)  [unwired: 2 in, 3 out]
                            n854 = local write "data file error"(w1531) -> ()
                          }
                          frame #1 {
                            n855 = Bundle(cluster=w1532, "STATUS"="STOP") -> (w1534:T4)  [unwired: 2 in]
                            n856 = local write "LAB01-2 (RESULT)"(TRUE) -> ()
                            n857 = local write "LAB01-2 (DISP)"(w1534) -> ()
                          }
                        }
                      }
                      frame False {
                      }
                    }
                  }
                }
              }
              frame #2 {
                # "LAB02-1"
                n858 = Equal?(x=w1536, y=2) -> (x = y?=w1540:bool)
                n859 = local read "LAB02-1 (DISP)"() -> (w1542:T4)
                n860 = Unbundle(w1542) -> ("STATUS"=w1543:string)  [unwired: 2 out]
                n861 = Equal?(x=w1543, y="RUN") -> (x = y?=w1539:bool)
                n862 = And(x=w1539, y=w1540) -> (x .and. y?=w1538:bool)
                n863 = case shown="True" w1538 {
                  tunnel: w1542 -> [_ w1546]
                  tunnel: w1537 -> [_ w1549]
                  frame False {
                  }
                  frame True {
                    n864 = local read "LAB02-1 (SET)"() -> (w1548:T5)
                    n865 = local read "LAB02-1 (TDMS)"() -> (w1545:refnum<k34>)
                    n866 = Unbundle(w1546) -> ("CYCLE"=w1550:dbl)  [unwired: 2 out]
                    n867 = Unbundle(w1548) -> ("T-RISE mins"=w1547:dbl)  [unwired: 4 out]
                    n868 = Greater Or Equal?(x=w1550, y=w1549) -> (x >= y?=w1551:bool)
                    n869 = case shown="True" w1551 {
                      tunnel: w1547 -> [w1554 _]
                      tunnel: w1546 -> [w1553 _]
                      tunnel: w1545 -> [w1552 _]
                      frame True {
                        n870 = stacked-sequence {
                          tunnel: w1554 -> [w1557 _]
                          tunnel: w1553 -> [_ w1562]
                          tunnel: w1552 -> [w1555 _]
                          frame #0 {
                            n871 = Build Array("T-RISE") -> (w1559:string[])
                            n872 = Build Array(w1557) -> (w1558:dbl[])
                            n873 = TDMS Write(0:w1555, 5:"TEST PASS", 7:w1559, 9:w1558) -> (15:w1561:errorcluster)  [unwired: 2 in, 3 out]
                            n874 = local write "data file error"(w1561) -> ()
                          }
                          frame #1 {
                            n875 = Bundle(cluster=w1562, "STATUS"="STOP") -> (w1564:T4)  [unwired: 2 in]
                            n876 = local write "LAB02-1 (RESULT)"(TRUE) -> ()
                            n877 = local write "LAB02-1 (DISP)"(w1564) -> ()
                          }
                        }
                      }
                      frame False {
                      }
                    }
                  }
                }
              }
              frame #3 {
                # "LAB02-2"
                n878 = Equal?(x=w1566, y=2) -> (x = y?=w1570:bool)
                n879 = local read "LAB02-2 (DISP)"() -> (w1572:T4)
                n880 = Unbundle(w1572) -> ("STATUS"=w1573:string)  [unwired: 2 out]
                n881 = Equal?(x=w1573, y="RUN") -> (x = y?=w1569:bool)
                n882 = And(x=w1569, y=w1570) -> (x .and. y?=w1568:bool)
                n883 = case shown="True" w1568 {
                  tunnel: w1572 -> [_ w1576]
                  tunnel: w1567 -> [_ w1579]
                  frame False {
                  }
                  frame True {
                    n884 = local read "LAB02-2 (SET)"() -> (w1578:T5)
                    n885 = local read "LAB02-2 (TDMS)"() -> (w1575:refnum<k34>)
                    n886 = Unbundle(w1576) -> ("CYCLE"=w1580:dbl)  [unwired: 2 out]
                    n887 = Unbundle(w1578) -> ("T-RISE mins"=w1577:dbl)  [unwired: 4 out]
                    n888 = Greater Or Equal?(x=w1580, y=w1579) -> (x >= y?=w1581:bool)
                    n889 = case shown="True" w1581 {
                      tunnel: w1577 -> [w1584 _]
                      tunnel: w1576 -> [w1583 _]
                      tunnel: w1575 -> [w1582 _]
                      frame True {
                        n890 = stacked-sequence {
                          tunnel: w1584 -> [w1587 _]
                          tunnel: w1583 -> [_ w1592]
                          tunnel: w1582 -> [w1585 _]
                          frame #0 {
                            n891 = Build Array("T-RISE") -> (w1589:string[])
                            n892 = Build Array(w1587) -> (w1588:dbl[])
                            n893 = TDMS Write(0:w1585, 5:"TEST PASS", 7:w1589, 9:w1588) -> (15:w1591:errorcluster)  [unwired: 2 in, 3 out]
                            n894 = local write "data file error"(w1591) -> ()
                          }
                          frame #1 {
                            n895 = Bundle(cluster=w1592, "STATUS"="STOP") -> (w1594:T4)  [unwired: 2 in]
                            n896 = local write "LAB02-2 (RESULT)"(TRUE) -> ()
                            n897 = local write "LAB02-2 (DISP)"(w1594) -> ()
                          }
                        }
                      }
                      frame False {
                      }
                    }
                  }
                }
              }
              frame #4 {
                # "LAB03-1"
                n898 = Equal?(x=w1596, y=2) -> (x = y?=w1600:bool)
                n899 = local read "LAB03-1 (DISP)"() -> (w1602:T4)
                n900 = Unbundle(w1602) -> ("STATUS"=w1603:string)  [unwired: 2 out]
                n901 = Equal?(x=w1603, y="RUN") -> (x = y?=w1599:bool)
                n902 = And(x=w1599, y=w1600) -> (x .and. y?=w1598:bool)
                n903 = case shown="True" w1598 {
                  tunnel: w1602 -> [_ w1606]
                  tunnel: w1597 -> [_ w1609]
                  frame False {
                  }
                  frame True {
                    n904 = local read "LAB03-1 (SET)"() -> (w1608:T5)
                    n905 = local read "LAB03-1 (TDMS)"() -> (w1605:refnum<k34>)
                    n906 = Unbundle(w1606) -> ("CYCLE"=w1610:dbl)  [unwired: 2 out]
                    n907 = Unbundle(w1608) -> ("T-RISE mins"=w1607:dbl)  [unwired: 4 out]
                    n908 = Greater Or Equal?(x=w1610, y=w1609) -> (x >= y?=w1611:bool)
                    n909 = case shown="True" w1611 {
                      tunnel: w1607 -> [w1614 _]
                      tunnel: w1606 -> [w1613 _]
                      tunnel: w1605 -> [w1612 _]
                      frame True {
                        n910 = stacked-sequence {
                          tunnel: w1614 -> [w1617 _]
                          tunnel: w1613 -> [_ w1622]
                          tunnel: w1612 -> [w1615 _]
                          frame #0 {
                            n911 = Build Array("T-RISE") -> (w1619:string[])
                            n912 = Build Array(w1617) -> (w1618:dbl[])
                            n913 = TDMS Write(0:w1615, 5:"TEST PASS", 7:w1619, 9:w1618) -> (15:w1621:errorcluster)  [unwired: 2 in, 3 out]
                            n914 = local write "data file error"(w1621) -> ()
                          }
                          frame #1 {
                            n915 = Bundle(cluster=w1622, "STATUS"="STOP") -> (w1624:T4)  [unwired: 2 in]
                            n916 = local write "LAB03-1 (RESULT)"(TRUE) -> ()
                            n917 = local write "LAB03-1 (DISP)"(w1624) -> ()
                          }
                        }
                      }
                      frame False {
                      }
                    }
                  }
                }
              }
              frame #5 {
                # "LAB03-2"
                n918 = Equal?(x=w1626, y=2) -> (x = y?=w1630:bool)
                n919 = local read "LAB03-2 (DISP)"() -> (w1632:T4)
                n920 = Unbundle(w1632) -> ("STATUS"=w1633:string)  [unwired: 2 out]
                n921 = Equal?(x=w1633, y="RUN") -> (x = y?=w1629:bool)
                n922 = And(x=w1629, y=w1630) -> (x .and. y?=w1628:bool)
                n923 = case shown="True" w1628 {
                  tunnel: w1632 -> [_ w1636]
                  tunnel: w1627 -> [_ w1639]
                  frame False {
                  }
                  frame True {
                    n924 = local read "LAB03-2 (SET)"() -> (w1638:T5)
                    n925 = local read "LAB03-2 (TDMS)"() -> (w1635:refnum<k34>)
                    n926 = Unbundle(w1636) -> ("CYCLE"=w1640:dbl)  [unwired: 2 out]
                    n927 = Unbundle(w1638) -> ("T-RISE mins"=w1637:dbl)  [unwired: 4 out]
                    n928 = Greater Or Equal?(x=w1640, y=w1639) -> (x >= y?=w1641:bool)
                    n929 = case shown="True" w1641 {
                      tunnel: w1637 -> [w1644 _]
                      tunnel: w1636 -> [w1643 _]
                      tunnel: w1635 -> [w1642 _]
                      frame True {
                        n930 = stacked-sequence {
                          tunnel: w1644 -> [w1647 _]
                          tunnel: w1643 -> [_ w1652]
                          tunnel: w1642 -> [w1645 _]
                          frame #0 {
                            n931 = Build Array("T-RISE") -> (w1649:string[])
                            n932 = Build Array(w1647) -> (w1648:dbl[])
                            n933 = TDMS Write(0:w1645, 5:"TEST PASS", 7:w1649, 9:w1648) -> (15:w1651:errorcluster)  [unwired: 2 in, 3 out]
                            n934 = local write "data file error"(w1651) -> ()
                          }
                          frame #1 {
                            n935 = Bundle(cluster=w1652, "STATUS"="STOP") -> (w1654:T4)  [unwired: 2 in]
                            n936 = local write "LAB03-2 (RESULT)"(TRUE) -> ()
                            n937 = local write "LAB03-2 (DISP)"(w1654) -> ()
                          }
                        }
                      }
                      frame False {
                      }
                    }
                  }
                }
              }
              frame #6 {
                # "LAB04-1"
                n938 = Equal?(x=w1656, y=2) -> (x = y?=w1660:bool)
                n939 = local read "LAB04-1 (DISP)"() -> (w1662:T4)
                n940 = Unbundle(w1662) -> ("STATUS"=w1663:string)  [unwired: 2 out]
                n941 = Equal?(x=w1663, y="RUN") -> (x = y?=w1659:bool)
                n942 = And(x=w1659, y=w1660) -> (x .and. y?=w1658:bool)
                n943 = case shown="True" w1658 {
                  tunnel: w1662 -> [_ w1666]
                  tunnel: w1657 -> [_ w1669]
                  frame False {
                  }
                  frame True {
                    n944 = local read "LAB04-1 (SET)"() -> (w1668:T5)
                    n945 = local read "LAB04-1 (TDMS)"() -> (w1665:refnum<k34>)
                    n946 = Unbundle(w1666) -> ("CYCLE"=w1670:dbl)  [unwired: 2 out]
                    n947 = Unbundle(w1668) -> ("T-RISE mins"=w1667:dbl)  [unwired: 4 out]
                    n948 = Greater Or Equal?(x=w1670, y=w1669) -> (x >= y?=w1671:bool)
                    n949 = case shown="True" w1671 {
                      tunnel: w1667 -> [w1674 _]
                      tunnel: w1666 -> [w1673 _]
                      tunnel: w1665 -> [w1672 _]
                      frame True {
                        n950 = stacked-sequence {
                          tunnel: w1674 -> [w1677 _]
                          tunnel: w1673 -> [_ w1682]
                          tunnel: w1672 -> [w1675 _]
                          frame #0 {
                            n951 = Build Array("T-RISE") -> (w1679:string[])
                            n952 = Build Array(w1677) -> (w1678:dbl[])
                            n953 = TDMS Write(0:w1675, 5:"TEST PASS", 7:w1679, 9:w1678) -> (15:w1681:errorcluster)  [unwired: 2 in, 3 out]
                            n954 = local write "data file error"(w1681) -> ()
                          }
                          frame #1 {
                            n955 = Bundle(cluster=w1682, "STATUS"="STOP") -> (w1684:T4)  [unwired: 2 in]
                            n956 = local write "LAB04-1 (RESULT)"(TRUE) -> ()
                            n957 = local write "LAB04-1 (DISP)"(w1684) -> ()
                          }
                        }
                      }
                      frame False {
                      }
                    }
                  }
                }
              }
              frame #7 {
                # "LAB04-2"
                n958 = Equal?(x=w1686, y=2) -> (x = y?=w1690:bool)
                n959 = local read "LAB04-2 (DISP)"() -> (w1692:T4)
                n960 = Unbundle(w1692) -> ("STATUS"=w1693:string)  [unwired: 2 out]
                n961 = Equal?(x=w1693, y="RUN") -> (x = y?=w1689:bool)
                n962 = And(x=w1689, y=w1690) -> (x .and. y?=w1688:bool)
                n963 = case shown="True" w1688 {
                  tunnel: w1692 -> [_ w1696]
                  tunnel: w1687 -> [_ w1699]
                  frame False {
                  }
                  frame True {
                    n964 = local read "LAB04-2 (SET)"() -> (w1698:T5)
                    n965 = local read "LAB04-2 (TDMS)"() -> (w1695:refnum<k34>)
                    n966 = Unbundle(w1696) -> ("CYCLE"=w1700:dbl)  [unwired: 2 out]
                    n967 = Unbundle(w1698) -> ("T-RISE mins"=w1697:dbl)  [unwired: 4 out]
                    n968 = Greater Or Equal?(x=w1700, y=w1699) -> (x >= y?=w1701:bool)
                    n969 = case shown="True" w1701 {
                      tunnel: w1697 -> [w1704 _]
                      tunnel: w1696 -> [w1703 _]
                      tunnel: w1695 -> [w1702 _]
                      frame True {
                        n970 = stacked-sequence {
                          tunnel: w1704 -> [w1707 _]
                          tunnel: w1703 -> [_ w1712]
                          tunnel: w1702 -> [w1705 _]
                          frame #0 {
                            n971 = Build Array("T-RISE") -> (w1709:string[])
                            n972 = Build Array(w1707) -> (w1708:dbl[])
                            n973 = TDMS Write(0:w1705, 5:"TEST PASS", 7:w1709, 9:w1708) -> (15:w1711:errorcluster)  [unwired: 2 in, 3 out]
                            n974 = local write "data file error"(w1711) -> ()
                          }
                          frame #1 {
                            n975 = Bundle(cluster=w1712, "STATUS"="STOP") -> (w1714:T4)  [unwired: 2 in]
                            n976 = local write "LAB04-2 (RESULT)"(TRUE) -> ()
                            n977 = local write "LAB04-2 (DISP)"(w1714) -> ()
                          }
                        }
                      }
                      frame False {
                      }
                    }
                  }
                }
              }
              frame #8 {
                # "LAB05-1"
                n978 = Equal?(x=w1716, y=2) -> (x = y?=w1720:bool)
                n979 = local read "LAB05-1 (DISP)"() -> (w1722:T4)
                n980 = Unbundle(w1722) -> ("STATUS"=w1723:string)  [unwired: 2 out]
                n981 = Equal?(x=w1723, y="RUN") -> (x = y?=w1719:bool)
                n982 = And(x=w1719, y=w1720) -> (x .and. y?=w1718:bool)
                n983 = case shown="True" w1718 {
                  tunnel: w1722 -> [_ w1726]
                  tunnel: w1717 -> [_ w1729]
                  frame False {
                  }
                  frame True {
                    n984 = local read "LAB05-1 (SET)"() -> (w1728:T5)
                    n985 = local read "LAB05-1 (TDMS)"() -> (w1725:refnum<k34>)
                    n986 = Unbundle(w1726) -> ("CYCLE"=w1730:dbl)  [unwired: 2 out]
                    n987 = Unbundle(w1728) -> ("T-RISE mins"=w1727:dbl)  [unwired: 4 out]
                    n988 = Greater Or Equal?(x=w1730, y=w1729) -> (x >= y?=w1731:bool)
                    n989 = case shown="True" w1731 {
                      tunnel: w1727 -> [w1734 _]
                      tunnel: w1726 -> [w1733 _]
                      tunnel: w1725 -> [w1732 _]
                      frame True {
                        n990 = stacked-sequence {
                          tunnel: w1734 -> [w1737 _]
                          tunnel: w1733 -> [_ w1742]
                          tunnel: w1732 -> [w1735 _]
                          frame #0 {
                            n991 = Build Array("T-RISE") -> (w1739:string[])
                            n992 = Build Array(w1737) -> (w1738:dbl[])
                            n993 = TDMS Write(0:w1735, 5:"TEST PASS", 7:w1739, 9:w1738) -> (15:w1741:errorcluster)  [unwired: 2 in, 3 out]
                            n994 = local write "data file error"(w1741) -> ()
                          }
                          frame #1 {
                            n995 = Bundle(cluster=w1742, "STATUS"="STOP") -> (w1744:T4)  [unwired: 2 in]
                            n996 = local write "LAB05-1 (RESULT)"(TRUE) -> ()
                            n997 = local write "LAB05-1 (DISP)"(w1744) -> ()
                          }
                        }
                      }
                      frame False {
                      }
                    }
                  }
                }
              }
              frame #9 {
                # "LAB05-2"
                n998 = Equal?(x=w1746, y=2) -> (x = y?=w1750:bool)
                n999 = local read "LAB05-2 (DISP)"() -> (w1752:T4)
                n1000 = Unbundle(w1752) -> ("STATUS"=w1753:string)  [unwired: 2 out]
                n1001 = Equal?(x=w1753, y="RUN") -> (x = y?=w1749:bool)
                n1002 = And(x=w1749, y=w1750) -> (x .and. y?=w1748:bool)
                n1003 = case shown="True" w1748 {
                  tunnel: w1752 -> [_ w1756]
                  tunnel: w1747 -> [_ w1759]
                  frame False {
                  }
                  frame True {
                    n1004 = local read "LAB05-2 (SET)"() -> (w1758:T5)
                    n1005 = local read "LAB05-2 (TDMS)"() -> (w1755:refnum<k34>)
                    n1006 = Unbundle(w1756) -> ("CYCLE"=w1760:dbl)  [unwired: 2 out]
                    n1007 = Unbundle(w1758) -> ("T-RISE mins"=w1757:dbl)  [unwired: 4 out]
                    n1008 = Greater Or Equal?(x=w1760, y=w1759) -> (x >= y?=w1761:bool)
                    n1009 = case shown="True" w1761 {
                      tunnel: w1757 -> [w1764 _]
                      tunnel: w1756 -> [w1763 _]
                      tunnel: w1755 -> [w1762 _]
                      frame True {
                        n1010 = stacked-sequence {
                          tunnel: w1764 -> [w1767 _]
                          tunnel: w1763 -> [_ w1772]
                          tunnel: w1762 -> [w1765 _]
                          frame #0 {
                            n1011 = Build Array("T-RISE") -> (w1769:string[])
                            n1012 = Build Array(w1767) -> (w1768:dbl[])
                            n1013 = TDMS Write(0:w1765, 5:"TEST PASS", 7:w1769, 9:w1768) -> (15:w1771:errorcluster)  [unwired: 2 in, 3 out]
                            n1014 = local write "data file error"(w1771) -> ()
                          }
                          frame #1 {
                            n1015 = Bundle(cluster=w1772, "STATUS"="STOP") -> (w1774:T4)  [unwired: 2 in]
                            n1016 = local write "LAB05-2 (RESULT)"(TRUE) -> ()
                            n1017 = local write "LAB05-2 (DISP)"(w1774) -> ()
                          }
                        }
                      }
                      frame False {
                      }
                    }
                  }
                }
              }
            }
          }
          frame #6 {
            # "disable functions"
            n1018 = stacked-sequence {
              tunnel: w1785 -> [w1795 _ w1845]
              tunnel: w1784 -> [w1794 _ w1844]
              tunnel: w1783 -> [w1793 _ w1843]
              tunnel: w1782 -> [w1792 _ w1842]
              tunnel: w1781 -> [w1791 _ w1841]
              tunnel: w1780 -> [_ w1815 w1840]
              tunnel: w1779 -> [_ w1814 w1839]
              tunnel: w1778 -> [_ w1813 w1838]
              tunnel: w1777 -> [_ w1812 w1837]
              tunnel: w1776 -> [_ w1811 w1836]
              frame #0 {
                n1019 = Select(t=2, s=w1792, f=0) -> (s? t:f=w1787:i32)
                n1020 = Select(t=2, s=w1793, f=0) -> (s? t:f=w1788:i32)
                n1021 = Select(t=2, s=w1791, f=0) -> (s? t:f=w1786:i32)
                n1022 = Select(t=2, s=w1795, f=0) -> (s? t:f=w1790:i32)
                n1023 = Select(t=2, s=w1794, f=0) -> (s? t:f=w1789:i32)
                n1024 = property on="LAB02-2 SELECT" class="RadioBtnsControl (strict)"("DisabledEnum"=w1787) -> ()  [unwired: 2 in, 2 out]
                n1025 = property on="LAB02-1 SELECT" class="RadioBtnsControl (strict)"("DisabledEnum"=w1788) -> ()  [unwired: 2 in, 2 out]
                n1026 = property on="LAB03-1 SELECT" class="RadioBtnsControl (strict)"("DisabledEnum"=w1786) -> ()  [unwired: 2 in, 2 out]
                n1027 = property on="LAB01-1 SELECT" class="RadioBtnsControl (strict)"("DisabledEnum"=w1790) -> ()  [unwired: 2 in, 2 out]
                n1028 = property on="LAB01-2 SELECT" class="RadioBtnsControl (strict)"("DisabledEnum"=w1789) -> ()  [unwired: 2 in, 2 out]
                n1029 = property on="LAB01-2 (RESULT)" class="Bool (strict)"("DisabledEnum"=w1789) -> ()  [unwired: 2 in, 2 out]
                n1030 = property on="LAB02-1 (RESULT)" class="Bool (strict)"("DisabledEnum"=w1788) -> ()  [unwired: 2 in, 2 out]
                n1031 = property on="LAB01-1 (RESULT)" class="Bool (strict)"("DisabledEnum"=w1790) -> ()  [unwired: 2 in, 2 out]
                n1032 = property on="LAB02-2 (RESULT)" class="Bool (strict)"("DisabledEnum"=w1787) -> ()  [unwired: 2 in, 2 out]
                n1033 = property on="LAB03-1 (RESULT)" class="Bool (strict)"("DisabledEnum"=w1786) -> ()  [unwired: 2 in, 2 out]
              }
              frame #1 {
                n1034 = Select(t=2, s=w1811, f=0) -> (s? t:f=w1806:i32)
                n1035 = Select(t=2, s=w1812, f=0) -> (s? t:f=w1807:i32)
                n1036 = Select(t=2, s=w1815, f=0) -> (s? t:f=w1810:i32)
                n1037 = Select(t=2, s=w1814, f=0) -> (s? t:f=w1809:i32)
                n1038 = Select(t=2, s=w1813, f=0) -> (s? t:f=w1808:i32)
                n1039 = property on="LAB05-2 SELECT" class="RadioBtnsControl (strict)"("DisabledEnum"=w1806) -> ()  [unwired: 2 in, 2 out]
                n1040 = property on="LAB05-1 SELECT" class="RadioBtnsControl (strict)"("DisabledEnum"=w1807) -> ()  [unwired: 2 in, 2 out]
                n1041 = property on="LAB03-2 SELECT" class="RadioBtnsControl (strict)"("DisabledEnum"=w1810) -> ()  [unwired: 2 in, 2 out]
                n1042 = property on="LAB04-1 SELECT" class="RadioBtnsControl (strict)"("DisabledEnum"=w1809) -> ()  [unwired: 2 in, 2 out]
                n1043 = property on="LAB04-2 SELECT" class="RadioBtnsControl (strict)"("DisabledEnum"=w1808) -> ()  [unwired: 2 in, 2 out]
                n1044 = property on="LAB03-2 (RESULT)" class="Bool (strict)"("DisabledEnum"=w1810) -> ()  [unwired: 2 in, 2 out]
                n1045 = property on="LAB05-2 (RESULT)" class="Bool (strict)"("DisabledEnum"=w1806) -> ()  [unwired: 2 in, 2 out]
                n1046 = property on="LAB05-1 (RESULT)" class="Bool (strict)"("DisabledEnum"=w1807) -> ()  [unwired: 2 in, 2 out]
                n1047 = property on="LAB04-2 (RESULT)" class="Bool (strict)"("DisabledEnum"=w1808) -> ()  [unwired: 2 in, 2 out]
                n1048 = property on="LAB04-1 (RESULT)" class="Bool (strict)"("DisabledEnum"=w1809) -> ()  [unwired: 2 in, 2 out]
              }
              frame #2 {
                # "disable calibrate if any test running"
                n1049 = Or(x=w1837, y=w1836) -> (x .or. y?=w1830:bool)
                n1050 = Or(x=w1839, y=w1838) -> (x .or. y?=w1832:bool)
                n1051 = Or(x=w1843, y=w1842) -> (x .or. y?=w1834:bool)
                n1052 = Or(x=w1841, y=w1840) -> (x .or. y?=w1833:bool)
                n1053 = Or(x=w1845, y=w1844) -> (x .or. y?=w1835:bool)
                n1054 = Or(x=w1833, y=w1832) -> (x .or. y?=w1831:bool)
                n1055 = Or(x=w1835, y=w1834) -> (x .or. y?=w1829:bool)
                n1056 = Or(x=w1831, y=w1830) -> (x .or. y?=w1828:bool)
                n1057 = Or(x=w1829, y=w1828) -> (x .or. y?=w1827:bool)
                n1058 = case shown="False" w1827 {
                  tunnel: [0 2] -> w1826
                  frame False {
                  }
                  frame True {
                  }
                }
                n1059 = property on="CALIBRATE" class="Bool (strict)"("DisabledEnum"=w1826) -> ()  [unwired: 2 in, 2 out]
              }
            }
          }
          frame #7 {
            # "end test & close test files"
            n1060 = stacked-sequence {
              tunnel: w1848 -> [w1849 _ _ _ _ _ _ _ _ _]
              frame #0 {
                # "LAB01-1"
                n1061 = case shown="True" w1849 {
                  frame False {
                  }
                  frame True {
                    n1062 = local read "LAB01-1 (DISP)"() -> (w1852:T4)
                    n1063 = local read "LAB01-1 (TDMS)"() -> (w1851:refnum<k34>)
                    n1064 = Unbundle(w1852) -> ("STATUS"=w1850:string)  [unwired: 2 out]
                    n1065 = Not Equal?(x=w1850, y="RUN") -> (x != y?=w1853:bool)
                    n1066 = case shown="True" w1853 {
                      tunnel: w1852 -> [_ w1856]
                      tunnel: w1851 -> [_ w1855]
                      frame False {
                      }
                      frame True {
                        n1067 = stacked-sequence {
                          tunnel: w1856 -> [w1858 _]
                          tunnel: w1855 -> [_ w1860]
                          frame #0 {
                            (unwired) "END"
                            n1068 = Bundle(cluster=w1858) -> (w1857:T4)  [unwired: 3 in]
                            n1069 = local write "LAB01-1 (DISP)"(w1857) -> ()
                            n1070 = local write "LAB01-1RUN"(FALSE) -> ()
                          }
                          frame #1 {
                            n1071 = TDMS Close(11:w1860) -> (0:w1861:errorcluster)  [unwired: 1 in, 1 out]
                            n1072 = local write "data file error"(w1861) -> ()
                          }
                        }
                      }
                    }
                  }
                }
              }
              frame #1 {
                # "LAB01-2"
                n1073 = local read "LAB01-2 (DISP)"() -> (w1863:T4)
                n1074 = local read "LAB01-2 (TDMS)"() -> (w1862:refnum<k34>)
                n1075 = Unbundle(w1863) -> ("STATUS"=w1864:string)  [unwired: 2 out]
                n1076 = Equal?(x=w1864, y="STOP") -> (x = y?=w1865:bool)
                n1077 = case shown="True" w1865 {
                  tunnel: w1863 -> [_ w1868]
                  tunnel: w1862 -> [_ w1867]
                  frame False {
                  }
                  frame True {
                    n1078 = stacked-sequence {
                      tunnel: w1868 -> [w1870 _]
                      tunnel: w1867 -> [_ w1873]
                      frame #0 {
                        n1079 = Bundle(cluster=w1870, "STATUS"="END") -> (w1871:T4)  [unwired: 2 in]
                        n1080 = local write "LAB01-2 RUN"(FALSE) -> ()
                        n1081 = local write "LAB01-2 (DISP)"(w1871) -> ()
                      }
                      frame #1 {
                        n1082 = TDMS Close(11:w1873) -> (0:w1874:errorcluster)  [unwired: 1 in, 1 out]
                        n1083 = local write "data file error"(w1874) -> ()
                      }
                    }
                  }
                }
              }
              frame #2 {
                # "LAB02-1"
                n1084 = local read "LAB02-1 (DISP)"() -> (w1876:T4)
                n1085 = local read "LAB02-1 (TDMS)"() -> (w1875:refnum<k34>)
                n1086 = Unbundle(w1876) -> ("STATUS"=w1877:string)  [unwired: 2 out]
                n1087 = Equal?(x=w1877, y="STOP") -> (x = y?=w1878:bool)
                n1088 = case shown="True" w1878 {
                  tunnel: w1876 -> [_ w1881]
                  tunnel: w1875 -> [_ w1880]
                  frame False {
                  }
                  frame True {
                    n1089 = stacked-sequence {
                      tunnel: w1881 -> [w1883 _]
                      tunnel: w1880 -> [_ w1886]
                      frame #0 {
                        n1090 = Bundle(cluster=w1883, "STATUS"="END") -> (w1884:T4)  [unwired: 2 in]
                        n1091 = local write "LAB02-1 RUN"(FALSE) -> ()
                        n1092 = local write "LAB02-1 (DISP)"(w1884) -> ()
                      }
                      frame #1 {
                        n1093 = TDMS Close(11:w1886) -> (0:w1887:errorcluster)  [unwired: 1 in, 1 out]
                        n1094 = local write "data file error"(w1887) -> ()
                      }
                    }
                  }
                }
              }
              frame #3 {
                # "LAB02-2"
                n1095 = local read "LAB02-2 (DISP)"() -> (w1889:T4)
                n1096 = local read "LAB02-2 (TDMS)"() -> (w1888:refnum<k34>)
                n1097 = Unbundle(w1889) -> ("STATUS"=w1890:string)  [unwired: 2 out]
                n1098 = Equal?(x=w1890, y="STOP") -> (x = y?=w1891:bool)
                n1099 = case shown="True" w1891 {
                  tunnel: w1889 -> [_ w1894]
                  tunnel: w1888 -> [_ w1893]
                  frame False {
                  }
                  frame True {
                    n1100 = stacked-sequence {
                      tunnel: w1894 -> [w1896 _]
                      tunnel: w1893 -> [_ w1899]
                      frame #0 {
                        n1101 = Bundle(cluster=w1896, "STATUS"="END") -> (w1897:T4)  [unwired: 2 in]
                        n1102 = local write "LAB02-2 RUN"(FALSE) -> ()
                        n1103 = local write "LAB02-2 (DISP)"(w1897) -> ()
                      }
                      frame #1 {
                        n1104 = TDMS Close(11:w1899) -> (0:w1900:errorcluster)  [unwired: 1 in, 1 out]
                        n1105 = local write "data file error"(w1900) -> ()
                      }
                    }
                  }
                }
              }
              frame #4 {
                # "LAB03-1"
                n1106 = local read "LAB03-1 (DISP)"() -> (w1902:T4)
                n1107 = local read "LAB03-1 (TDMS)"() -> (w1901:refnum<k34>)
                n1108 = Unbundle(w1902) -> ("STATUS"=w1903:string)  [unwired: 2 out]
                n1109 = Equal?(x=w1903, y="STOP") -> (x = y?=w1904:bool)
                n1110 = case shown="True" w1904 {
                  tunnel: w1902 -> [_ w1907]
                  tunnel: w1901 -> [_ w1906]
                  frame False {
                  }
                  frame True {
                    n1111 = stacked-sequence {
                      tunnel: w1907 -> [w1909 _]
                      tunnel: w1906 -> [_ w1912]
                      frame #0 {
                        n1112 = Bundle(cluster=w1909, "STATUS"="END") -> (w1910:T4)  [unwired: 2 in]
                        n1113 = local write "LAB03-1 RUN"(FALSE) -> ()
                        n1114 = local write "LAB03-1 (DISP)"(w1910) -> ()
                      }
                      frame #1 {
                        n1115 = TDMS Close(11:w1912) -> (0:w1913:errorcluster)  [unwired: 1 in, 1 out]
                        n1116 = local write "data file error"(w1913) -> ()
                      }
                    }
                  }
                }
              }
              frame #5 {
                # "LAB03-2"
                n1117 = local read "LAB03-2 (DISP)"() -> (w1915:T4)
                n1118 = local read "LAB03-2 (TDMS)"() -> (w1914:refnum<k34>)
                n1119 = Unbundle(w1915) -> ("STATUS"=w1916:string)  [unwired: 2 out]
                n1120 = Equal?(x=w1916, y="STOP") -> (x = y?=w1917:bool)
                n1121 = case shown="True" w1917 {
                  tunnel: w1915 -> [_ w1920]
                  tunnel: w1914 -> [_ w1919]
                  frame False {
                  }
                  frame True {
                    n1122 = stacked-sequence {
                      tunnel: w1920 -> [w1922 _]
                      tunnel: w1919 -> [_ w1925]
                      frame #0 {
                        n1123 = Bundle(cluster=w1922, "STATUS"="END") -> (w1923:T4)  [unwired: 2 in]
                        n1124 = local write "LAB03-2 RUN"(FALSE) -> ()
                        n1125 = local write "LAB03-2 (DISP)"(w1923) -> ()
                      }
                      frame #1 {
                        n1126 = TDMS Close(11:w1925) -> (0:w1926:errorcluster)  [unwired: 1 in, 1 out]
                        n1127 = local write "data file error"(w1926) -> ()
                      }
                    }
                  }
                }
              }
              frame #6 {
                # "LAB04-1"
                n1128 = local read "LAB04-1 (DISP)"() -> (w1928:T4)
                n1129 = local read "LAB04-1 (TDMS)"() -> (w1927:refnum<k34>)
                n1130 = Unbundle(w1928) -> ("STATUS"=w1929:string)  [unwired: 2 out]
                n1131 = Equal?(x=w1929, y="STOP") -> (x = y?=w1930:bool)
                n1132 = case shown="True" w1930 {
                  tunnel: w1928 -> [_ w1933]
                  tunnel: w1927 -> [_ w1932]
                  frame False {
                  }
                  frame True {
                    n1133 = stacked-sequence {
                      tunnel: w1933 -> [w1935 _]
                      tunnel: w1932 -> [_ w1938]
                      frame #0 {
                        n1134 = Bundle(cluster=w1935, "STATUS"="END") -> (w1936:T4)  [unwired: 2 in]
                        n1135 = local write "LAB04-1 RUN"(FALSE) -> ()
                        n1136 = local write "LAB04-1 (DISP)"(w1936) -> ()
                      }
                      frame #1 {
                        n1137 = TDMS Close(11:w1938) -> (0:w1939:errorcluster)  [unwired: 1 in, 1 out]
                        n1138 = local write "data file error"(w1939) -> ()
                      }
                    }
                  }
                }
              }
              frame #7 {
                # "LAB04-2"
                n1139 = local read "LAB04-2 (DISP)"() -> (w1941:T4)
                n1140 = local read "LAB04-2 (TDMS)"() -> (w1940:refnum<k34>)
                n1141 = Unbundle(w1941) -> ("STATUS"=w1942:string)  [unwired: 2 out]
                n1142 = Equal?(x=w1942, y="STOP") -> (x = y?=w1943:bool)
                n1143 = case shown="True" w1943 {
                  tunnel: w1941 -> [_ w1946]
                  tunnel: w1940 -> [_ w1945]
                  frame False {
                  }
                  frame True {
                    n1144 = stacked-sequence {
                      tunnel: w1946 -> [w1948 _]
                      tunnel: w1945 -> [_ w1951]
                      frame #0 {
                        n1145 = Bundle(cluster=w1948, "STATUS"="END") -> (w1949:T4)  [unwired: 2 in]
                        n1146 = local write "LAB04-2 RUN"(FALSE) -> ()
                        n1147 = local write "LAB04-2 (DISP)"(w1949) -> ()
                      }
                      frame #1 {
                        n1148 = TDMS Close(11:w1951) -> (0:w1952:errorcluster)  [unwired: 1 in, 1 out]
                        n1149 = local write "data file error"(w1952) -> ()
                      }
                    }
                  }
                }
              }
              frame #8 {
                # "LAB05-1"
                n1150 = local read "LAB05-1 (DISP)"() -> (w1954:T4)
                n1151 = local read "LAB05-1 (TDMS)"() -> (w1953:refnum<k34>)
                n1152 = Unbundle(w1954) -> ("STATUS"=w1955:string)  [unwired: 2 out]
                n1153 = Equal?(x=w1955, y="STOP") -> (x = y?=w1956:bool)
                n1154 = case shown="True" w1956 {
                  tunnel: w1954 -> [_ w1959]
                  tunnel: w1953 -> [_ w1958]
                  frame False {
                  }
                  frame True {
                    n1155 = stacked-sequence {
                      tunnel: w1959 -> [w1961 _]
                      tunnel: w1958 -> [_ w1964]
                      frame #0 {
                        n1156 = Bundle(cluster=w1961, "STATUS"="END") -> (w1962:T4)  [unwired: 2 in]
                        n1157 = local write "LAB05-1 RUN"(FALSE) -> ()
                        n1158 = local write "LAB05-1 (DISP)"(w1962) -> ()
                      }
                      frame #1 {
                        n1159 = TDMS Close(11:w1964) -> (0:w1965:errorcluster)  [unwired: 1 in, 1 out]
                        n1160 = local write "data file error"(w1965) -> ()
                      }
                    }
                  }
                }
              }
              frame #9 {
                # "LAB05-2"
                n1161 = local read "LAB05-2 (DISP)"() -> (w1967:T4)
                n1162 = local read "LAB05-2 (TDMS)"() -> (w1966:refnum<k34>)
                n1163 = Unbundle(w1967) -> ("STATUS"=w1968:string)  [unwired: 2 out]
                n1164 = Equal?(x=w1968, y="STOP") -> (x = y?=w1969:bool)
                n1165 = case shown="True" w1969 {
                  tunnel: w1967 -> [_ w1972]
                  tunnel: w1966 -> [_ w1971]
                  frame False {
                  }
                  frame True {
                    n1166 = stacked-sequence {
                      tunnel: w1972 -> [w1974 _]
                      tunnel: w1971 -> [_ w1977]
                      frame #0 {
                        n1167 = Bundle(cluster=w1974, "STATUS"="END") -> (w1975:T4)  [unwired: 2 in]
                        n1168 = local write "LAB05-2 RUN"(FALSE) -> ()
                        n1169 = local write "LAB05-2 (DISP)"(w1975) -> ()
                      }
                      frame #1 {
                        n1170 = TDMS Close(11:w1977) -> (0:w1978:errorcluster)  [unwired: 1 in, 1 out]
                        n1171 = local write "data file error"(w1978) -> ()
                      }
                    }
                  }
                }
              }
            }
          }
          frame #8 {
            # "drive jigs"
            n1172 = stacked-sequence {
              frame #0 {
                # "jig on"
                n1173 = local read "jig cycle"() -> (w1979:dbl)
                n1174 = Equal?(x=w1979, y=0) -> (x = y?=w1981:bool)
                n1175 = case shown="True" w1981 {
                  frame False {
                  }
                  frame True {
                    n1176 = local read "LAB01-1RUN"() -> (w1982:bool)
                    n1177 = local read "LAB01-2 RUN"() -> (w1983:bool)
                    n1178 = local read "LAB03-1 RUN"() -> (w1989:bool)
                    n1179 = local read "LAB03-2 RUN"() -> (w1988:bool)
                    n1180 = local read "LAB02-1 RUN"() -> (w1991:bool)
                    n1181 = local read "LAB02-2 RUN"() -> (w1990:bool)
                    n1182 = local read "LAB04-1 RUN"() -> (w1987:bool)
                    n1183 = local read "LAB04-2 RUN"() -> (w1986:bool)
                    n1184 = local read "LAB05-1 RUN"() -> (w1985:bool)
                    n1185 = local read "LAB05-2 RUN"() -> (w1984:bool)
                    n1186 = local write "LAB05-1 (JIG)"(w1985) -> ()
                    n1187 = local write "LAB05-2 (JIG)"(w1984) -> ()
                    n1188 = local write "LAB04-2 (JIG)"(w1986) -> ()
                    n1189 = local write "LAB02-1 (JIG)"(w1991) -> ()
                    n1190 = local write "LAB03-1 (JIG)"(w1989) -> ()
                    n1191 = local write "LAB04-1 (JIG)"(w1987) -> ()
                    n1192 = local write "LAB03-2 (JIG)"(w1988) -> ()
                    n1193 = local write "LAB02-2 (JIG)"(w1990) -> ()
                    n1194 = local write "LAB01-1 (JIG)"(w1982) -> ()
                    n1195 = local write "LAB01-2 (JIG)"(w1983) -> ()
                  }
                }
              }
              frame #1 {
                # "jig off"
                n1196 = local read "jig cycle"() -> (w1994:dbl)
                n1197 = local read "on loops"() -> (w1993:dbl)
                n1198 = Equal?(x=w1994, y=w1993) -> (x = y?=w1992:bool)
                n1199 = case shown="True" w1992 {
                  frame False {
                  }
                  frame True {
                    w2045 = FALSE
                    w2046 = TRUE
                    w2044 = 2
                    n1200 = local read "LAB05-2 SELECT"() -> (w2035:T3)
                    n1201 = local read "LAB04-2 SELECT"() -> (w2037:T3)
                    n1202 = local read "LAB04-1 SELECT"() -> (w2038:T3)
                    n1203 = local read "LAB05-1 SELECT"() -> (w2036:T3)
                    n1204 = local read "LAB03-2 SELECT"() -> (w2039:T3)
                    n1205 = local read "LAB02-1 SELECT"() -> (w2042:T3)
                    n1206 = local read "LAB03-1 SELECT"() -> (w2040:T3)
                    n1207 = local read "LAB02-2 SELECT"() -> (w2041:T3)
                    n1208 = local read "LAB01-2 SELECT"() -> (w2043:T3)
                    n1209 = local read "LAB05-1 RUN"() -> (w2005:bool)
                    n1210 = local read "LAB05-2 RUN"() -> (w2004:bool)
                    n1211 = local read "LAB04-2 RUN"() -> (w2006:bool)
                    n1212 = local read "LAB04-1 RUN"() -> (w2007:bool)
                    n1213 = local read "LAB01-2 RUN"() -> (w2012:bool)
                    n1214 = local read "LAB03-2 RUN"() -> (w2008:bool)
                    n1215 = local read "LAB01-1RUN"() -> (w2023:bool)
                    n1216 = local read "LAB01-1 SELECT"() -> (w2047:T3)
                    n1217 = local read "LAB03-1 RUN"() -> (w2009:bool)
                    n1218 = local read "LAB02-1 RUN"() -> (w2011:bool)
                    n1219 = local read "LAB02-2 RUN"() -> (w2010:bool)
                    n1220 = Equal?(x=w2044, y=w2040) -> (x = y?=w2018:bool)
                    n1221 = Equal?(x=w2044, y=w2039) -> (x = y?=w2017:bool)
                    n1222 = Equal?(x=w2044, y=w2038) -> (x = y?=w2016:bool)
                    n1223 = Equal?(x=w2044, y=w2037) -> (x = y?=w2015:bool)
                    n1224 = Equal?(x=w2044, y=w2036) -> (x = y?=w2014:bool)
                    n1225 = Equal?(x=w2044, y=w2035) -> (x = y?=w2013:bool)
                    n1226 = Equal?(x=w2044, y=w2047) -> (x = y?=w2024:bool)
                    n1227 = Equal?(x=w2044, y=w2042) -> (x = y?=w2020:bool)
                    n1228 = Equal?(x=w2044, y=w2041) -> (x = y?=w2019:bool)
                    n1229 = Equal?(x=w2044, y=w2043) -> (x = y?=w2021:bool)
                    n1230 = And(x=w2015, y=w2006) -> (x .and. y?=w1997:bool)
                    n1231 = And(x=w2018, y=w2009) -> (x .and. y?=w2000:bool)
                    n1232 = And(x=w2016, y=w2007) -> (x .and. y?=w1998:bool)
                    n1233 = And(x=w2013, y=w2004) -> (x .and. y?=w1995:bool)
                    n1234 = And(x=w2019, y=w2010) -> (x .and. y?=w2001:bool)
                    n1235 = And(x=w2017, y=w2008) -> (x .and. y?=w1999:bool)
                    n1236 = And(x=w2014, y=w2005) -> (x .and. y?=w1996:bool)
                    n1237 = And(x=w2021, y=w2012) -> (x .and. y?=w2003:bool)
                    n1238 = And(x=w2024, y=w2023) -> (x .and. y?=w2022:bool)
                    n1239 = And(x=w2020, y=w2011) -> (x .and. y?=w2002:bool)
                    n1240 = Select(t=w2046, s=w2022, f=w2045) -> (s? t:f=w2025:bool)
                    n1241 = Select(t=w2046, s=w2003, f=w2045) -> (s? t:f=w2026:bool)
                    n1242 = Select(t=w2046, s=w2002, f=w2045) -> (s? t:f=w2027:bool)
                    n1243 = Select(t=w2046, s=w2001, f=w2045) -> (s? t:f=w2028:bool)
                    n1244 = Select(t=w2046, s=w2000, f=w2045) -> (s? t:f=w2029:bool)
                    n1245 = Select(t=w2046, s=w1999, f=w2045) -> (s? t:f=w2030:bool)
                    n1246 = Select(t=w2046, s=w1998, f=w2045) -> (s? t:f=w2031:bool)
                    n1247 = Select(t=w2046, s=w1997, f=w2045) -> (s? t:f=w2032:bool)
                    n1248 = Select(t=w2046, s=w1996, f=w2045) -> (s? t:f=w2033:bool)
                    n1249 = Select(t=w2046, s=w1995, f=w2045) -> (s? t:f=w2034:bool)
                    n1250 = local write "LAB03-2 (JIG)"(w2030) -> ()
                    n1251 = local write "LAB02-1 (JIG)"(w2027) -> ()
                    n1252 = local write "LAB02-2 (JIG)"(w2028) -> ()
                    n1253 = local write "LAB01-2 (JIG)"(w2026) -> ()
                    n1254 = local write "LAB03-1 (JIG)"(w2029) -> ()
                    n1255 = local write "LAB01-1 (JIG)"(w2025) -> ()
                    n1256 = local write "LAB05-2 (JIG)"(w2034) -> ()
                    n1257 = local write "LAB04-1 (JIG)"(w2031) -> ()
                    n1258 = local write "LAB05-1 (JIG)"(w2033) -> ()
                    n1259 = local write "LAB04-2 (JIG)"(w2032) -> ()
                  }
                }
              }
            }
          }
          frame #9 {
            # "drive digital output"
            n1260 = local read "LAB05-2 (O/I)"() -> (w2053:bool)
            n1261 = local read "LAB05-2 (JIG)"() -> (w2052:bool)
            n1262 = local read "LAB05-1 (O/I)"() -> (w2055:bool)
            n1263 = local read "LAB05-1 (JIG)"() -> (w2054:bool)
            n1264 = local read "LAB04-2 (O/I)"() -> (w2057:bool)
            n1265 = local read "LAB04-2 (JIG)"() -> (w2056:bool)
            n1266 = local read "LAB03-1 (O/I)"() -> (w2062:bool)
            n1267 = local read "LAB04-1 (O/I)"() -> (w2058:bool)
            n1268 = local read "LAB04-1 (JIG)"() -> (w2051:bool)
            n1269 = local read "LAB02-1 (O/I)"() -> (w2066:bool)
            n1270 = local read "LAB02-2 (O/I)"() -> (w2064:bool)
            n1271 = local read "LAB03-2 (O/I)"() -> (w2060:bool)
            n1272 = local read "LAB03-2 (JIG)"() -> (w2059:bool)
            n1273 = local read "LAB02-1 (JIG)"() -> (w2065:bool)
            n1274 = local read "LAB02-2 (JIG)"() -> (w2063:bool)
            n1275 = local read "LAB03-1 (JIG)"() -> (w2061:bool)
            n1276 = local read "LAB01-2 (O/I)"() -> (w2068:bool)
            n1277 = local read "LAB01-2 (JIG)"() -> (w2067:bool)
            n1278 = local read "LAB01-1 (O/I)"() -> (w2070:bool)
            n1279 = local read "LAB01-1 (JIG)"() -> (w2069:bool)
            n1280 = Build Array(w2057, w2056, w2055, w2054, w2053, w2052) -> (w2048:bool[])
            n1281 = Build Array(w2063, w2062, w2061, w2060, w2059, w2058, w2051) -> (w2049:bool[])
            n1282 = Build Array(w2070, w2069, w2068, w2067, w2066, w2065, w2064) -> (w2050:bool[])
            n1283 = call "sub vi - Drive Relays All v6.vi"("Array #2"=w2048, "Array #1"=w2049, "Array #0"=w2050) -> ()  [unwired: 8 in, 1 out]
          }
          frame #10 {
            # "get temperature values"
            n1284 = stacked-sequence {
              frame #0 {
                n1285 = local read "jig cycle"() -> (w2071:dbl)
                n1286 = local read "on loops"() -> (w2074:dbl)
                n1287 = local read "jig cycle"() -> (w2076:dbl)
                n1288 = Add(x=w2074, y=2) -> (x+y=w2075:dbl)
                n1289 = Equal?(x=w2076, y=0) -> (x = y?=w2077:bool)
                n1290 = Equal?(x=w2071, y=w2075) -> (x = y?=w2072:bool)
                n1291 = case shown="True" w2077 {
                  frame False {
                  }
                  frame True {
                    w2089 = FALSE
                    w2090 = TRUE
                    n1292 = local write "TEMP update"(TRUE) -> ()
                    n1293 = call "sub vi - GET ALL TEMP v3.vi"("LA01-EN"=w2090, "LA02-EN"=w2090, "LA03-EN"=w2090, "LA04-EN"=w2089, "LA05-EN"=w2089, "Gen Cal Value"=1.0) -> ("LA01 TEMP"=w2088:T14, "LA02 TEMP"=w2086:T14, "LA03 TEMP"=w2085:T14)  [unwired: 4 in, 3 out]
                    n1294 = local write "LAB03 TEMP"(w2085) -> ()
                    n1295 = local write "LAB02 TEMP"(w2086) -> ()
                    n1296 = local write "LAB01 TEMP"(w2088) -> ()
                  }
                }
                n1297 = case shown="True" w2072 {
                  frame False {
                  }
                  frame True {
                    w2082 = TRUE
                    w2083 = FALSE
                    n1298 = local write "TEMP update"(TRUE) -> ()
                    n1299 = call "sub vi - GET ALL TEMP v3.vi"("LA01-EN"=w2083, "LA02-EN"=w2083, "LA03-EN"=w2083, "LA04-EN"=w2082, "LA05-EN"=w2082, "Gen Cal Value"=1.0) -> ("LA04 TEMP"=w2080:T14, "LA05 TEMP"=w2079:T14)  [unwired: 4 in, 4 out]
                    n1300 = local write "LAB04 TEMP"(w2080) -> ()
                    n1301 = local write "LAB05 TEMP"(w2079) -> ()
                  }
                }
              }
              frame #1 {
                n1302 = local read "LAB01 (CAL)"() -> (w2108:T6)
                n1303 = local read "LAB01 TEMP"() -> (w2109:T9)
                n1304 = Unbundle By Name(w2109) -> ("T1 Live"=w2099:dbl, "T1 Neut"=w2098:dbl, "T2 Live"=w2097:dbl, "T2 Neut"=w2096:dbl)  [unwired: 2 out]
                n1305 = Unbundle By Name(w2108) -> ("1 (TL) cal"=w2095:dbl, "1 (TN) cal"=w2094:dbl, "2 (TL) cal"=w2093:dbl, "2 (TN) cal"=w2092:dbl)  [unwired: 6 out]
                n1306 = Multiply(x=w2099, y=w2095) -> (x*y=w2105:dbl)
                n1307 = Multiply(x=w2098, y=w2094) -> (x*y=w2104:dbl)
                n1308 = Multiply(x=w2097, y=w2093) -> (x*y=w2101:dbl)
                n1309 = Multiply(x=w2096, y=w2092) -> (x*y=w2100:dbl)
                n1310 = local read "LAB01-2 (SIG)"() -> (w2103:T2)
                n1311 = local read "LAB01-1 (SIG)"() -> (w2107:T2)
                n1312 = Bundle By Name(cluster=w2107, "Tmp Live"=w2105, "Tmp Neut"=w2104) -> (w2106:T2)
                n1313 = Bundle By Name(cluster=w2103, "Tmp Live"=w2101, "Tmp Neut"=w2100) -> (w2102:T2)
                n1314 = local write "LAB01-1 (SIG)"(w2106) -> ()
                n1315 = local write "LAB01-2 (SIG)"(w2102) -> ()
              }
              frame #2 {
                n1316 = local read "LAB02 (CAL)"() -> (w2126:T7)
                n1317 = local read "LAB02 TEMP"() -> (w2127:T9)
                n1318 = Unbundle By Name(w2127) -> ("T1 Live"=w2117:dbl, "T1 Neut"=w2116:dbl, "T2 Live"=w2115:dbl, "T2 Neut"=w2114:dbl)  [unwired: 2 out]
                n1319 = Unbundle By Name(w2126) -> ("1 (TL) cal"=w2113:dbl, "1 (TN) cal"=w2112:dbl, "2 (TL) cal"=w2111:dbl, "2 (TN) cal"=w2110:dbl)  [unwired: 6 out]
                n1320 = Multiply(x=w2117, y=w2113) -> (x*y=w2123:dbl)
                n1321 = Multiply(x=w2116, y=w2112) -> (x*y=w2122:dbl)
                n1322 = Multiply(x=w2115, y=w2111) -> (x*y=w2119:dbl)
                n1323 = Multiply(x=w2114, y=w2110) -> (x*y=w2118:dbl)
                n1324 = local read "LAB02-2 (SIG)"() -> (w2121:T2)
                n1325 = local read "LAB02-1 (SIG)"() -> (w2125:T2)
                n1326 = Bundle By Name(cluster=w2125, "Tmp Live"=w2123, "Tmp Neut"=w2122) -> (w2124:T2)
                n1327 = Bundle By Name(cluster=w2121, "Tmp Live"=w2119, "Tmp Neut"=w2118) -> (w2120:T2)
                n1328 = local write "LAB02-1 (SIG)"(w2124) -> ()
                n1329 = local write "LAB02-2 (SIG)"(w2120) -> ()
              }
              frame #3 {
                n1330 = local read "LAB03 (CAL)"() -> (w2144:T6)
                n1331 = local read "LAB03 TEMP"() -> (w2145:T9)
                n1332 = Unbundle By Name(w2145) -> ("T1 Live"=w2135:dbl, "T1 Neut"=w2134:dbl, "T2 Live"=w2133:dbl, "T2 Neut"=w2132:dbl)  [unwired: 2 out]
                n1333 = Unbundle By Name(w2144) -> ("1 (TL) cal"=w2131:dbl, "1 (TN) cal"=w2130:dbl, "2 (TL) cal"=w2129:dbl, "2 (TN) cal"=w2128:dbl)  [unwired: 6 out]
                n1334 = Multiply(x=w2135, y=w2131) -> (x*y=w2141:dbl)
                n1335 = Multiply(x=w2134, y=w2130) -> (x*y=w2140:dbl)
                n1336 = Multiply(x=w2133, y=w2129) -> (x*y=w2137:dbl)
                n1337 = Multiply(x=w2132, y=w2128) -> (x*y=w2136:dbl)
                n1338 = local read "LAB03-2 (SIG)"() -> (w2139:T2)
                n1339 = local read "LAB03-1 (SIG)"() -> (w2143:T2)
                n1340 = Bundle By Name(cluster=w2143, "Tmp Live"=w2141, "Tmp Neut"=w2140) -> (w2142:T2)
                n1341 = Bundle By Name(cluster=w2139, "Tmp Live"=w2137, "Tmp Neut"=w2136) -> (w2138:T2)
                n1342 = local write "LAB03-1 (SIG)"(w2142) -> ()
                n1343 = local write "LAB03-2 (SIG)"(w2138) -> ()
              }
              frame #4 {
                n1344 = local read "LAB04 (CAL)"() -> (w2162:T6)
                n1345 = local read "LAB04 TEMP"() -> (w2163:T9)
                n1346 = Unbundle By Name(w2163) -> ("T1 Live"=w2153:dbl, "T1 Neut"=w2152:dbl, "T2 Live"=w2151:dbl, "T2 Neut"=w2150:dbl)  [unwired: 2 out]
                n1347 = Unbundle By Name(w2162) -> ("1 (TL) cal"=w2149:dbl, "1 (TN) cal"=w2148:dbl, "2 (TL) cal"=w2147:dbl, "2 (TN) cal"=w2146:dbl)  [unwired: 6 out]
                n1348 = Multiply(x=w2153, y=w2149) -> (x*y=w2159:dbl)
                n1349 = Multiply(x=w2152, y=w2148) -> (x*y=w2158:dbl)
                n1350 = Multiply(x=w2151, y=w2147) -> (x*y=w2155:dbl)
                n1351 = Multiply(x=w2150, y=w2146) -> (x*y=w2154:dbl)
                n1352 = local read "LAB04-2 (SIG)"() -> (w2157:T2)
                n1353 = local read "LAB04-1 (SIG)"() -> (w2161:T2)
                n1354 = Bundle By Name(cluster=w2161, "Tmp Live"=w2159, "Tmp Neut"=w2158) -> (w2160:T2)
                n1355 = Bundle By Name(cluster=w2157, "Tmp Live"=w2155, "Tmp Neut"=w2154) -> (w2156:T2)
                n1356 = local write "LAB04-1 (SIG)"(w2160) -> ()
                n1357 = local write "LAB04-2 (SIG)"(w2156) -> ()
              }
              frame #5 {
                n1358 = local read "LAB05 (CAL)"() -> (w2180:T6)
                n1359 = local read "LAB05 TEMP"() -> (w2181:T9)
                n1360 = Unbundle By Name(w2181) -> ("T1 Live"=w2171:dbl, "T1 Neut"=w2170:dbl, "T2 Live"=w2169:dbl, "T2 Neut"=w2168:dbl)  [unwired: 2 out]
                n1361 = Unbundle By Name(w2180) -> ("1 (TL) cal"=w2167:dbl, "1 (TN) cal"=w2166:dbl, "2 (TL) cal"=w2165:dbl, "2 (TN) cal"=w2164:dbl)  [unwired: 6 out]
                n1362 = Multiply(x=w2171, y=w2167) -> (x*y=w2177:dbl)
                n1363 = Multiply(x=w2170, y=w2166) -> (x*y=w2176:dbl)
                n1364 = Multiply(x=w2169, y=w2165) -> (x*y=w2173:dbl)
                n1365 = Multiply(x=w2168, y=w2164) -> (x*y=w2172:dbl)
                n1366 = local read "LAB05-2 (SIG)"() -> (w2175:T2)
                n1367 = local read "LAB05-1 (SIG)"() -> (w2179:T2)
                n1368 = Bundle By Name(cluster=w2179, "Tmp Live"=w2177, "Tmp Neut"=w2176) -> (w2178:T2)
                n1369 = Bundle By Name(cluster=w2175, "Tmp Live"=w2173, "Tmp Neut"=w2172) -> (w2174:T2)
                n1370 = local write "LAB05-1 (SIG)"(w2178) -> ()
                n1371 = local write "LAB05-2 (SIG)"(w2174) -> ()
              }
            }
          }
          frame #11 {
            # "get analog values"
            n1372 = local read "on loops"() -> (w2188:dbl)
            n1373 = local read "jig cycle"() -> (w2185:dbl)
            n1374 = Add(x=w2188, y=1) -> (x+y=w2186:dbl)
            n1375 = Equal?(x=w2185, y=1) -> (x = y?=w2183:bool)
            n1376 = Equal?(x=w2185, y=w2186) -> (x = y?=w2184:bool)
            n1377 = Or(x=w2183, y=w2184) -> (x .or. y?=w2182:bool)
            n1378 = case shown="True" w2182 {
              frame False {
              }
              frame True {
                n1379 = call "sub vi - Read Analog All v8.vi"() -> ("Analog loop time"=w2196:dbl, "array GRAPH"=w2195:dynamicdata[], "LAB01"=w2194:T15, "LAB02"=w2193:T16, "LAB03"=w2192:T17, "LAB04"=w2191:T18, "array ERROR"=w2197:errorcluster[], "LAB05"=w2190:T19)  [unwired: 8 in]
                n1380 = stacked-sequence {
                  tunnel: w2197 -> [w2200 _ _ _ _ _]
                  tunnel: w2196 -> [w2199 _ _ _ _ _]
                  tunnel: w2195 -> [w2198 _ _ _ _ _]
                  tunnel: w2194 -> [_ w2245 _ _ _ _]
                  tunnel: w2193 -> [_ _ w2246 _ _ _]
                  tunnel: w2192 -> [_ _ _ w2270 _ _]
                  tunnel: w2191 -> [_ _ _ _ w2294 _]
                  tunnel: w2190 -> [_ _ _ _ _ w2318]
                  frame #0 {
                    n1381 = local write "AI update"(TRUE) -> ()
                    n1382 = Index Array(array=w2198, index=6) -> (element=→"LAB04-1 (GRAPH)":dynamicdata)
                    n1383 = Index Array(array=w2198, index=7) -> (element=→"LAB04-2 (GRAPH)":dynamicdata)
                    n1384 = Index Array(array=w2198, index=9) -> (element=→"LAB05-2 (GRAPH)":dynamicdata)
                    n1385 = Index Array(array=w2198, index=8) -> (element=→"LAB05-1 (GRAPH)":dynamicdata)
                    n1386 = Index Array(array=w2198, index=5) -> (element=→"LAB03-2 (GRAPH)":dynamicdata)
                    n1387 = Index Array(array=w2198, index=0) -> (element=→"LAB01-1 (GRAPH)":dynamicdata)
                    n1388 = Index Array(array=w2198, index=1) -> (element=→"LAB01-2 (GRAPH)":dynamicdata)
                    n1389 = Index Array(array=w2198, index=2) -> (element=→"LAB02-1 (GRAPH)":dynamicdata)
                    n1390 = Index Array(array=w2198, index=3) -> (element=→"LAB02-2 (GRAPH)":dynamicdata)
                    n1391 = Index Array(array=w2198, index=4) -> (element=→"LAB03-1 (GRAPH)":dynamicdata)
                    "AI loop time" <- w2199
                    "Analog Error Array" <- w2200
                  }
                  frame #1 {
                    n1392 = local read "LAB01 (CAL)"() -> (w2244:T6)
                    n1393 = Unbundle By Name(w2245) -> ("LAB01-1 (A)"=w2243:dbl, "LAB01-1 (V)"=w2242:dbl, "LAB01-1 (PF)"=w2241:dbl, "LAB01-2 (A)"=w2240:dbl, "LAB01-2 (V)"=w2239:dbl, "LAB01-2 (PF)"=w2238:dbl)
                    n1394 = Unbundle By Name(w2244) -> ("1  (A) cal"=w2237:dbl, "1 (V) cal"=w2236:dbl, "1 (PF) cal"=w2235:dbl, "2 (A) cal"=w2234:dbl, "2 (V) cal"=w2233:dbl, "2 (PF) cal"=w2232:dbl)  [unwired: 4 out]
                    n1395 = Multiply(x=w2243, y=w2237) -> (x*y=w2230:dbl)
                    n1396 = Multiply(x=w2242, y=w2236) -> (x*y=w2229:dbl)
                    n1397 = Multiply(x=w2241, y=w2235) -> (x*y=w2228:dbl)
                    n1398 = Multiply(x=w2240, y=w2234) -> (x*y=w2224:dbl)
                    n1399 = local read "LAB01-1 (SIG)"() -> (w2231:T2)
                    n1400 = Multiply(x=w2239, y=w2233) -> (x*y=w2223:dbl)
                    n1401 = Multiply(x=w2238, y=w2232) -> (x*y=w2222:dbl)
                    n1402 = local read "LAB01-2 (SIG)"() -> (w2226:T2)
                    n1403 = Bundle By Name(cluster=w2231, "AMPS"=w2230, "VOLTS"=w2229, "PF"=w2228) -> (w2227:T2)
                    n1404 = Bundle By Name(cluster=w2226, "AMPS"=w2224, "VOLTS"=w2223, "PF"=w2222) -> (w2225:T2)
                    n1405 = local write "LAB01-2 (SIG)"(w2225) -> ()
                    n1406 = local write "LAB01-1 (SIG)"(w2227) -> ()
                  }
                  frame #2 {
                    n1407 = local read "LAB02 (CAL)"() -> (w2269:T7)
                    n1408 = Unbundle By Name(w2246) -> ("LAB02-1 (A)"=w2268:dbl, "LAB02-1 (V)"=w2267:dbl, "LAB02-1 (PF)"=w2266:dbl, "LAB02-2 (A)"=w2265:dbl, "LAB02-2 (V)"=w2264:dbl, "LAB02-2 (PF)"=w2263:dbl)
                    n1409 = Unbundle By Name(w2269) -> ("1 (A) cal"=w2262:dbl, "1 (V) cal"=w2261:dbl, "1 (PF) cal"=w2260:dbl, "2 (A) cal"=w2259:dbl, "2 (V) cal"=w2258:dbl, "2 (PF) cal"=w2257:dbl)  [unwired: 4 out]
                    n1410 = Multiply(x=w2268, y=w2262) -> (x*y=w2255:dbl)
                    n1411 = Multiply(x=w2267, y=w2261) -> (x*y=w2254:dbl)
                    n1412 = Multiply(x=w2266, y=w2260) -> (x*y=w2253:dbl)
                    n1413 = Multiply(x=w2265, y=w2259) -> (x*y=w2249:dbl)
                    n1414 = local read "LAB02-1 (SIG)"() -> (w2256:T2)
                    n1415 = Multiply(x=w2264, y=w2258) -> (x*y=w2248:dbl)
                    n1416 = Multiply(x=w2263, y=w2257) -> (x*y=w2247:dbl)
                    n1417 = local read "LAB02-2 (SIG)"() -> (w2251:T2)
                    n1418 = Bundle By Name(cluster=w2256, "AMPS"=w2255, "VOLTS"=w2254, "PF"=w2253) -> (w2252:T2)
                    n1419 = Bundle By Name(cluster=w2251, "AMPS"=w2249, "VOLTS"=w2248, "PF"=w2247) -> (w2250:T2)
                    n1420 = local write "LAB02-2 (SIG)"(w2250) -> ()
                    n1421 = local write "LAB02-1 (SIG)"(w2252) -> ()
                  }
                  frame #3 {
                    n1422 = local read "LAB03 (CAL)"() -> (w2293:T6)
                    n1423 = Unbundle By Name(w2270) -> ("LAB03-1 (A)"=w2292:dbl, "LAB03-1 (V)"=w2291:dbl, "LAB03-1 (PF)"=w2290:dbl, "LAB03-2 (A)"=w2289:dbl, "LAB03-2 (V)"=w2288:dbl, "LAB03-2 (PF)"=w2287:dbl)
                    n1424 = Unbundle By Name(w2293) -> ("1  (A) cal"=w2286:dbl, "1 (V) cal"=w2285:dbl, "1 (PF) cal"=w2284:dbl, "2 (A) cal"=w2283:dbl, "2 (V) cal"=w2282:dbl, "2 (PF) cal"=w2281:dbl)  [unwired: 4 out]
                    n1425 = Multiply(x=w2292, y=w2286) -> (x*y=w2279:dbl)
                    n1426 = Multiply(x=w2291, y=w2285) -> (x*y=w2278:dbl)
                    n1427 = Multiply(x=w2290, y=w2284) -> (x*y=w2277:dbl)
                    n1428 = Multiply(x=w2289, y=w2283) -> (x*y=w2273:dbl)
                    n1429 = local read "LAB03-1 (SIG)"() -> (w2280:T2)
                    n1430 = Multiply(x=w2288, y=w2282) -> (x*y=w2272:dbl)
                    n1431 = Multiply(x=w2287, y=w2281) -> (x*y=w2271:dbl)
                    n1432 = local read "LAB03-1 (SIG)"() -> (w2275:T2)
                    n1433 = Bundle By Name(cluster=w2280, "AMPS"=w2279, "VOLTS"=w2278, "PF"=w2277) -> (w2276:T2)
                    n1434 = Bundle By Name(cluster=w2275, "AMPS"=w2273, "VOLTS"=w2272, "PF"=w2271) -> (w2274:T2)
                    n1435 = local write "LAB03-1 (SIG)"(w2274) -> ()
                    n1436 = local write "LAB03-1 (SIG)"(w2276) -> ()
                  }
                  frame #4 {
                    n1437 = local read "LAB04 (CAL)"() -> (w2317:T6)
                    n1438 = Unbundle By Name(w2294) -> ("LAB04-1 (A)"=w2316:dbl, "LAB04-1 (V)"=w2315:dbl, "LAB04-1 (PF)"=w2314:dbl, "LAB04-2 (A)"=w2313:dbl, "LAB04-2 (V)"=w2312:dbl, "LAB04-2 (PF)"=w2311:dbl)
                    n1439 = Unbundle By Name(w2317) -> ("1  (A) cal"=w2310:dbl, "1 (V) cal"=w2309:dbl, "1 (PF) cal"=w2308:dbl, "2 (A) cal"=w2307:dbl, "2 (V) cal"=w2306:dbl, "2 (PF) cal"=w2305:dbl)  [unwired: 4 out]
                    n1440 = Multiply(x=w2316, y=w2310) -> (x*y=w2303:dbl)
                    n1441 = Multiply(x=w2315, y=w2309) -> (x*y=w2302:dbl)
                    n1442 = Multiply(x=w2314, y=w2308) -> (x*y=w2301:dbl)
                    n1443 = Multiply(x=w2313, y=w2307) -> (x*y=w2297:dbl)
                    n1444 = local read "LAB04-1 (SIG)"() -> (w2304:T2)
                    n1445 = Multiply(x=w2312, y=w2306) -> (x*y=w2296:dbl)
                    n1446 = Multiply(x=w2311, y=w2305) -> (x*y=w2295:dbl)
                    n1447 = local read "LAB04-2 (SIG)"() -> (w2299:T2)
                    n1448 = Bundle By Name(cluster=w2304, "AMPS"=w2303, "VOLTS"=w2302, "PF"=w2301) -> (w2300:T2)
                    n1449 = Bundle By Name(cluster=w2299, "AMPS"=w2297, "VOLTS"=w2296, "PF"=w2295) -> (w2298:T2)
                    n1450 = local write "LAB04-2 (SIG)"(w2298) -> ()
                    n1451 = local write "LAB04-1 (SIG)"(w2300) -> ()
                  }
                  frame #5 {
                    n1452 = local read "LAB05 (CAL)"() -> (w2341:T6)
                    n1453 = Unbundle By Name(w2318) -> ("LAB05-1 (A)"=w2340:dbl, "LAB05-1 (V)"=w2339:dbl, "LAB05-1 (PF)"=w2338:dbl, "LAB05-2 (A)"=w2337:dbl, "LAB05-2 (V)"=w2336:dbl, "LAB05-2 (PF)"=w2335:dbl)
                    n1454 = Unbundle By Name(w2341) -> ("1  (A) cal"=w2334:dbl, "1 (V) cal"=w2333:dbl, "1 (PF) cal"=w2332:dbl, "2 (A) cal"=w2331:dbl, "2 (V) cal"=w2330:dbl, "2 (PF) cal"=w2329:dbl)  [unwired: 4 out]
                    n1455 = Multiply(x=w2340, y=w2334) -> (x*y=w2327:dbl)
                    n1456 = Multiply(x=w2339, y=w2333) -> (x*y=w2326:dbl)
                    n1457 = Multiply(x=w2338, y=w2332) -> (x*y=w2325:dbl)
                    n1458 = Multiply(x=w2337, y=w2331) -> (x*y=w2321:dbl)
                    n1459 = local read "LAB05-1 (SIG)"() -> (w2328:T2)
                    n1460 = Multiply(x=w2336, y=w2330) -> (x*y=w2320:dbl)
                    n1461 = Multiply(x=w2335, y=w2329) -> (x*y=w2319:dbl)
                    n1462 = local read "LAB05-2 (SIG)"() -> (w2323:T2)
                    n1463 = Bundle By Name(cluster=w2328, "AMPS"=w2327, "VOLTS"=w2326, "PF"=w2325) -> (w2324:T2)
                    n1464 = Bundle By Name(cluster=w2323, "AMPS"=w2321, "VOLTS"=w2320, "PF"=w2319) -> (w2322:T2)
                    n1465 = local write "LAB05-2 (SIG)"(w2322) -> ()
                    n1466 = local write "LAB05-1 (SIG)"(w2324) -> ()
                  }
                }
              }
            }
          }
          frame #12 {
            # "save test data to file"
            n1467 = local read "on loops"() -> (w2358:dbl)
            n1468 = local read "jig cycle"() -> (w2355:dbl)
            n1469 = Add(x=w2358, y=2) -> (x+y=w2356:dbl)
            n1470 = Equal?(x=w2355, y=1) -> (x = y?=w2353:bool)
            n1471 = Equal?(x=w2355, y=w2356) -> (x = y?=w2354:bool)
            n1472 = Or(x=w2353, y=w2354) -> (x .or. y?=w2352:bool)
            n1473 = case shown="True" w2352 {
              tunnel: w2351 -> [_ w2369]
              tunnel: w2350 -> [_ w2368]
              tunnel: w2349 -> [_ w2367]
              tunnel: w2348 -> [_ w2366]
              tunnel: w2347 -> [_ w2365]
              tunnel: w2346 -> [_ w2364]
              tunnel: w2345 -> [_ w2363]
              tunnel: w2344 -> [_ w2362]
              tunnel: w2343 -> [_ w2361]
              tunnel: w2342 -> [_ w2360]
              frame False {
              }
              frame True {
                n1474 = stacked-sequence {
                  tunnel: w2369 -> [w2370 _ _ _ _ _ _ _ _ _]
                  tunnel: w2368 -> [_ w2415 _ _ _ _ _ _ _ _]
                  tunnel: w2367 -> [_ _ w2460 _ _ _ _ _ _ _]
                  tunnel: w2366 -> [_ _ _ w2505 _ _ _ _ _ _]
                  tunnel: w2365 -> [_ _ _ _ w2550 _ _ _ _ _]
                  tunnel: w2364 -> [_ _ _ _ _ w2595 _ _ _ _]
                  tunnel: w2363 -> [_ _ _ _ _ _ w2640 _ _ _]
                  tunnel: w2362 -> [_ _ _ _ _ _ _ w2685 _ _]
                  tunnel: w2361 -> [_ _ _ _ _ _ _ _ w2730 _]
                  tunnel: w2360 -> [_ _ _ _ _ _ _ _ _ w2775]
                  frame #0 {
                    # "LAB01-1"
                    n1475 = case shown="True" w2370 {
                      frame False {
                      }
                      frame True {
                        n1476 = local read "LAB01-1 (DISP)"() -> (w2412:T4)
                        n1477 = local read "LAB01-1 (SIG)"() -> (w2413:T2)
                        n1478 = local read "LAB01-1 (TDMS)"() -> (w2414:refnum<k34>)
                        n1479 = Build Array("TEMP Neut") -> (w2378:string[])
                        n1480 = Build Array("CYCLE") -> (w2373:string[])
                        n1481 = Build Array("TEMP Live") -> (w2383:string[])
                        n1482 = Build Array("PF") -> (w2388:string[])
                        n1483 = Build Array("AMPS") -> (w2409:string[])
                        n1484 = Build Array("VOLTS") -> (w2400:string[])
                        n1485 = Unbundle(w2413) -> ("AMPS"=w2408:dbl, "VOLTS"=w2397:dbl, "PF"=w2396:dbl, "Tmp Live"=w2395:dbl, "Tmp Neut"=w2398:dbl)
                        n1486 = Unbundle(w2412) -> ("CYCLE"=w2393:dbl)  [unwired: 2 out]
                        n1487 = Build Array(w2397) -> (w2394:dbl[])
                        n1488 = Build Array(w2396) -> (w2387:dbl[])
                        n1489 = Build Array(w2395) -> (w2382:dbl[])
                        n1490 = Build Array(w2398) -> (w2377:dbl[])
                        n1491 = Build Array(w2408) -> (w2407:dbl[])
                        n1492 = Build Array(w2393) -> (w2372:dbl[])
                        n1493 = TDMS Write(0:w2414, 5:"LAB01-1 TEST VALUES", 7:w2409, 9:w2407) -> (4:w2402:refnum<k34>, 6:w2401:string, 15:w2389:errorcluster)  [unwired: 2 in, 1 out]
                        n1494 = TDMS Write(0:w2402, 5:w2401, 7:w2400, 9:w2394, 11:w2389) -> (4:w2392:refnum<k34>, 6:w2391:string, 15:w2390:errorcluster)  [unwired: 1 in, 1 out]
                        n1495 = TDMS Write(0:w2392, 5:w2391, 7:w2388, 9:w2387, 11:w2390) -> (4:w2386:refnum<k34>, 6:w2385:string, 15:w2384:errorcluster)  [unwired: 1 in, 1 out]
                        n1496 = TDMS Write(0:w2386, 5:w2385, 7:w2383, 9:w2382, 11:w2384) -> (4:w2381:refnum<k34>, 6:w2380:string, 15:w2379:errorcluster)  [unwired: 1 in, 1 out]
                        n1497 = TDMS Write(0:w2381, 5:w2380, 7:w2378, 9:w2377, 11:w2379) -> (4:w2376:refnum<k34>, 6:w2375:string, 15:w2374:errorcluster)  [unwired: 1 in, 1 out]
                        n1498 = TDMS Write(0:w2376, 5:w2375, 7:w2373, 9:w2372, 11:w2374) -> (15:w2371:errorcluster)  [unwired: 1 in, 3 out]
                        n1499 = local write "data file error"(w2371) -> ()
                      }
                    }
                  }
                  frame #1 {
                    # "LAB01-2"
                    n1500 = case shown="True" w2415 {
                      frame False {
                      }
                      frame True {
                        n1501 = local read "LAB01-2 (DISP)"() -> (w2457:T4)
                        n1502 = local read "LAB01-2 (SIG)"() -> (w2458:T2)
                        n1503 = local read "LAB01-2 (TDMS)"() -> (w2459:refnum<k34>)
                        n1504 = Build Array("TEMP Neut") -> (w2423:string[])
                        n1505 = Build Array("CYCLE") -> (w2418:string[])
                        n1506 = Build Array("TEMP Live") -> (w2428:string[])
                        n1507 = Build Array("PF") -> (w2433:string[])
                        n1508 = Build Array("AMPS") -> (w2454:string[])
                        n1509 = Build Array("VOLTS") -> (w2445:string[])
                        n1510 = Unbundle(w2458) -> ("AMPS"=w2453:dbl, "VOLTS"=w2442:dbl, "PF"=w2441:dbl, "Tmp Live"=w2440:dbl, "Tmp Neut"=w2443:dbl)
                        n1511 = Unbundle(w2457) -> ("CYCLE"=w2438:dbl)  [unwired: 2 out]
                        n1512 = Build Array(w2442) -> (w2439:dbl[])
                        n1513 = Build Array(w2441) -> (w2432:dbl[])
                        n1514 = Build Array(w2440) -> (w2427:dbl[])
                        n1515 = Build Array(w2443) -> (w2422:dbl[])
                        n1516 = Build Array(w2453) -> (w2452:dbl[])
                        n1517 = Build Array(w2438) -> (w2417:dbl[])
                        n1518 = TDMS Write(0:w2459, 5:"LAB01-2 TEST VALUES", 7:w2454, 9:w2452) -> (4:w2447:refnum<k34>, 6:w2446:string, 15:w2434:errorcluster)  [unwired: 2 in, 1 out]
                        n1519 = TDMS Write(0:w2447, 5:w2446, 7:w2445, 9:w2439, 11:w2434) -> (4:w2437:refnum<k34>, 6:w2436:string, 15:w2435:errorcluster)  [unwired: 1 in, 1 out]
                        n1520 = TDMS Write(0:w2437, 5:w2436, 7:w2433, 9:w2432, 11:w2435) -> (4:w2431:refnum<k34>, 6:w2430:string, 15:w2429:errorcluster)  [unwired: 1 in, 1 out]
                        n1521 = TDMS Write(0:w2431, 5:w2430, 7:w2428, 9:w2427, 11:w2429) -> (4:w2426:refnum<k34>, 6:w2425:string, 15:w2424:errorcluster)  [unwired: 1 in, 1 out]
                        n1522 = TDMS Write(0:w2426, 5:w2425, 7:w2423, 9:w2422, 11:w2424) -> (4:w2421:refnum<k34>, 6:w2420:string, 15:w2419:errorcluster)  [unwired: 1 in, 1 out]
                        n1523 = TDMS Write(0:w2421, 5:w2420, 7:w2418, 9:w2417, 11:w2419) -> (15:w2416:errorcluster)  [unwired: 1 in, 3 out]
                        n1524 = local write "data file error"(w2416) -> ()
                      }
                    }
                  }
                  frame #2 {
                    # "LAB02-1"
                    n1525 = case shown="True" w2460 {
                      frame False {
                      }
                      frame True {
                        n1526 = local read "LAB02-1 (DISP)"() -> (w2502:T4)
                        n1527 = local read "LAB02-1 (SIG)"() -> (w2503:T2)
                        n1528 = local read "LAB02-1 (TDMS)"() -> (w2504:refnum<k34>)
                        n1529 = Build Array("TEMP Neut") -> (w2468:string[])
                        n1530 = Build Array("CYCLE") -> (w2463:string[])
                        n1531 = Build Array("TEMP Live") -> (w2473:string[])
                        n1532 = Build Array("PF") -> (w2478:string[])
                        n1533 = Build Array("AMPS") -> (w2499:string[])
                        n1534 = Build Array("VOLTS") -> (w2490:string[])
                        n1535 = Unbundle(w2503) -> ("AMPS"=w2498:dbl, "VOLTS"=w2487:dbl, "PF"=w2486:dbl, "Tmp Live"=w2485:dbl, "Tmp Neut"=w2488:dbl)
                        n1536 = Unbundle(w2502) -> ("CYCLE"=w2483:dbl)  [unwired: 2 out]
                        n1537 = Build Array(w2487) -> (w2484:dbl[])
                        n1538 = Build Array(w2486) -> (w2477:dbl[])
                        n1539 = Build Array(w2485) -> (w2472:dbl[])
                        n1540 = Build Array(w2488) -> (w2467:dbl[])
                        n1541 = Build Array(w2498) -> (w2497:dbl[])
                        n1542 = Build Array(w2483) -> (w2462:dbl[])
                        n1543 = TDMS Write(0:w2504, 5:"LAB02-1 TEST VALUES", 7:w2499, 9:w2497) -> (4:w2492:refnum<k34>, 6:w2491:string, 15:w2479:errorcluster)  [unwired: 2 in, 1 out]
                        n1544 = TDMS Write(0:w2492, 5:w2491, 7:w2490, 9:w2484, 11:w2479) -> (4:w2482:refnum<k34>, 6:w2481:string, 15:w2480:errorcluster)  [unwired: 1 in, 1 out]
                        n1545 = TDMS Write(0:w2482, 5:w2481, 7:w2478, 9:w2477, 11:w2480) -> (4:w2476:refnum<k34>, 6:w2475:string, 15:w2474:errorcluster)  [unwired: 1 in, 1 out]
                        n1546 = TDMS Write(0:w2476, 5:w2475, 7:w2473, 9:w2472, 11:w2474) -> (4:w2471:refnum<k34>, 6:w2470:string, 15:w2469:errorcluster)  [unwired: 1 in, 1 out]
                        n1547 = TDMS Write(0:w2471, 5:w2470, 7:w2468, 9:w2467, 11:w2469) -> (4:w2466:refnum<k34>, 6:w2465:string, 15:w2464:errorcluster)  [unwired: 1 in, 1 out]
                        n1548 = TDMS Write(0:w2466, 5:w2465, 7:w2463, 9:w2462, 11:w2464) -> (15:w2461:errorcluster)  [unwired: 1 in, 3 out]
                        n1549 = local write "data file error"(w2461) -> ()
                      }
                    }
                  }
                  frame #3 {
                    # "LAB02-2"
                    n1550 = case shown="True" w2505 {
                      frame False {
                      }
                      frame True {
                        n1551 = local read "LAB02-2 (DISP)"() -> (w2547:T4)
                        n1552 = local read "LAB02-2 (SIG)"() -> (w2548:T2)
                        n1553 = local read "LAB02-2 (TDMS)"() -> (w2549:refnum<k34>)
                        n1554 = Build Array("TEMP Neut") -> (w2513:string[])
                        n1555 = Build Array("CYCLE") -> (w2508:string[])
                        n1556 = Build Array("TEMP Live") -> (w2518:string[])
                        n1557 = Build Array("PF") -> (w2523:string[])
                        n1558 = Build Array("AMPS") -> (w2544:string[])
                        n1559 = Build Array("VOLTS") -> (w2535:string[])
                        n1560 = Unbundle(w2548) -> ("AMPS"=w2543:dbl, "VOLTS"=w2532:dbl, "PF"=w2531:dbl, "Tmp Live"=w2530:dbl, "Tmp Neut"=w2533:dbl)
                        n1561 = Unbundle(w2547) -> ("CYCLE"=w2528:dbl)  [unwired: 2 out]
                        n1562 = Build Array(w2532) -> (w2529:dbl[])
                        n1563 = Build Array(w2531) -> (w2522:dbl[])
                        n1564 = Build Array(w2530) -> (w2517:dbl[])
                        n1565 = Build Array(w2533) -> (w2512:dbl[])
                        n1566 = Build Array(w2543) -> (w2542:dbl[])
                        n1567 = Build Array(w2528) -> (w2507:dbl[])
                        n1568 = TDMS Write(0:w2549, 5:"LAB02-2 TEST VALUES", 7:w2544, 9:w2542) -> (4:w2537:refnum<k34>, 6:w2536:string, 15:w2524:errorcluster)  [unwired: 2 in, 1 out]
                        n1569 = TDMS Write(0:w2537, 5:w2536, 7:w2535, 9:w2529, 11:w2524) -> (4:w2527:refnum<k34>, 6:w2526:string, 15:w2525:errorcluster)  [unwired: 1 in, 1 out]
                        n1570 = TDMS Write(0:w2527, 5:w2526, 7:w2523, 9:w2522, 11:w2525) -> (4:w2521:refnum<k34>, 6:w2520:string, 15:w2519:errorcluster)  [unwired: 1 in, 1 out]
                        n1571 = TDMS Write(0:w2521, 5:w2520, 7:w2518, 9:w2517, 11:w2519) -> (4:w2516:refnum<k34>, 6:w2515:string, 15:w2514:errorcluster)  [unwired: 1 in, 1 out]
                        n1572 = TDMS Write(0:w2516, 5:w2515, 7:w2513, 9:w2512, 11:w2514) -> (4:w2511:refnum<k34>, 6:w2510:string, 15:w2509:errorcluster)  [unwired: 1 in, 1 out]
                        n1573 = TDMS Write(0:w2511, 5:w2510, 7:w2508, 9:w2507, 11:w2509) -> (15:w2506:errorcluster)  [unwired: 1 in, 3 out]
                        n1574 = local write "data file error"(w2506) -> ()
                      }
                    }
                  }
                  frame #4 {
                    # "LAB03-1"
                    n1575 = case shown="True" w2550 {
                      frame False {
                      }
                      frame True {
                        n1576 = local read "LAB03-1 (DISP)"() -> (w2592:T4)
                        n1577 = local read "LAB03-1 (SIG)"() -> (w2593:T2)
                        n1578 = local read "LAB03-1 (TDMS)"() -> (w2594:refnum<k34>)
                        n1579 = Build Array("TEMP Neut") -> (w2558:string[])
                        n1580 = Build Array("CYCLE") -> (w2553:string[])
                        n1581 = Build Array("TEMP Live") -> (w2563:string[])
                        n1582 = Build Array("PF") -> (w2568:string[])
                        n1583 = Build Array("AMPS") -> (w2589:string[])
                        n1584 = Build Array("VOLTS") -> (w2580:string[])
                        n1585 = Unbundle(w2593) -> ("AMPS"=w2588:dbl, "VOLTS"=w2577:dbl, "PF"=w2576:dbl, "Tmp Live"=w2575:dbl, "Tmp Neut"=w2578:dbl)
                        n1586 = Unbundle(w2592) -> ("CYCLE"=w2573:dbl)  [unwired: 2 out]
                        n1587 = Build Array(w2577) -> (w2574:dbl[])
                        n1588 = Build Array(w2576) -> (w2567:dbl[])
                        n1589 = Build Array(w2575) -> (w2562:dbl[])
                        n1590 = Build Array(w2578) -> (w2557:dbl[])
                        n1591 = Build Array(w2588) -> (w2587:dbl[])
                        n1592 = Build Array(w2573) -> (w2552:dbl[])
                        n1593 = TDMS Write(0:w2594, 5:"LAB03-1 TEST VALUES", 7:w2589, 9:w2587) -> (4:w2582:refnum<k34>, 6:w2581:string, 15:w2569:errorcluster)  [unwired: 2 in, 1 out]
                        n1594 = TDMS Write(0:w2582, 5:w2581, 7:w2580, 9:w2574, 11:w2569) -> (4:w2572:refnum<k34>, 6:w2571:string, 15:w2570:errorcluster)  [unwired: 1 in, 1 out]
                        n1595 = TDMS Write(0:w2572, 5:w2571, 7:w2568, 9:w2567, 11:w2570) -> (4:w2566:refnum<k34>, 6:w2565:string, 15:w2564:errorcluster)  [unwired: 1 in, 1 out]
                        n1596 = TDMS Write(0:w2566, 5:w2565, 7:w2563, 9:w2562, 11:w2564) -> (4:w2561:refnum<k34>, 6:w2560:string, 15:w2559:errorcluster)  [unwired: 1 in, 1 out]
                        n1597 = TDMS Write(0:w2561, 5:w2560, 7:w2558, 9:w2557, 11:w2559) -> (4:w2556:refnum<k34>, 6:w2555:string, 15:w2554:errorcluster)  [unwired: 1 in, 1 out]
                        n1598 = TDMS Write(0:w2556, 5:w2555, 7:w2553, 9:w2552, 11:w2554) -> (15:w2551:errorcluster)  [unwired: 1 in, 3 out]
                        n1599 = local write "data file error"(w2551) -> ()
                      }
                    }
                  }
                  frame #5 {
                    # "LAB03-2"
                    n1600 = case shown="True" w2595 {
                      frame False {
                      }
                      frame True {
                        n1601 = local read "LAB03-2 (DISP)"() -> (w2637:T4)
                        n1602 = local read "LAB03-2 (SIG)"() -> (w2638:T2)
                        n1603 = local read "LAB03-2 (TDMS)"() -> (w2639:refnum<k34>)
                        n1604 = Build Array("TEMP Neut") -> (w2603:string[])
                        n1605 = Build Array("CYCLE") -> (w2598:string[])
                        n1606 = Build Array("TEMP Live") -> (w2608:string[])
                        n1607 = Build Array("PF") -> (w2613:string[])
                        n1608 = Build Array("AMPS") -> (w2634:string[])
                        n1609 = Build Array("VOLTS") -> (w2625:string[])
                        n1610 = Unbundle(w2638) -> ("AMPS"=w2633:dbl, "VOLTS"=w2622:dbl, "PF"=w2621:dbl, "Tmp Live"=w2620:dbl, "Tmp Neut"=w2623:dbl)
                        n1611 = Unbundle(w2637) -> ("CYCLE"=w2618:dbl)  [unwired: 2 out]
                        n1612 = Build Array(w2622) -> (w2619:dbl[])
                        n1613 = Build Array(w2621) -> (w2612:dbl[])
                        n1614 = Build Array(w2620) -> (w2607:dbl[])
                        n1615 = Build Array(w2623) -> (w2602:dbl[])
                        n1616 = Build Array(w2633) -> (w2632:dbl[])
                        n1617 = Build Array(w2618) -> (w2597:dbl[])
                        n1618 = TDMS Write(0:w2639, 5:"LAB03-2 TEST VALUES", 7:w2634, 9:w2632) -> (4:w2627:refnum<k34>, 6:w2626:string, 15:w2614:errorcluster)  [unwired: 2 in, 1 out]
                        n1619 = TDMS Write(0:w2627, 5:w2626, 7:w2625, 9:w2619, 11:w2614) -> (4:w2617:refnum<k34>, 6:w2616:string, 15:w2615:errorcluster)  [unwired: 1 in, 1 out]
                        n1620 = TDMS Write(0:w2617, 5:w2616, 7:w2613, 9:w2612, 11:w2615) -> (4:w2611:refnum<k34>, 6:w2610:string, 15:w2609:errorcluster)  [unwired: 1 in, 1 out]
                        n1621 = TDMS Write(0:w2611, 5:w2610, 7:w2608, 9:w2607, 11:w2609) -> (4:w2606:refnum<k34>, 6:w2605:string, 15:w2604:errorcluster)  [unwired: 1 in, 1 out]
                        n1622 = TDMS Write(0:w2606, 5:w2605, 7:w2603, 9:w2602, 11:w2604) -> (4:w2601:refnum<k34>, 6:w2600:string, 15:w2599:errorcluster)  [unwired: 1 in, 1 out]
                        n1623 = TDMS Write(0:w2601, 5:w2600, 7:w2598, 9:w2597, 11:w2599) -> (15:w2596:errorcluster)  [unwired: 1 in, 3 out]
                        n1624 = local write "data file error"(w2596) -> ()
                      }
                    }
                  }
                  frame #6 {
                    # "LAB04-1"
                    n1625 = case shown="True" w2640 {
                      frame False {
                      }
                      frame True {
                        n1626 = local read "LAB04-1 (DISP)"() -> (w2682:T4)
                        n1627 = local read "LAB04-1 (SIG)"() -> (w2683:T2)
                        n1628 = local read "LAB04-1 (TDMS)"() -> (w2684:refnum<k34>)
                        n1629 = Build Array("TEMP Neut") -> (w2648:string[])
                        n1630 = Build Array("CYCLE") -> (w2643:string[])
                        n1631 = Build Array("TEMP Live") -> (w2653:string[])
                        n1632 = Build Array("PF") -> (w2658:string[])
                        n1633 = Build Array("AMPS") -> (w2679:string[])
                        n1634 = Build Array("VOLTS") -> (w2670:string[])
                        n1635 = Unbundle(w2683) -> ("AMPS"=w2678:dbl, "VOLTS"=w2667:dbl, "PF"=w2666:dbl, "Tmp Live"=w2665:dbl, "Tmp Neut"=w2668:dbl)
                        n1636 = Unbundle(w2682) -> ("CYCLE"=w2663:dbl)  [unwired: 2 out]
                        n1637 = Build Array(w2667) -> (w2664:dbl[])
                        n1638 = Build Array(w2666) -> (w2657:dbl[])
                        n1639 = Build Array(w2665) -> (w2652:dbl[])
                        n1640 = Build Array(w2668) -> (w2647:dbl[])
                        n1641 = Build Array(w2678) -> (w2677:dbl[])
                        n1642 = Build Array(w2663) -> (w2642:dbl[])
                        n1643 = TDMS Write(0:w2684, 5:"LAB04-1 TEST VALUES", 7:w2679, 9:w2677) -> (4:w2672:refnum<k34>, 6:w2671:string, 15:w2659:errorcluster)  [unwired: 2 in, 1 out]
                        n1644 = TDMS Write(0:w2672, 5:w2671, 7:w2670, 9:w2664, 11:w2659) -> (4:w2662:refnum<k34>, 6:w2661:string, 15:w2660:errorcluster)  [unwired: 1 in, 1 out]
                        n1645 = TDMS Write(0:w2662, 5:w2661, 7:w2658, 9:w2657, 11:w2660) -> (4:w2656:refnum<k34>, 6:w2655:string, 15:w2654:errorcluster)  [unwired: 1 in, 1 out]
                        n1646 = TDMS Write(0:w2656, 5:w2655, 7:w2653, 9:w2652, 11:w2654) -> (4:w2651:refnum<k34>, 6:w2650:string, 15:w2649:errorcluster)  [unwired: 1 in, 1 out]
                        n1647 = TDMS Write(0:w2651, 5:w2650, 7:w2648, 9:w2647, 11:w2649) -> (4:w2646:refnum<k34>, 6:w2645:string, 15:w2644:errorcluster)  [unwired: 1 in, 1 out]
                        n1648 = TDMS Write(0:w2646, 5:w2645, 7:w2643, 9:w2642, 11:w2644) -> (15:w2641:errorcluster)  [unwired: 1 in, 3 out]
                        n1649 = local write "data file error"(w2641) -> ()
                      }
                    }
                  }
                  frame #7 {
                    # "LAB04-2"
                    n1650 = case shown="True" w2685 {
                      frame False {
                      }
                      frame True {
                        n1651 = local read "LAB04-2 (DISP)"() -> (w2727:T4)
                        n1652 = local read "LAB04-2 (SIG)"() -> (w2728:T2)
                        n1653 = local read "LAB04-2 (TDMS)"() -> (w2729:refnum<k34>)
                        n1654 = Build Array("TEMP Neut") -> (w2693:string[])
                        n1655 = Build Array("CYCLE") -> (w2688:string[])
                        n1656 = Build Array("TEMP Live") -> (w2698:string[])
                        n1657 = Build Array("PF") -> (w2703:string[])
                        n1658 = Build Array("AMPS") -> (w2724:string[])
                        n1659 = Build Array("VOLTS") -> (w2715:string[])
                        n1660 = Unbundle(w2728) -> ("AMPS"=w2723:dbl, "VOLTS"=w2712:dbl, "PF"=w2711:dbl, "Tmp Live"=w2710:dbl, "Tmp Neut"=w2713:dbl)
                        n1661 = Unbundle(w2727) -> ("CYCLE"=w2708:dbl)  [unwired: 2 out]
                        n1662 = Build Array(w2712) -> (w2709:dbl[])
                        n1663 = Build Array(w2711) -> (w2702:dbl[])
                        n1664 = Build Array(w2710) -> (w2697:dbl[])
                        n1665 = Build Array(w2713) -> (w2692:dbl[])
                        n1666 = Build Array(w2723) -> (w2722:dbl[])
                        n1667 = Build Array(w2708) -> (w2687:dbl[])
                        n1668 = TDMS Write(0:w2729, 5:"LAB04-2 TEST VALUES", 7:w2724, 9:w2722) -> (4:w2717:refnum<k34>, 6:w2716:string, 15:w2704:errorcluster)  [unwired: 2 in, 1 out]
                        n1669 = TDMS Write(0:w2717, 5:w2716, 7:w2715, 9:w2709, 11:w2704) -> (4:w2707:refnum<k34>, 6:w2706:string, 15:w2705:errorcluster)  [unwired: 1 in, 1 out]
                        n1670 = TDMS Write(0:w2707, 5:w2706, 7:w2703, 9:w2702, 11:w2705) -> (4:w2701:refnum<k34>, 6:w2700:string, 15:w2699:errorcluster)  [unwired: 1 in, 1 out]
                        n1671 = TDMS Write(0:w2701, 5:w2700, 7:w2698, 9:w2697, 11:w2699) -> (4:w2696:refnum<k34>, 6:w2695:string, 15:w2694:errorcluster)  [unwired: 1 in, 1 out]
                        n1672 = TDMS Write(0:w2696, 5:w2695, 7:w2693, 9:w2692, 11:w2694) -> (4:w2691:refnum<k34>, 6:w2690:string, 15:w2689:errorcluster)  [unwired: 1 in, 1 out]
                        n1673 = TDMS Write(0:w2691, 5:w2690, 7:w2688, 9:w2687, 11:w2689) -> (15:w2686:errorcluster)  [unwired: 1 in, 3 out]
                        n1674 = local write "data file error"(w2686) -> ()
                      }
                    }
                  }
                  frame #8 {
                    # "LAB05-1"
                    n1675 = case shown="True" w2730 {
                      frame False {
                      }
                      frame True {
                        n1676 = local read "LAB05-1 (DISP)"() -> (w2772:T4)
                        n1677 = local read "LAB05-1 (SIG)"() -> (w2773:T2)
                        n1678 = local read "LAB05-1 (TDMS)"() -> (w2774:refnum<k34>)
                        n1679 = Build Array("TEMP Neut") -> (w2738:string[])
                        n1680 = Build Array("CYCLE") -> (w2733:string[])
                        n1681 = Build Array("TEMP Live") -> (w2743:string[])
                        n1682 = Build Array("PF") -> (w2748:string[])
                        n1683 = Build Array("AMPS") -> (w2769:string[])
                        n1684 = Build Array("VOLTS") -> (w2760:string[])
                        n1685 = Unbundle(w2773) -> ("AMPS"=w2768:dbl, "VOLTS"=w2757:dbl, "PF"=w2756:dbl, "Tmp Live"=w2755:dbl, "Tmp Neut"=w2758:dbl)
                        n1686 = Unbundle(w2772) -> ("CYCLE"=w2753:dbl)  [unwired: 2 out]
                        n1687 = Build Array(w2757) -> (w2754:dbl[])
                        n1688 = Build Array(w2756) -> (w2747:dbl[])
                        n1689 = Build Array(w2755) -> (w2742:dbl[])
                        n1690 = Build Array(w2758) -> (w2737:dbl[])
                        n1691 = Build Array(w2768) -> (w2767:dbl[])
                        n1692 = Build Array(w2753) -> (w2732:dbl[])
                        n1693 = TDMS Write(0:w2774, 5:"LAB05-1 TEST VALUES", 7:w2769, 9:w2767) -> (4:w2762:refnum<k34>, 6:w2761:string, 15:w2749:errorcluster)  [unwired: 2 in, 1 out]
                        n1694 = TDMS Write(0:w2762, 5:w2761, 7:w2760, 9:w2754, 11:w2749) -> (4:w2752:refnum<k34>, 6:w2751:string, 15:w2750:errorcluster)  [unwired: 1 in, 1 out]
                        n1695 = TDMS Write(0:w2752, 5:w2751, 7:w2748, 9:w2747, 11:w2750) -> (4:w2746:refnum<k34>, 6:w2745:string, 15:w2744:errorcluster)  [unwired: 1 in, 1 out]
                        n1696 = TDMS Write(0:w2746, 5:w2745, 7:w2743, 9:w2742, 11:w2744) -> (4:w2741:refnum<k34>, 6:w2740:string, 15:w2739:errorcluster)  [unwired: 1 in, 1 out]
                        n1697 = TDMS Write(0:w2741, 5:w2740, 7:w2738, 9:w2737, 11:w2739) -> (4:w2736:refnum<k34>, 6:w2735:string, 15:w2734:errorcluster)  [unwired: 1 in, 1 out]
                        n1698 = TDMS Write(0:w2736, 5:w2735, 7:w2733, 9:w2732, 11:w2734) -> (15:w2731:errorcluster)  [unwired: 1 in, 3 out]
                        n1699 = local write "data file error"(w2731) -> ()
                      }
                    }
                  }
                  frame #9 {
                    # "LAB05-2"
                    n1700 = case shown="True" w2775 {
                      frame False {
                      }
                      frame True {
                        n1701 = local read "LAB05-2 (DISP)"() -> (w2817:T4)
                        n1702 = local read "LAB05-2 (SIG)"() -> (w2818:T2)
                        n1703 = local read "LAB05-2 (TDMS)"() -> (w2819:refnum<k34>)
                        n1704 = Build Array("TEMP Neut") -> (w2783:string[])
                        n1705 = Build Array("CYCLE") -> (w2778:string[])
                        n1706 = Build Array("TEMP Live") -> (w2788:string[])
                        n1707 = Build Array("PF") -> (w2793:string[])
                        n1708 = Build Array("AMPS") -> (w2814:string[])
                        n1709 = Build Array("VOLTS") -> (w2805:string[])
                        n1710 = Unbundle(w2818) -> ("AMPS"=w2813:dbl, "VOLTS"=w2802:dbl, "PF"=w2801:dbl, "Tmp Live"=w2800:dbl, "Tmp Neut"=w2803:dbl)
                        n1711 = Unbundle(w2817) -> ("CYCLE"=w2798:dbl)  [unwired: 2 out]
                        n1712 = Build Array(w2802) -> (w2799:dbl[])
                        n1713 = Build Array(w2801) -> (w2792:dbl[])
                        n1714 = Build Array(w2800) -> (w2787:dbl[])
                        n1715 = Build Array(w2803) -> (w2782:dbl[])
                        n1716 = Build Array(w2813) -> (w2812:dbl[])
                        n1717 = Build Array(w2798) -> (w2777:dbl[])
                        n1718 = TDMS Write(0:w2819, 5:"LAB05-2 TEST VALUES", 7:w2814, 9:w2812) -> (4:w2807:refnum<k34>, 6:w2806:string, 15:w2794:errorcluster)  [unwired: 2 in, 1 out]
                        n1719 = TDMS Write(0:w2807, 5:w2806, 7:w2805, 9:w2799, 11:w2794) -> (4:w2797:refnum<k34>, 6:w2796:string, 15:w2795:errorcluster)  [unwired: 1 in, 1 out]
                        n1720 = TDMS Write(0:w2797, 5:w2796, 7:w2793, 9:w2792, 11:w2795) -> (4:w2791:refnum<k34>, 6:w2790:string, 15:w2789:errorcluster)  [unwired: 1 in, 1 out]
                        n1721 = TDMS Write(0:w2791, 5:w2790, 7:w2788, 9:w2787, 11:w2789) -> (4:w2786:refnum<k34>, 6:w2785:string, 15:w2784:errorcluster)  [unwired: 1 in, 1 out]
                        n1722 = TDMS Write(0:w2786, 5:w2785, 7:w2783, 9:w2782, 11:w2784) -> (4:w2781:refnum<k34>, 6:w2780:string, 15:w2779:errorcluster)  [unwired: 1 in, 1 out]
                        n1723 = TDMS Write(0:w2781, 5:w2780, 7:w2778, 9:w2777, 11:w2779) -> (15:w2776:errorcluster)  [unwired: 1 in, 3 out]
                        n1724 = local write "data file error"(w2776) -> ()
                      }
                    }
                  }
                }
              }
            }
          }
          frame #13 {
            # "check for cycle test fail conditions"
            n1725 = local read "on loops"() -> (w2846:dbl)
            n1726 = local read "jig cycle"() -> (w2843:dbl)
            n1727 = local read "jig cycle"() -> (w2848:dbl)
            n1728 = Add(x=w2846, y=3.0) -> (x+y=w2844:dbl)
            n1729 = Equal?(x=w2843, y=w2844) -> (x = y?=w2839:bool)
            n1730 = Equal?(x=w2848, y=1.0) -> (x = y?=w2841:bool)
            n1731 = stacked-sequence {
              tunnel: w2842 -> [w2850 _ _ _ _ _ _ _ _ _]
              tunnel: w2841 -> [w2854 w2918 w2969 w3020 w3071 w3122 w3173 w3224 w3275 w3326]
              tunnel: w2840 -> [w2860 _ _ _ _ _ _ _ _ _]
              tunnel: w2839 -> [w2853 w2917 w2968 w3019 w3070 w3121 w3172 w3223 w3274 w3325]
              tunnel: w2838 -> [_ w2914 _ _ _ _ _ _ _ _]
              tunnel: w2837 -> [_ w2913 _ _ _ _ _ _ _ _]
              tunnel: w2836 -> [_ _ w2965 _ _ _ _ _ _ _]
              tunnel: w2835 -> [_ _ w2964 _ _ _ _ _ _ _]
              tunnel: w2834 -> [_ _ _ w3016 _ _ _ _ _ _]
              tunnel: w2833 -> [_ _ _ w3015 _ _ _ _ _ _]
              tunnel: w2832 -> [_ _ _ _ w3067 _ _ _ _ _]
              tunnel: w2831 -> [_ _ _ _ w3066 _ _ _ _ _]
              tunnel: w2830 -> [_ _ _ _ _ w3118 _ _ _ _]
              tunnel: w2829 -> [_ _ _ _ _ w3117 _ _ _ _]
              tunnel: w2828 -> [_ _ _ _ _ _ w3169 _ _ _]
              tunnel: w2827 -> [_ _ _ _ _ _ w3168 _ _ _]
              tunnel: w2826 -> [_ _ _ _ _ _ _ w3220 _ _]
              tunnel: w2825 -> [_ _ _ _ _ _ _ w3219 _ _]
              tunnel: w2824 -> [_ _ _ _ _ _ _ _ w3271 _]
              tunnel: w2823 -> [_ _ _ _ _ _ _ _ w3270 _]
              tunnel: w2822 -> [_ _ _ _ _ _ _ _ _ w3322]
              tunnel: w2821 -> [_ _ _ _ _ _ _ _ _ w3321]
              tunnel: 2.0 -> [w2849 w2912 w2963 w3014 w3065 w3116 w3167 w3218 w3269 w3320]
              frame #0 {
                # "check for amps fail"
                # "LAB01-1"
                n1732 = local read "LAB01-1 (SIG)"() -> (w2856:T2)
                n1733 = Or(x=w2854, y=w2853) -> (x .or. y?=w2858:bool)
                n1734 = case shown="\"CYCLE TEST\"" w2850 {
                  tunnel: [FALSE TRUE FALSE] -> w2851
                  frame "TEST SET UP", Default {
                  }
                  frame "CYCLE TEST" {
                  }
                  frame "T-RISE TEST" {
                  }
                }
                n1735 = And(x=w2860, y=w2858) -> (x .and. y?=w2857:bool)
                n1736 = local read "LAB01-1 (TDMS)"() -> (w2852:refnum<k34>)
                n1737 = Unbundle(w2856) -> ("AMPS"=w2855:dbl)  [unwired: 4 out]
                n1738 = And(x=w2851, y=w2857) -> (x .and. y?=w2859:bool)
                n1739 = case shown="True" w2859 {
                  tunnel: w2855 -> [_ w2872]
                  tunnel: w2854 -> [_ w2874]
                  tunnel: w2853 -> [_ w2873]
                  tunnel: w2852 -> [_ w2869]
                  tunnel: w2849 -> [_ w2868]
                  tunnel: w2849 -> [_ w2867]
                  frame False {
                  }
                  frame True {
                    w2861 = 5.0
                    n1740 = case shown="True" w2874 {
                      tunnel: w2872 -> [_ w2892]
                      tunnel: ["" "AMPS LO"] -> w2870
                      tunnel: w2867 -> [_ w2890]
                      frame False {
                        (unwired) FALSE
                      }
                      frame True {
                        n1741 = Less?(x=w2892, y=w2890) -> (x < y?=w2889:bool)
                        n1742 = local read "LAB01-1 (FAIL LO)"() -> (w2888:dbl)
                        n1743 = Increment(x=w2888) -> (x+1=w2886:dbl)
                        n1744 = Select(t=w2886, s=w2889, f=0.0) -> (s? t:f=w2887:dbl)
                        n1745 = local write "LAB01-1 (FAIL LO)"(w2887) -> ()
                      }
                    }
                    n1746 = case shown="True" w2873 {
                      tunnel: w2872 -> [_ w2883]
                      tunnel: ["" "AMPS HI"] -> w2871
                      tunnel: w2868 -> [_ w2881]
                      frame False {
                        (unwired) FALSE
                      }
                      frame True {
                        n1747 = Greater?(x=w2883, y=w2881) -> (0:w2879:bool)
                        n1748 = local read "LAB01-1 (FAIL HI)"() -> (w2880:dbl)
                        n1749 = Increment(x=w2880) -> (x+1=w2877:dbl)
                        n1750 = Select(t=w2877, s=w2879, f=0.0) -> (s? t:f=w2878:dbl)
                        n1751 = local write "LAB01-1 (FAIL HI)"(w2878) -> ()
                      }
                    }
                    n1752 = local read "LAB01-1 (FAIL LO)"() -> (w2863:dbl)
                    n1753 = local read "LAB01-1 (FAIL HI)"() -> (w2862:dbl)
                    n1754 = Greater Or Equal?(x=w2863, y=w2861) -> (x >= y?=w2866:bool)
                    n1755 = Greater Or Equal?(x=w2862, y=w2861) -> (x >= y?=w2865:bool)
                    n1756 = Or(x=w2866, y=w2865) -> (x .or. y?=w2864:bool)
                    n1757 = case shown="True" w2864 {
                      tunnel: w2871 -> [_ w2895]
                      tunnel: w2870 -> [_ w2894]
                      tunnel: w2869 -> [_ w2893]
                      frame False {
                      }
                      frame True {
                        n1758 = stacked-sequence {
                          tunnel: w2895 -> [w2900 w2905]
                          tunnel: w2894 -> [w2899 w2904]
                          tunnel: w2893 -> [w2896 _]
                          frame #0 {
                            n1759 = Build Array(w2900, w2899) -> (w2898:string[])
                            n1760 = TDMS Write(0:w2896, 5:"TEST RESULT", 7:"AMPS FAIL ", 9:w2898) -> (15:w2902:errorcluster)  [unwired: 2 in, 3 out]
                            n1761 = local write "data file error"(w2902) -> ()
                          }
                          frame #1 {
                            (unwired) "STOP"
                            n1762 = local read "LAB01-1 (DISP)"() -> (w2908:T4)
                            n1763 = Concatenate Strings(w2905, w2904) -> (w2903:string)
                            n1764 = Bundle(cluster=w2908, "STATUS"=w2903) -> (w2907:T4)  [unwired: 2 in]
                            n1765 = local write "LAB01-1 (RESULT)"(FALSE) -> ()
                            n1766 = local write "LAB01-1 (DISP)"(w2907) -> ()
                          }
                        }
                      }
                    }
                  }
                }
              }
              frame #1 {
                # "LAB01-2"
                n1767 = local read "LAB01-2 (SIG)"() -> (w2920:T2)
                n1768 = Or(x=w2918, y=w2917) -> (x .or. y?=w2922:bool)
                n1769 = case shown="\"CYCLE TEST\"" w2913 {
                  tunnel: [FALSE TRUE FALSE] -> w2915
                  frame "TEST SET UP", Default {
                  }
                  frame "CYCLE TEST" {
                  }
                  frame "T-RISE TEST" {
                  }
                }
                n1770 = And(x=w2914, y=w2922) -> (x .and. y?=w2921:bool)
                n1771 = local read "LAB01-2 (TDMS)"() -> (w2916:refnum<k34>)
                n1772 = Unbundle(w2920) -> ("AMPS"=w2919:dbl)  [unwired: 4 out]
                n1773 = And(x=w2915, y=w2921) -> (x .and. y?=w2923:bool)
                n1774 = case shown="True" w2923 {
                  tunnel: w2919 -> [_ w2931]
                  tunnel: w2918 -> [_ w2933]
                  tunnel: w2917 -> [_ w2932]
                  tunnel: w2916 -> [_ w2925]
                  tunnel: w2912 -> [_ w2924]
                  frame False {
                  }
                  frame True {
                    # "check for amps fail"
                    n1775 = case shown="True" w2932 {
                      tunnel: w2931 -> [_ w2939]
                      tunnel: [FALSE w2938] -> w2929
                      tunnel: ["" "AMPS HI"] -> w2927
                      tunnel: w2924 -> [_ w2936]
                      frame False {
                      }
                      frame True {
                        n1776 = Greater?(x=w2939, y=w2936) -> (0:w2938:bool)
                      }
                    }
                    n1777 = case shown="True" w2933 {
                      tunnel: w2931 -> [_ w2945]
                      tunnel: [FALSE w2944] -> w2930
                      tunnel: ["" "AMPS LO"] -> w2926
                      tunnel: w2924 -> [_ w2942]
                      frame False {
                      }
                      frame True {
                        n1778 = Less?(x=w2945, y=w2942) -> (x < y?=w2944:bool)
                      }
                    }
                    n1779 = Or(x=w2930, y=w2929) -> (x .or. y?=w2928:bool)
                    n1780 = case shown="True" w2928 {
                      tunnel: w2927 -> [_ w2948]
                      tunnel: w2926 -> [_ w2947]
                      tunnel: w2925 -> [_ w2946]
                      frame False {
                      }
                      frame True {
                        n1781 = stacked-sequence {
                          tunnel: w2948 -> [w2953 _]
                          tunnel: w2947 -> [w2952 _]
                          tunnel: w2946 -> [w2949 _]
                          frame #0 {
                            n1782 = Build Array(w2953, w2952) -> (w2951:string[])
                            n1783 = TDMS Write(0:w2949, 5:"TEST RESULT", 7:"AMPS FAIL ", 9:w2951) -> (15:w2955:errorcluster)  [unwired: 2 in, 3 out]
                            n1784 = local write "data file error"(w2955) -> ()
                          }
                          frame #1 {
                            n1785 = local read "LAB01-2 (DISP)"() -> (w2959:T4)
                            n1786 = Bundle(cluster=w2959, "STATUS"="STOP") -> (w2958:T4)  [unwired: 2 in]
                            n1787 = local write "LAB01-2 (RESULT)"(FALSE) -> ()
                            n1788 = local write "LAB01-2 (DISP)"(w2958) -> ()
                          }
                        }
                      }
                    }
                  }
                }
              }
              frame #2 {
                # "LAB02-1"
                n1789 = local read "LAB02-1 (SIG)"() -> (w2971:T2)
                n1790 = Or(x=w2969, y=w2968) -> (x .or. y?=w2973:bool)
                n1791 = case shown="\"CYCLE TEST\"" w2964 {
                  tunnel: [FALSE TRUE FALSE] -> w2966
                  frame "TEST SET UP", Default {
                  }
                  frame "CYCLE TEST" {
                  }
                  frame "T-RISE TEST" {
                  }
                }
                n1792 = And(x=w2965, y=w2973) -> (x .and. y?=w2972:bool)
                n1793 = local read "LAB02-1 (TDMS)"() -> (w2967:refnum<k34>)
                n1794 = Unbundle(w2971) -> ("AMPS"=w2970:dbl)  [unwired: 4 out]
                n1795 = And(x=w2966, y=w2972) -> (x .and. y?=w2974:bool)
                n1796 = case shown="True" w2974 {
                  tunnel: w2970 -> [_ w2982]
                  tunnel: w2969 -> [_ w2984]
                  tunnel: w2968 -> [_ w2983]
                  tunnel: w2967 -> [_ w2976]
                  tunnel: w2963 -> [_ w2975]
                  frame False {
                  }
                  frame True {
                    # "check for amps fail"
                    n1797 = case shown="True" w2983 {
                      tunnel: w2982 -> [_ w2990]
                      tunnel: [FALSE w2989] -> w2980
                      tunnel: ["" "AMPS HI"] -> w2978
                      tunnel: w2975 -> [_ w2987]
                      frame False {
                      }
                      frame True {
                        n1798 = Greater?(x=w2990, y=w2987) -> (0:w2989:bool)
                      }
                    }
                    n1799 = case shown="True" w2984 {
                      tunnel: w2982 -> [_ w2996]
                      tunnel: [FALSE w2995] -> w2981
                      tunnel: ["" "AMPS LO"] -> w2977
                      tunnel: w2975 -> [_ w2993]
                      frame False {
                      }
                      frame True {
                        n1800 = Less?(x=w2996, y=w2993) -> (x < y?=w2995:bool)
                      }
                    }
                    n1801 = Or(x=w2981, y=w2980) -> (x .or. y?=w2979:bool)
                    n1802 = case shown="True" w2979 {
                      tunnel: w2978 -> [_ w2999]
                      tunnel: w2977 -> [_ w2998]
                      tunnel: w2976 -> [_ w2997]
                      frame False {
                      }
                      frame True {
                        n1803 = stacked-sequence {
                          tunnel: w2999 -> [w3004 _]
                          tunnel: w2998 -> [w3003 _]
                          tunnel: w2997 -> [w3000 _]
                          frame #0 {
                            n1804 = Build Array(w3004, w3003) -> (w3002:string[])
                            n1805 = TDMS Write(0:w3000, 5:"TEST RESULT", 7:"AMPS FAIL ", 9:w3002) -> (15:w3006:errorcluster)  [unwired: 2 in, 3 out]
                            n1806 = local write "data file error"(w3006) -> ()
                          }
                          frame #1 {
                            n1807 = local read "LAB02-1 (DISP)"() -> (w3010:T4)
                            n1808 = Bundle(cluster=w3010, "STATUS"="STOP") -> (w3009:T4)  [unwired: 2 in]
                            n1809 = local write "LAB02-1 (RESULT)"(FALSE) -> ()
                            n1810 = local write "LAB02-1 (DISP)"(w3009) -> ()
                          }
                        }
                      }
                    }
                  }
                }
              }
              frame #3 {
                # "LAB02-2"
                n1811 = local read "LAB02-2 (SIG)"() -> (w3022:T2)
                n1812 = Or(x=w3020, y=w3019) -> (x .or. y?=w3024:bool)
                n1813 = case shown="\"CYCLE TEST\"" w3015 {
                  tunnel: [FALSE TRUE FALSE] -> w3017
                  frame "TEST SET UP", Default {
                  }
                  frame "CYCLE TEST" {
                  }
                  frame "T-RISE TEST" {
                  }
                }
                n1814 = And(x=w3016, y=w3024) -> (x .and. y?=w3023:bool)
                n1815 = local read "LAB02-2 (TDMS)"() -> (w3018:refnum<k34>)
                n1816 = Unbundle(w3022) -> ("AMPS"=w3021:dbl)  [unwired: 4 out]
                n1817 = And(x=w3017, y=w3023) -> (x .and. y?=w3025:bool)
                n1818 = case shown="True" w3025 {
                  tunnel: w3021 -> [_ w3033]
                  tunnel: w3020 -> [_ w3035]
                  tunnel: w3019 -> [_ w3034]
                  tunnel: w3018 -> [_ w3027]
                  tunnel: w3014 -> [_ w3026]
                  frame False {
                  }
                  frame True {
                    # "check for amps fail"
                    n1819 = case shown="True" w3034 {
                      tunnel: w3033 -> [_ w3041]
                      tunnel: [FALSE w3040] -> w3031
                      tunnel: ["" "AMPS HI"] -> w3029
                      tunnel: w3026 -> [_ w3038]
                      frame False {
                      }
                      frame True {
                        n1820 = Greater?(x=w3041, y=w3038) -> (0:w3040:bool)
                      }
                    }
                    n1821 = case shown="True" w3035 {
                      tunnel: w3033 -> [_ w3047]
                      tunnel: [FALSE w3046] -> w3032
                      tunnel: ["" "AMPS LO"] -> w3028
                      tunnel: w3026 -> [_ w3044]
                      frame False {
                      }
                      frame True {
                        n1822 = Less?(x=w3047, y=w3044) -> (x < y?=w3046:bool)
                      }
                    }
                    n1823 = Or(x=w3032, y=w3031) -> (x .or. y?=w3030:bool)
                    n1824 = case shown="True" w3030 {
                      tunnel: w3029 -> [_ w3050]
                      tunnel: w3028 -> [_ w3049]
                      tunnel: w3027 -> [_ w3048]
                      frame False {
                      }
                      frame True {
                        n1825 = stacked-sequence {
                          tunnel: w3050 -> [w3055 _]
                          tunnel: w3049 -> [w3054 _]
                          tunnel: w3048 -> [w3051 _]
                          frame #0 {
                            n1826 = Build Array(w3055, w3054) -> (w3053:string[])
                            n1827 = TDMS Write(0:w3051, 5:"TEST RESULT", 7:"AMPS FAIL ", 9:w3053) -> (15:w3057:errorcluster)  [unwired: 2 in, 3 out]
                            n1828 = local write "data file error"(w3057) -> ()
                          }
                          frame #1 {
                            n1829 = local read "LAB02-2 (DISP)"() -> (w3061:T4)
                            n1830 = Bundle(cluster=w3061, "STATUS"="STOP") -> (w3060:T4)  [unwired: 2 in]
                            n1831 = local write "LAB02-2 (RESULT)"(FALSE) -> ()
                            n1832 = local write "LAB02-2 (DISP)"(w3060) -> ()
                          }
                        }
                      }
                    }
                  }
                }
              }
              frame #4 {
                # "LAB03-1"
                n1833 = local read "LAB03-1 (SIG)"() -> (w3073:T2)
                n1834 = Or(x=w3071, y=w3070) -> (x .or. y?=w3075:bool)
                n1835 = case shown="\"CYCLE TEST\"" w3066 {
                  tunnel: [FALSE TRUE FALSE] -> w3068
                  frame "TEST SET UP", Default {
                  }
                  frame "CYCLE TEST" {
                  }
                  frame "T-RISE TEST" {
                  }
                }
                n1836 = And(x=w3067, y=w3075) -> (x .and. y?=w3074:bool)
                n1837 = local read "LAB03-1 (TDMS)"() -> (w3069:refnum<k34>)
                n1838 = Unbundle(w3073) -> ("AMPS"=w3072:dbl)  [unwired: 4 out]
                n1839 = And(x=w3068, y=w3074) -> (x .and. y?=w3076:bool)
                n1840 = case shown="True" w3076 {
                  tunnel: w3072 -> [_ w3084]
                  tunnel: w3071 -> [_ w3086]
                  tunnel: w3070 -> [_ w3085]
                  tunnel: w3069 -> [_ w3078]
                  tunnel: w3065 -> [_ w3077]
                  frame False {
                  }
                  frame True {
                    # "check for amps fail"
                    n1841 = case shown="True" w3085 {
                      tunnel: w3084 -> [_ w3092]
                      tunnel: [FALSE w3091] -> w3082
                      tunnel: ["" "AMPS HI"] -> w3080
                      tunnel: w3077 -> [_ w3089]
                      frame False {
                      }
                      frame True {
                        n1842 = Greater?(x=w3092, y=w3089) -> (0:w3091:bool)
                      }
                    }
                    n1843 = case shown="True" w3086 {
                      tunnel: w3084 -> [_ w3098]
                      tunnel: [FALSE w3097] -> w3083
                      tunnel: ["" "AMPS LO"] -> w3079
                      tunnel: w3077 -> [_ w3095]
                      frame False {
                      }
                      frame True {
                        n1844 = Less?(x=w3098, y=w3095) -> (x < y?=w3097:bool)
                      }
                    }
                    n1845 = Or(x=w3083, y=w3082) -> (x .or. y?=w3081:bool)
                    n1846 = case shown="True" w3081 {
                      tunnel: w3080 -> [_ w3101]
                      tunnel: w3079 -> [_ w3100]
                      tunnel: w3078 -> [_ w3099]
                      frame False {
                      }
                      frame True {
                        n1847 = stacked-sequence {
                          tunnel: w3101 -> [w3106 _]
                          tunnel: w3100 -> [w3105 _]
                          tunnel: w3099 -> [w3102 _]
                          frame #0 {
                            n1848 = Build Array(w3106, w3105) -> (w3104:string[])
                            n1849 = TDMS Write(0:w3102, 5:"TEST RESULT", 7:"AMPS FAIL ", 9:w3104) -> (15:w3108:errorcluster)  [unwired: 2 in, 3 out]
                            n1850 = local write "data file error"(w3108) -> ()
                          }
                          frame #1 {
                            n1851 = local read "LAB03-1 (DISP)"() -> (w3112:T4)
                            n1852 = Bundle(cluster=w3112, "STATUS"="STOP") -> (w3111:T4)  [unwired: 2 in]
                            n1853 = local write "LAB03-1 (RESULT)"(FALSE) -> ()
                            n1854 = local write "LAB03-1 (DISP)"(w3111) -> ()
                          }
                        }
                      }
                    }
                  }
                }
              }
              frame #5 {
                # "LAB03-2"
                n1855 = local read "LAB03-2 (SIG)"() -> (w3124:T2)
                n1856 = Or(x=w3122, y=w3121) -> (x .or. y?=w3126:bool)
                n1857 = case shown="\"CYCLE TEST\"" w3117 {
                  tunnel: [FALSE TRUE FALSE] -> w3119
                  frame "TEST SET UP", Default {
                  }
                  frame "CYCLE TEST" {
                  }
                  frame "T-RISE TEST" {
                  }
                }
                n1858 = And(x=w3118, y=w3126) -> (x .and. y?=w3125:bool)
                n1859 = local read "LAB03-2 (TDMS)"() -> (w3120:refnum<k34>)
                n1860 = Unbundle(w3124) -> ("AMPS"=w3123:dbl)  [unwired: 4 out]
                n1861 = And(x=w3119, y=w3125) -> (x .and. y?=w3127:bool)
                n1862 = case shown="True" w3127 {
                  tunnel: w3123 -> [_ w3135]
                  tunnel: w3122 -> [_ w3137]
                  tunnel: w3121 -> [_ w3136]
                  tunnel: w3120 -> [_ w3129]
                  tunnel: w3116 -> [_ w3128]
                  frame False {
                  }
                  frame True {
                    # "check for amps fail"
                    n1863 = case shown="True" w3136 {
                      tunnel: w3135 -> [_ w3143]
                      tunnel: [FALSE w3142] -> w3133
                      tunnel: ["" "AMPS HI"] -> w3131
                      tunnel: w3128 -> [_ w3140]
                      frame False {
                      }
                      frame True {
                        n1864 = Greater?(x=w3143, y=w3140) -> (0:w3142:bool)
                      }
                    }
                    n1865 = case shown="True" w3137 {
                      tunnel: w3135 -> [_ w3149]
                      tunnel: [FALSE w3148] -> w3134
                      tunnel: ["" "AMPS LO"] -> w3130
                      tunnel: w3128 -> [_ w3146]
                      frame False {
                      }
                      frame True {
                        n1866 = Less?(x=w3149, y=w3146) -> (x < y?=w3148:bool)
                      }
                    }
                    n1867 = Or(x=w3134, y=w3133) -> (x .or. y?=w3132:bool)
                    n1868 = case shown="True" w3132 {
                      tunnel: w3131 -> [_ w3152]
                      tunnel: w3130 -> [_ w3151]
                      tunnel: w3129 -> [_ w3150]
                      frame False {
                      }
                      frame True {
                        n1869 = stacked-sequence {
                          tunnel: w3152 -> [w3157 _]
                          tunnel: w3151 -> [w3156 _]
                          tunnel: w3150 -> [w3153 _]
                          frame #0 {
                            n1870 = Build Array(w3157, w3156) -> (w3155:string[])
                            n1871 = TDMS Write(0:w3153, 5:"TEST RESULT", 7:"AMPS FAIL ", 9:w3155) -> (15:w3159:errorcluster)  [unwired: 2 in, 3 out]
                            n1872 = local write "data file error"(w3159) -> ()
                          }
                          frame #1 {
                            n1873 = local read "LAB03-2 (DISP)"() -> (w3163:T4)
                            n1874 = Bundle(cluster=w3163, "STATUS"="STOP") -> (w3162:T4)  [unwired: 2 in]
                            n1875 = local write "LAB03-2 (RESULT)"(FALSE) -> ()
                            n1876 = local write "LAB03-2 (DISP)"(w3162) -> ()
                          }
                        }
                      }
                    }
                  }
                }
              }
              frame #6 {
                # "LAB04-1"
                n1877 = local read "LAB04-1 (SIG)"() -> (w3175:T2)
                n1878 = Or(x=w3173, y=w3172) -> (x .or. y?=w3177:bool)
                n1879 = case shown="\"CYCLE TEST\"" w3168 {
                  tunnel: [FALSE TRUE FALSE] -> w3170
                  frame "TEST SET UP", Default {
                  }
                  frame "CYCLE TEST" {
                  }
                  frame "T-RISE TEST" {
                  }
                }
                n1880 = And(x=w3169, y=w3177) -> (x .and. y?=w3176:bool)
                n1881 = local read "LAB04-1 (TDMS)"() -> (w3171:refnum<k34>)
                n1882 = Unbundle(w3175) -> ("AMPS"=w3174:dbl)  [unwired: 4 out]
                n1883 = And(x=w3170, y=w3176) -> (x .and. y?=w3178:bool)
                n1884 = case shown="True" w3178 {
                  tunnel: w3174 -> [_ w3186]
                  tunnel: w3173 -> [_ w3188]
                  tunnel: w3172 -> [_ w3187]
                  tunnel: w3171 -> [_ w3180]
                  tunnel: w3167 -> [_ w3179]
                  frame False {
                  }
                  frame True {
                    # "check for amps fail"
                    n1885 = case shown="True" w3187 {
                      tunnel: w3186 -> [_ w3194]
                      tunnel: [FALSE w3193] -> w3184
                      tunnel: ["" "AMPS HI"] -> w3182
                      tunnel: w3179 -> [_ w3191]
                      frame False {
                      }
                      frame True {
                        n1886 = Greater?(x=w3194, y=w3191) -> (0:w3193:bool)
                      }
                    }
                    n1887 = case shown="True" w3188 {
                      tunnel: w3186 -> [_ w3200]
                      tunnel: [FALSE w3199] -> w3185
                      tunnel: ["" "AMPS LO"] -> w3181
                      tunnel: w3179 -> [_ w3197]
                      frame False {
                      }
                      frame True {
                        n1888 = Less?(x=w3200, y=w3197) -> (x < y?=w3199:bool)
                      }
                    }
                    n1889 = Or(x=w3185, y=w3184) -> (x .or. y?=w3183:bool)
                    n1890 = case shown="True" w3183 {
                      tunnel: w3182 -> [_ w3203]
                      tunnel: w3181 -> [_ w3202]
                      tunnel: w3180 -> [_ w3201]
                      frame False {
                      }
                      frame True {
                        n1891 = stacked-sequence {
                          tunnel: w3203 -> [w3208 _]
                          tunnel: w3202 -> [w3207 _]
                          tunnel: w3201 -> [w3204 _]
                          frame #0 {
                            n1892 = Build Array(w3208, w3207) -> (w3206:string[])
                            n1893 = TDMS Write(0:w3204, 5:"TEST RESULT", 7:"AMPS FAIL ", 9:w3206) -> (15:w3210:errorcluster)  [unwired: 2 in, 3 out]
                            n1894 = local write "data file error"(w3210) -> ()
                          }
                          frame #1 {
                            n1895 = local read "LAB04-1 (DISP)"() -> (w3214:T4)
                            n1896 = Bundle(cluster=w3214, "STATUS"="STOP") -> (w3213:T4)  [unwired: 2 in]
                            n1897 = local write "LAB04-1 (RESULT)"(FALSE) -> ()
                            n1898 = local write "LAB04-1 (DISP)"(w3213) -> ()
                          }
                        }
                      }
                    }
                  }
                }
              }
              frame #7 {
                # "LAB04-2"
                n1899 = local read "LAB04-2 (SIG)"() -> (w3226:T2)
                n1900 = Or(x=w3224, y=w3223) -> (x .or. y?=w3228:bool)
                n1901 = case shown="\"CYCLE TEST\"" w3219 {
                  tunnel: [FALSE TRUE FALSE] -> w3221
                  frame "TEST SET UP", Default {
                  }
                  frame "CYCLE TEST" {
                  }
                  frame "T-RISE TEST" {
                  }
                }
                n1902 = And(x=w3220, y=w3228) -> (x .and. y?=w3227:bool)
                n1903 = local read "LAB04-2 (TDMS)"() -> (w3222:refnum<k34>)
                n1904 = Unbundle(w3226) -> ("AMPS"=w3225:dbl)  [unwired: 4 out]
                n1905 = And(x=w3221, y=w3227) -> (x .and. y?=w3229:bool)
                n1906 = case shown="True" w3229 {
                  tunnel: w3225 -> [_ w3237]
                  tunnel: w3224 -> [_ w3239]
                  tunnel: w3223 -> [_ w3238]
                  tunnel: w3222 -> [_ w3231]
                  tunnel: w3218 -> [_ w3230]
                  frame False {
                  }
                  frame True {
                    # "check for amps fail"
                    n1907 = case shown="True" w3238 {
                      tunnel: w3237 -> [_ w3245]
                      tunnel: [FALSE w3244] -> w3235
                      tunnel: ["" "AMPS HI"] -> w3233
                      tunnel: w3230 -> [_ w3242]
                      frame False {
                      }
                      frame True {
                        n1908 = Greater?(x=w3245, y=w3242) -> (0:w3244:bool)
                      }
                    }
                    n1909 = case shown="True" w3239 {
                      tunnel: w3237 -> [_ w3251]
                      tunnel: [FALSE w3250] -> w3236
                      tunnel: ["" "AMPS LO"] -> w3232
                      tunnel: w3230 -> [_ w3248]
                      frame False {
                      }
                      frame True {
                        n1910 = Less?(x=w3251, y=w3248) -> (x < y?=w3250:bool)
                      }
                    }
                    n1911 = Or(x=w3236, y=w3235) -> (x .or. y?=w3234:bool)
                    n1912 = case shown="True" w3234 {
                      tunnel: w3233 -> [_ w3254]
                      tunnel: w3232 -> [_ w3253]
                      tunnel: w3231 -> [_ w3252]
                      frame False {
                      }
                      frame True {
                        n1913 = stacked-sequence {
                          tunnel: w3254 -> [w3259 _]
                          tunnel: w3253 -> [w3258 _]
                          tunnel: w3252 -> [w3255 _]
                          frame #0 {
                            n1914 = Build Array(w3259, w3258) -> (w3257:string[])
                            n1915 = TDMS Write(0:w3255, 5:"TEST RESULT", 7:"AMPS FAIL ", 9:w3257) -> (15:w3261:errorcluster)  [unwired: 2 in, 3 out]
                            n1916 = local write "data file error"(w3261) -> ()
                          }
                          frame #1 {
                            n1917 = local read "LAB04-2 (DISP)"() -> (w3265:T4)
                            n1918 = Bundle(cluster=w3265, "STATUS"="STOP") -> (w3264:T4)  [unwired: 2 in]
                            n1919 = local write "LAB04-2 (RESULT)"(FALSE) -> ()
                            n1920 = local write "LAB04-2 (DISP)"(w3264) -> ()
                          }
                        }
                      }
                    }
                  }
                }
              }
              frame #8 {
                # "LAB05-1"
                n1921 = local read "LAB05-1 (SIG)"() -> (w3277:T2)
                n1922 = Or(x=w3275, y=w3274) -> (x .or. y?=w3279:bool)
                n1923 = case shown="\"CYCLE TEST\"" w3270 {
                  tunnel: [FALSE TRUE FALSE] -> w3272
                  frame "TEST SET UP", Default {
                  }
                  frame "CYCLE TEST" {
                  }
                  frame "T-RISE TEST" {
                  }
                }
                n1924 = And(x=w3271, y=w3279) -> (x .and. y?=w3278:bool)
                n1925 = local read "LAB05-1 (TDMS)"() -> (w3273:refnum<k34>)
                n1926 = Unbundle(w3277) -> ("AMPS"=w3276:dbl)  [unwired: 4 out]
                n1927 = And(x=w3272, y=w3278) -> (x .and. y?=w3280:bool)
                n1928 = case shown="True" w3280 {
                  tunnel: w3276 -> [_ w3288]
                  tunnel: w3275 -> [_ w3290]
                  tunnel: w3274 -> [_ w3289]
                  tunnel: w3273 -> [_ w3282]
                  tunnel: w3269 -> [_ w3281]
                  frame False {
                  }
                  frame True {
                    # "check for amps fail"
                    n1929 = case shown="True" w3289 {
                      tunnel: w3288 -> [_ w3296]
                      tunnel: [FALSE w3295] -> w3286
                      tunnel: ["" "AMPS HI"] -> w3284
                      tunnel: w3281 -> [_ w3293]
                      frame False {
                      }
                      frame True {
                        n1930 = Greater?(x=w3296, y=w3293) -> (0:w3295:bool)
                      }
                    }
                    n1931 = case shown="True" w3290 {
                      tunnel: w3288 -> [_ w3302]
                      tunnel: [FALSE w3301] -> w3287
                      tunnel: ["" "AMPS LO"] -> w3283
                      tunnel: w3281 -> [_ w3299]
                      frame False {
                      }
                      frame True {
                        n1932 = Less?(x=w3302, y=w3299) -> (x < y?=w3301:bool)
                      }
                    }
                    n1933 = Or(x=w3287, y=w3286) -> (x .or. y?=w3285:bool)
                    n1934 = case shown="True" w3285 {
                      tunnel: w3284 -> [_ w3305]
                      tunnel: w3283 -> [_ w3304]
                      tunnel: w3282 -> [_ w3303]
                      frame False {
                      }
                      frame True {
                        n1935 = stacked-sequence {
                          tunnel: w3305 -> [w3310 _]
                          tunnel: w3304 -> [w3309 _]
                          tunnel: w3303 -> [w3306 _]
                          frame #0 {
                            n1936 = Build Array(w3310, w3309) -> (w3308:string[])
                            n1937 = TDMS Write(0:w3306, 5:"TEST RESULT", 7:"AMPS FAIL ", 9:w3308) -> (15:w3312:errorcluster)  [unwired: 2 in, 3 out]
                            n1938 = local write "data file error"(w3312) -> ()
                          }
                          frame #1 {
                            n1939 = local read "LAB05-1 (DISP)"() -> (w3316:T4)
                            n1940 = Bundle(cluster=w3316, "STATUS"="STOP") -> (w3315:T4)  [unwired: 2 in]
                            n1941 = local write "LAB05-1 (RESULT)"(FALSE) -> ()
                            n1942 = local write "LAB05-1 (DISP)"(w3315) -> ()
                          }
                        }
                      }
                    }
                  }
                }
              }
              frame #9 {
                # "LAB05-2"
                n1943 = local read "LAB05-2 (SIG)"() -> (w3328:T2)
                n1944 = Or(x=w3326, y=w3325) -> (x .or. y?=w3330:bool)
                n1945 = case shown="\"CYCLE TEST\"" w3321 {
                  tunnel: [FALSE TRUE FALSE] -> w3323
                  frame "TEST SET UP", Default {
                  }
                  frame "CYCLE TEST" {
                  }
                  frame "T-RISE TEST" {
                  }
                }
                n1946 = And(x=w3322, y=w3330) -> (x .and. y?=w3329:bool)
                n1947 = local read "LAB05-2 (TDMS)"() -> (w3324:refnum<k34>)
                n1948 = Unbundle(w3328) -> ("AMPS"=w3327:dbl)  [unwired: 4 out]
                n1949 = And(x=w3323, y=w3329) -> (x .and. y?=w3331:bool)
                n1950 = case shown="True" w3331 {
                  tunnel: w3327 -> [_ w3339]
                  tunnel: w3326 -> [_ w3341]
                  tunnel: w3325 -> [_ w3340]
                  tunnel: w3324 -> [_ w3333]
                  tunnel: w3320 -> [_ w3332]
                  frame False {
                  }
                  frame True {
                    # "check for amps fail"
                    n1951 = case shown="True" w3340 {
                      tunnel: w3339 -> [_ w3347]
                      tunnel: [FALSE w3346] -> w3337
                      tunnel: ["" "AMPS HI"] -> w3335
                      tunnel: w3332 -> [_ w3344]
                      frame False {
                      }
                      frame True {
                        n1952 = Greater?(x=w3347, y=w3344) -> (0:w3346:bool)
                      }
                    }
                    n1953 = case shown="True" w3341 {
                      tunnel: w3339 -> [_ w3353]
                      tunnel: [FALSE w3352] -> w3338
                      tunnel: ["" "AMPS LO"] -> w3334
                      tunnel: w3332 -> [_ w3350]
                      frame False {
                      }
                      frame True {
                        n1954 = Less?(x=w3353, y=w3350) -> (x < y?=w3352:bool)
                      }
                    }
                    n1955 = Or(x=w3338, y=w3337) -> (x .or. y?=w3336:bool)
                    n1956 = case shown="True" w3336 {
                      tunnel: w3335 -> [_ w3356]
                      tunnel: w3334 -> [_ w3355]
                      tunnel: w3333 -> [_ w3354]
                      frame False {
                      }
                      frame True {
                        n1957 = stacked-sequence {
                          tunnel: w3356 -> [w3361 _]
                          tunnel: w3355 -> [w3360 _]
                          tunnel: w3354 -> [w3357 _]
                          frame #0 {
                            n1958 = Build Array(w3361, w3360) -> (w3359:string[])
                            n1959 = TDMS Write(0:w3357, 5:"TEST RESULT", 7:"AMPS FAIL ", 9:w3359) -> (15:w3363:errorcluster)  [unwired: 2 in, 3 out]
                            n1960 = local write "data file error"(w3363) -> ()
                          }
                          frame #1 {
                            n1961 = local read "LAB05-2 (DISP)"() -> (w3367:T4)
                            n1962 = Bundle(cluster=w3367, "STATUS"="STOP") -> (w3366:T4)  [unwired: 2 in]
                            n1963 = local write "LAB05-2 (RESULT)"(FALSE) -> ()
                            n1964 = local write "LAB05-2 (DISP)"(w3366) -> ()
                          }
                        }
                      }
                    }
                  }
                }
              }
            }
          }
          frame #14 {
            # "check for temperature rise test fail conditions"
            n1965 = stacked-sequence {
              tunnel: w3391 -> [w3413 _ _ _ _ _ _ _ _ _]
              tunnel: w3390 -> [w3412 _ _ _ _ _ _ _ _ _]
              tunnel: w3389 -> [_ w3452 _ _ _ _ _ _ _ _]
              tunnel: w3388 -> [_ _ w3508 _ _ _ _ _ _ _]
              tunnel: w3387 -> [_ _ _ w3564 _ _ _ _ _ _]
              tunnel: w3386 -> [_ _ _ _ w3620 _ _ _ _ _]
              tunnel: w3385 -> [_ _ _ _ _ w3676 _ _ _ _]
              tunnel: w3384 -> [_ _ _ _ _ _ w3732 _ _ _]
              tunnel: w3383 -> [_ _ _ _ _ _ _ w3788 _ _]
              tunnel: w3382 -> [_ _ _ _ _ _ _ _ w3844 _]
              tunnel: w3381 -> [_ _ _ _ _ _ _ _ _ w3900]
              tunnel: w3380 -> [_ w3451 _ _ _ _ _ _ _ _]
              tunnel: w3379 -> [_ _ w3507 _ _ _ _ _ _ _]
              tunnel: w3378 -> [_ _ _ w3563 _ _ _ _ _ _]
              tunnel: w3377 -> [_ _ _ _ w3619 _ _ _ _ _]
              tunnel: w3376 -> [_ _ _ _ _ w3675 _ _ _ _]
              tunnel: w3375 -> [_ _ _ _ _ _ _ w3787 _ _]
              tunnel: w3374 -> [_ _ _ _ _ _ _ _ w3843 _]
              tunnel: w3373 -> [_ _ _ _ _ _ _ _ _ w3899]
              tunnel: w3372 -> [_ _ _ _ _ _ w3731 _ _ _]
              tunnel: 2.0 -> [w3392 w3450 w3506 w3562 w3618 w3674 w3730 w3786 w3842 w3898]
              frame #0 {
                # "LAB01-1"
                n1966 = local read "LAB01-1 (TEMP START)"() -> (w3406:cluster{"TL":dbl, "TN":dbl})
                n1967 = local read "LAB01-1 (DISP)"() -> (w3397:T4)
                n1968 = local read "LAB01-1 (SIG)"() -> (w3408:T2)
                n1969 = case shown="\"T-RISE TEST\"" w3413 {
                  tunnel: [FALSE FALSE TRUE] -> w3411
                  frame "TEST SET UP", Default {
                  }
                  frame "CYCLE TEST" {
                  }
                  frame "T-RISE TEST" {
                  }
                }
                n1970 = local read "LAB01-1 (SET)"() -> (w3401:T5)
                n1971 = Unbundle(w3408) -> ("AMPS"=w3407:dbl, "Tmp Live"=w3405:dbl, "Tmp Neut"=w3404:dbl)  [unwired: 2 out]
                n1972 = Unbundle(w3406) -> ("TL"=w3403:dbl, "TN"=w3402:dbl)
                n1973 = Unbundle(w3397) -> ("CYCLE"=w3396:dbl)  [unwired: 2 out]
                n1974 = local read "LAB01-1 (TDMS)"() -> (w3393:refnum<k34>)
                n1975 = Greater?(x=w3396, y=2.0) -> (0:w3395:bool)
                n1976 = And(x=w3412, y=w3395) -> (x .and. y?=w3409:bool)
                n1977 = Unbundle(w3401) -> ("T-RISE deg C"=w3398:dbl)  [unwired: 4 out]
                n1978 = Subtract(x=w3405, y=w3403) -> (x-y=w3400:dbl)
                n1979 = And(x=w3411, y=w3409) -> (x .and. y?=w3410:bool)
                n1980 = Subtract(x=w3404, y=w3402) -> (x-y=w3399:dbl)
                n1981 = case shown="True" w3410 {
                  tunnel: w3407 -> [_ w3430]
                  tunnel: w3400 -> [_ w3424]
                  tunnel: w3399 -> [_ w3423]
                  tunnel: w3398 -> [_ w3422]
                  tunnel: w3393 -> [_ w3415]
                  tunnel: w3392 -> [_ w3414]
                  frame False {
                  }
                  frame True {
                    # "check for amps & t-rise fail"
                    n1982 = Less?(x=w3430, y=w3414) -> (x < y?=w3417:bool)
                    n1983 = Greater?(x=w3424, y=w3422) -> (0:w3427:bool)
                    n1984 = Greater?(x=w3423, y=w3422) -> (0:w3428:bool)
                    n1985 = Or(x=w3427, y=w3428) -> (x .or. y?=w3416:bool)
                    n1986 = Select(t="AMPS LO", s=w3417, f="") -> (s? t:f=w3418:string)
                    n1987 = Select(t="T-RISE HI", s=w3416, f="") -> (s? t:f=w3419:string)
                    n1988 = Or(x=w3417, y=w3416) -> (x .or. y?=w3429:bool)
                    n1989 = case shown="True" w3429 {
                      tunnel: w3419 -> [_ w3433]
                      tunnel: w3418 -> [_ w3432]
                      tunnel: w3415 -> [_ w3431]
                      frame False {
                      }
                      frame True {
                        n1990 = stacked-sequence {
                          tunnel: w3433 -> [w3436 w3442]
                          tunnel: w3432 -> [w3435 w3443]
                          tunnel: w3431 -> [w3434 _]
                          frame #0 {
                            n1991 = Build Array(w3435, w3436) -> (w3438:string[])
                            n1992 = TDMS Write(0:w3434, 5:"TEST RESULT", 7:"T-RISE FAIL ", 9:w3438) -> (15:w3440:errorcluster)  [unwired: 2 in, 3 out]
                            n1993 = local write "data file error"(w3440) -> ()
                          }
                          frame #1 {
                            (unwired) "STOP"
                            n1994 = local read "LAB01-1 (DISP)"() -> (w3446:T4)
                            n1995 = Concatenate Strings(w3443, w3442) -> (w3441:string)
                            n1996 = Bundle(cluster=w3446, "STATUS"=w3441) -> (w3445:T4)  [unwired: 2 in]
                            n1997 = local write "LAB01-1 (RESULT)"(FALSE) -> ()
                            n1998 = local write "LAB01-1 (DISP)"(w3445) -> ()
                          }
                        }
                      }
                    }
                  }
                }
              }
              frame #1 {
                # "LAB01-2"
                n1999 = local read "LAB01-2 (TEMP START)"() -> (w3466:cluster{"TL":dbl, "TN":dbl})
                n2000 = local read "LAB01-2 (DISP)"() -> (w3457:T4)
                n2001 = local read "LAB01-2 (SIG)"() -> (w3468:T2)
                n2002 = case shown="\"T-RISE TEST\"" w3452 {
                  tunnel: [FALSE FALSE TRUE] -> w3471
                  frame "TEST SET UP", Default {
                  }
                  frame "CYCLE TEST" {
                  }
                  frame "T-RISE TEST" {
                  }
                }
                n2003 = local read "LAB01-2(SET)"() -> (w3461:T5)
                n2004 = Unbundle(w3468) -> ("AMPS"=w3467:dbl, "Tmp Live"=w3465:dbl, "Tmp Neut"=w3464:dbl)  [unwired: 2 out]
                n2005 = Unbundle(w3457) -> ("CYCLE"=w3456:dbl)  [unwired: 2 out]
                n2006 = Unbundle(w3466) -> ("TL"=w3463:dbl, "TN"=w3462:dbl)
                n2007 = local read "LAB01-2 (TDMS)"() -> (w3453:refnum<k34>)
                n2008 = Greater?(x=w3456, y=2.0) -> (0:w3455:bool)
                n2009 = And(x=w3451, y=w3455) -> (x .and. y?=w3469:bool)
                n2010 = Unbundle(w3461) -> ("T-RISE deg C"=w3458:dbl)  [unwired: 4 out]
                n2011 = Subtract(x=w3465, y=w3463) -> (x-y=w3460:dbl)
                n2012 = And(x=w3471, y=w3469) -> (x .and. y?=w3470:bool)
                n2013 = Subtract(x=w3464, y=w3462) -> (x-y=w3459:dbl)
                n2014 = case shown="True" w3470 {
                  tunnel: w3467 -> [_ w3488]
                  tunnel: w3460 -> [_ w3482]
                  tunnel: w3459 -> [_ w3481]
                  tunnel: w3458 -> [_ w3480]
                  tunnel: w3453 -> [_ w3473]
                  tunnel: w3450 -> [_ w3472]
                  frame False {
                  }
                  frame True {
                    # "check for amps & t-rise fail"
                    n2015 = Less?(x=w3488, y=w3472) -> (x < y?=w3475:bool)
                    n2016 = Greater?(x=w3482, y=w3480) -> (0:w3485:bool)
                    n2017 = Greater?(x=w3481, y=w3480) -> (0:w3486:bool)
                    n2018 = Or(x=w3485, y=w3486) -> (x .or. y?=w3474:bool)
                    n2019 = Select(t="AMPS LO", s=w3475, f="") -> (s? t:f=w3476:string)
                    n2020 = Select(t="T-RISE HI", s=w3474, f="") -> (s? t:f=w3477:string)
                    n2021 = Or(x=w3475, y=w3474) -> (x .or. y?=w3487:bool)
                    n2022 = case shown="True" w3487 {
                      tunnel: w3477 -> [_ w3491]
                      tunnel: w3476 -> [_ w3490]
                      tunnel: w3473 -> [_ w3489]
                      frame False {
                      }
                      frame True {
                        n2023 = stacked-sequence {
                          tunnel: w3491 -> [w3494 _]
                          tunnel: w3490 -> [w3493 _]
                          tunnel: w3489 -> [w3492 _]
                          frame #0 {
                            n2024 = Build Array(w3493, w3494) -> (w3496:string[])
                            n2025 = TDMS Write(0:w3492, 5:"TEST RESULT", 7:"T-RISE FAIL ", 9:w3496) -> (15:w3498:errorcluster)  [unwired: 2 in, 3 out]
                            n2026 = local write "data file error"(w3498) -> ()
                          }
                          frame #1 {
                            n2027 = local read "LAB01-2 (DISP)"() -> (w3502:T4)
                            n2028 = Bundle(cluster=w3502, "STATUS"="STOP") -> (w3501:T4)  [unwired: 2 in]
                            n2029 = local write "LAB01-2 (RESULT)"(FALSE) -> ()
                            n2030 = local write "LAB01-2 (DISP)"(w3501) -> ()
                          }
                        }
                      }
                    }
                  }
                }
              }
              frame #2 {
                # "LAB02-1"
                n2031 = local read "LAB02-1 (TEMP START)"() -> (w3522:cluster{"TL":dbl, "TN":dbl})
                n2032 = local read "LAB02-1 (DISP)"() -> (w3513:T4)
                n2033 = local read "LAB02-1 (SIG)"() -> (w3524:T2)
                n2034 = case shown="\"T-RISE TEST\"" w3508 {
                  tunnel: [FALSE FALSE TRUE] -> w3527
                  frame "TEST SET UP", Default {
                  }
                  frame "CYCLE TEST" {
                  }
                  frame "T-RISE TEST" {
                  }
                }
                n2035 = local read "LAB02-1 (SET)"() -> (w3517:T5)
                n2036 = Unbundle(w3524) -> ("AMPS"=w3523:dbl, "Tmp Live"=w3521:dbl, "Tmp Neut"=w3520:dbl)  [unwired: 2 out]
                n2037 = Unbundle(w3513) -> ("CYCLE"=w3512:dbl)  [unwired: 2 out]
                n2038 = Unbundle(w3522) -> ("TL"=w3519:dbl, "TN"=w3518:dbl)
                n2039 = local read "LAB02-1 (TDMS)"() -> (w3509:refnum<k34>)
                n2040 = Greater?(x=w3512, y=2.0) -> (0:w3511:bool)
                n2041 = And(x=w3507, y=w3511) -> (x .and. y?=w3525:bool)
                n2042 = Unbundle(w3517) -> ("T-RISE deg C"=w3514:dbl)  [unwired: 4 out]
                n2043 = Subtract(x=w3521, y=w3519) -> (x-y=w3516:dbl)
                n2044 = And(x=w3527, y=w3525) -> (x .and. y?=w3526:bool)
                n2045 = Subtract(x=w3520, y=w3518) -> (x-y=w3515:dbl)
                n2046 = case shown="True" w3526 {
                  tunnel: w3523 -> [_ w3544]
                  tunnel: w3516 -> [_ w3538]
                  tunnel: w3515 -> [_ w3537]
                  tunnel: w3514 -> [_ w3536]
                  tunnel: w3509 -> [_ w3529]
                  tunnel: w3506 -> [_ w3528]
                  frame False {
                  }
                  frame True {
                    # "check for amps & t-rise fail"
                    n2047 = Less?(x=w3544, y=w3528) -> (x < y?=w3531:bool)
                    n2048 = Greater?(x=w3538, y=w3536) -> (0:w3541:bool)
                    n2049 = Greater?(x=w3537, y=w3536) -> (0:w3542:bool)
                    n2050 = Or(x=w3541, y=w3542) -> (x .or. y?=w3530:bool)
                    n2051 = Select(t="AMPS LO", s=w3531, f="") -> (s? t:f=w3532:string)
                    n2052 = Select(t="T-RISE HI", s=w3530, f="") -> (s? t:f=w3533:string)
                    n2053 = Or(x=w3531, y=w3530) -> (x .or. y?=w3543:bool)
                    n2054 = case shown="True" w3543 {
                      tunnel: w3533 -> [_ w3547]
                      tunnel: w3532 -> [_ w3546]
                      tunnel: w3529 -> [_ w3545]
                      frame False {
                      }
                      frame True {
                        n2055 = stacked-sequence {
                          tunnel: w3547 -> [w3550 _]
                          tunnel: w3546 -> [w3549 _]
                          tunnel: w3545 -> [w3548 _]
                          frame #0 {
                            n2056 = Build Array(w3549, w3550) -> (w3552:string[])
                            n2057 = TDMS Write(0:w3548, 5:"TEST RESULT", 7:"T-RISE FAIL ", 9:w3552) -> (15:w3554:errorcluster)  [unwired: 2 in, 3 out]
                            n2058 = local write "data file error"(w3554) -> ()
                          }
                          frame #1 {
                            n2059 = local read "LAB02-1 (DISP)"() -> (w3558:T4)
                            n2060 = Bundle(cluster=w3558, "STATUS"="STOP") -> (w3557:T4)  [unwired: 2 in]
                            n2061 = local write "LAB02-1 (RESULT)"(FALSE) -> ()
                            n2062 = local write "LAB02-1 (DISP)"(w3557) -> ()
                          }
                        }
                      }
                    }
                  }
                }
              }
              frame #3 {
                # "LAB02-2"
                n2063 = local read "LAB02-2 (TEMP START)"() -> (w3578:cluster{"TL":dbl, "TN":dbl})
                n2064 = local read "LAB02-2 (DISP)"() -> (w3569:T4)
                n2065 = local read "LAB02-2 (SIG)"() -> (w3580:T2)
                n2066 = case shown="\"T-RISE TEST\"" w3564 {
                  tunnel: [FALSE FALSE TRUE] -> w3583
                  frame "TEST SET UP", Default {
                  }
                  frame "CYCLE TEST" {
                  }
                  frame "T-RISE TEST" {
                  }
                }
                n2067 = local read "LAB02-2 (SET)"() -> (w3573:T5)
                n2068 = Unbundle(w3580) -> ("AMPS"=w3579:dbl, "Tmp Live"=w3577:dbl, "Tmp Neut"=w3576:dbl)  [unwired: 2 out]
                n2069 = Unbundle(w3569) -> ("CYCLE"=w3568:dbl)  [unwired: 2 out]
                n2070 = Unbundle(w3578) -> ("TL"=w3575:dbl, "TN"=w3574:dbl)
                n2071 = local read "LAB02-2 (TDMS)"() -> (w3565:refnum<k34>)
                n2072 = Greater?(x=w3568, y=2.0) -> (0:w3567:bool)
                n2073 = And(x=w3563, y=w3567) -> (x .and. y?=w3581:bool)
                n2074 = Unbundle(w3573) -> ("T-RISE deg C"=w3570:dbl)  [unwired: 4 out]
                n2075 = Subtract(x=w3577, y=w3575) -> (x-y=w3572:dbl)
                n2076 = And(x=w3583, y=w3581) -> (x .and. y?=w3582:bool)
                n2077 = Subtract(x=w3576, y=w3574) -> (x-y=w3571:dbl)
                n2078 = case shown="True" w3582 {
                  tunnel: w3579 -> [_ w3600]
                  tunnel: w3572 -> [_ w3594]
                  tunnel: w3571 -> [_ w3593]
                  tunnel: w3570 -> [_ w3592]
                  tunnel: w3565 -> [_ w3585]
                  tunnel: w3562 -> [_ w3584]
                  frame False {
                  }
                  frame True {
                    # "check for amps & t-rise fail"
                    n2079 = Less?(x=w3600, y=w3584) -> (x < y?=w3587:bool)
                    n2080 = Greater?(x=w3594, y=w3592) -> (0:w3597:bool)
                    n2081 = Greater?(x=w3593, y=w3592) -> (0:w3598:bool)
                    n2082 = Or(x=w3597, y=w3598) -> (x .or. y?=w3586:bool)
                    n2083 = Select(t="AMPS LO", s=w3587, f="") -> (s? t:f=w3588:string)
                    n2084 = Select(t="T-RISE HI", s=w3586, f="") -> (s? t:f=w3589:string)
                    n2085 = Or(x=w3587, y=w3586) -> (x .or. y?=w3599:bool)
                    n2086 = case shown="True" w3599 {
                      tunnel: w3589 -> [_ w3603]
                      tunnel: w3588 -> [_ w3602]
                      tunnel: w3585 -> [_ w3601]
                      frame False {
                      }
                      frame True {
                        n2087 = stacked-sequence {
                          tunnel: w3603 -> [w3606 _]
                          tunnel: w3602 -> [w3605 _]
                          tunnel: w3601 -> [w3604 _]
                          frame #0 {
                            n2088 = Build Array(w3605, w3606) -> (w3608:string[])
                            n2089 = TDMS Write(0:w3604, 5:"TEST RESULT", 7:"T-RISE FAIL ", 9:w3608) -> (15:w3610:errorcluster)  [unwired: 2 in, 3 out]
                            n2090 = local write "data file error"(w3610) -> ()
                          }
                          frame #1 {
                            n2091 = local read "LAB02-2 (DISP)"() -> (w3614:T4)
                            n2092 = Bundle(cluster=w3614, "STATUS"="STOP") -> (w3613:T4)  [unwired: 2 in]
                            n2093 = local write "LAB02-2 (RESULT)"(FALSE) -> ()
                            n2094 = local write "LAB02-2 (DISP)"(w3613) -> ()
                          }
                        }
                      }
                    }
                  }
                }
              }
              frame #4 {
                # "LAB03-1"
                n2095 = local read "LAB03-1 (TEMP START)"() -> (w3634:cluster{"TL":dbl, "TN":dbl})
                n2096 = local read "LAB03-1 (DISP)"() -> (w3625:T4)
                n2097 = local read "LAB03-1 (SIG)"() -> (w3636:T2)
                n2098 = case shown="\"T-RISE TEST\"" w3620 {
                  tunnel: [FALSE FALSE TRUE] -> w3639
                  frame "TEST SET UP", Default {
                  }
                  frame "CYCLE TEST" {
                  }
                  frame "T-RISE TEST" {
                  }
                }
                n2099 = local read "LAB03-1 (SET)"() -> (w3629:T5)
                n2100 = Unbundle(w3636) -> ("AMPS"=w3635:dbl, "Tmp Live"=w3633:dbl, "Tmp Neut"=w3632:dbl)  [unwired: 2 out]
                n2101 = Unbundle(w3625) -> ("CYCLE"=w3624:dbl)  [unwired: 2 out]
                n2102 = Unbundle(w3634) -> ("TL"=w3631:dbl, "TN"=w3630:dbl)
                n2103 = local read "LAB03-1 (TDMS)"() -> (w3621:refnum<k34>)
                n2104 = Greater?(x=w3624, y=2.0) -> (0:w3623:bool)
                n2105 = And(x=w3619, y=w3623) -> (x .and. y?=w3637:bool)
                n2106 = Unbundle(w3629) -> ("T-RISE deg C"=w3626:dbl)  [unwired: 4 out]
                n2107 = Subtract(x=w3633, y=w3631) -> (x-y=w3628:dbl)
                n2108 = And(x=w3639, y=w3637) -> (x .and. y?=w3638:bool)
                n2109 = Subtract(x=w3632, y=w3630) -> (x-y=w3627:dbl)
                n2110 = case shown="True" w3638 {
                  tunnel: w3635 -> [_ w3656]
                  tunnel: w3628 -> [_ w3650]
                  tunnel: w3627 -> [_ w3649]
                  tunnel: w3626 -> [_ w3648]
                  tunnel: w3621 -> [_ w3641]
                  tunnel: w3618 -> [_ w3640]
                  frame False {
                  }
                  frame True {
                    # "check for amps & t-rise fail"
                    n2111 = Less?(x=w3656, y=w3640) -> (x < y?=w3643:bool)
                    n2112 = Greater?(x=w3650, y=w3648) -> (0:w3653:bool)
                    n2113 = Greater?(x=w3649, y=w3648) -> (0:w3654:bool)
                    n2114 = Or(x=w3653, y=w3654) -> (x .or. y?=w3642:bool)
                    n2115 = Select(t="AMPS LO", s=w3643, f="") -> (s? t:f=w3644:string)
                    n2116 = Select(t="T-RISE HI", s=w3642, f="") -> (s? t:f=w3645:string)
                    n2117 = Or(x=w3643, y=w3642) -> (x .or. y?=w3655:bool)
                    n2118 = case shown="True" w3655 {
                      tunnel: w3645 -> [_ w3659]
                      tunnel: w3644 -> [_ w3658]
                      tunnel: w3641 -> [_ w3657]
                      frame False {
                      }
                      frame True {
                        n2119 = stacked-sequence {
                          tunnel: w3659 -> [w3662 _]
                          tunnel: w3658 -> [w3661 _]
                          tunnel: w3657 -> [w3660 _]
                          frame #0 {
                            n2120 = Build Array(w3661, w3662) -> (w3664:string[])
                            n2121 = TDMS Write(0:w3660, 5:"TEST RESULT", 7:"T-RISE FAIL ", 9:w3664) -> (15:w3666:errorcluster)  [unwired: 2 in, 3 out]
                            n2122 = local write "data file error"(w3666) -> ()
                          }
                          frame #1 {
                            n2123 = local read "LAB03-1 (DISP)"() -> (w3670:T4)
                            n2124 = Bundle(cluster=w3670, "STATUS"="STOP") -> (w3669:T4)  [unwired: 2 in]
                            n2125 = local write "LAB03-1 (RESULT)"(FALSE) -> ()
                            n2126 = local write "LAB03-1 (DISP)"(w3669) -> ()
                          }
                        }
                      }
                    }
                  }
                }
              }
              frame #5 {
                # "LAB03-2"
                n2127 = local read "LAB03-2 (TEMP START)"() -> (w3690:cluster{"TL":dbl, "TN":dbl})
                n2128 = local read "LAB03-2 (SIG)"() -> (w3692:T2)
                n2129 = local read "LAB03-2 (DISP)"() -> (w3681:T4)
                n2130 = case shown="\"T-RISE TEST\"" w3676 {
                  tunnel: [FALSE FALSE TRUE] -> w3695
                  frame "TEST SET UP", Default {
                  }
                  frame "CYCLE TEST" {
                  }
                  frame "T-RISE TEST" {
                  }
                }
                n2131 = local read "LAB03-2 (SET)"() -> (w3685:T5)
                n2132 = Unbundle(w3692) -> ("AMPS"=w3691:dbl, "Tmp Live"=w3689:dbl, "Tmp Neut"=w3688:dbl)  [unwired: 2 out]
                n2133 = Unbundle(w3681) -> ("CYCLE"=w3680:dbl)  [unwired: 2 out]
                n2134 = Unbundle(w3690) -> ("TL"=w3687:dbl, "TN"=w3686:dbl)
                n2135 = local read "LAB03-2 (TDMS)"() -> (w3677:refnum<k34>)
                n2136 = Greater?(x=w3680, y=2.0) -> (0:w3679:bool)
                n2137 = And(x=w3675, y=w3679) -> (x .and. y?=w3693:bool)
                n2138 = Unbundle(w3685) -> ("T-RISE deg C"=w3682:dbl)  [unwired: 4 out]
                n2139 = Subtract(x=w3689, y=w3687) -> (x-y=w3684:dbl)
                n2140 = And(x=w3695, y=w3693) -> (x .and. y?=w3694:bool)
                n2141 = Subtract(x=w3688, y=w3686) -> (x-y=w3683:dbl)
                n2142 = case shown="True" w3694 {
                  tunnel: w3691 -> [_ w3712]
                  tunnel: w3684 -> [_ w3706]
                  tunnel: w3683 -> [_ w3705]
                  tunnel: w3682 -> [_ w3704]
                  tunnel: w3677 -> [_ w3697]
                  tunnel: w3674 -> [_ w3696]
                  frame False {
                  }
                  frame True {
                    # "check for amps & t-rise fail"
                    n2143 = Less?(x=w3712, y=w3696) -> (x < y?=w3699:bool)
                    n2144 = Greater?(x=w3706, y=w3704) -> (0:w3709:bool)
                    n2145 = Greater?(x=w3705, y=w3704) -> (0:w3710:bool)
                    n2146 = Or(x=w3709, y=w3710) -> (x .or. y?=w3698:bool)
                    n2147 = Select(t="AMPS LO", s=w3699, f="") -> (s? t:f=w3700:string)
                    n2148 = Select(t="T-RISE HI", s=w3698, f="") -> (s? t:f=w3701:string)
                    n2149 = Or(x=w3699, y=w3698) -> (x .or. y?=w3711:bool)
                    n2150 = case shown="True" w3711 {
                      tunnel: w3701 -> [_ w3715]
                      tunnel: w3700 -> [_ w3714]
                      tunnel: w3697 -> [_ w3713]
                      frame False {
                      }
                      frame True {
                        n2151 = stacked-sequence {
                          tunnel: w3715 -> [w3718 _]
                          tunnel: w3714 -> [w3717 _]
                          tunnel: w3713 -> [w3716 _]
                          frame #0 {
                            n2152 = Build Array(w3717, w3718) -> (w3720:string[])
                            n2153 = TDMS Write(0:w3716, 5:"TEST RESULT", 7:"T-RISE FAIL ", 9:w3720) -> (15:w3722:errorcluster)  [unwired: 2 in, 3 out]
                            n2154 = local write "data file error"(w3722) -> ()
                          }
                          frame #1 {
                            n2155 = local read "LAB03-2 (DISP)"() -> (w3726:T4)
                            n2156 = Bundle(cluster=w3726, "STATUS"="STOP") -> (w3725:T4)  [unwired: 2 in]
                            n2157 = local write "LAB03-2 (RESULT)"(FALSE) -> ()
                            n2158 = local write "LAB03-2 (DISP)"(w3725) -> ()
                          }
                        }
                      }
                    }
                  }
                }
              }
              frame #6 {
                # "LAB04-1"
                n2159 = local read "LAB04-1 (TEMP START)"() -> (w3746:cluster{"TL":dbl, "TN":dbl})
                n2160 = local read "LAB04-1 (SIG)"() -> (w3748:T2)
                n2161 = local read "LAB04-1 (DISP)"() -> (w3737:T4)
                n2162 = case shown="\"T-RISE TEST\"" w3732 {
                  tunnel: [FALSE FALSE TRUE] -> w3751
                  frame "TEST SET UP", Default {
                  }
                  frame "CYCLE TEST" {
                  }
                  frame "T-RISE TEST" {
                  }
                }
                n2163 = local read "LAB04-1 (SET)"() -> (w3741:T5)
                n2164 = Unbundle(w3748) -> ("AMPS"=w3747:dbl, "Tmp Live"=w3745:dbl, "Tmp Neut"=w3744:dbl)  [unwired: 2 out]
                n2165 = Unbundle(w3737) -> ("CYCLE"=w3736:dbl)  [unwired: 2 out]
                n2166 = Unbundle(w3746) -> ("TL"=w3743:dbl, "TN"=w3742:dbl)
                n2167 = local read "LAB04-1 (TDMS)"() -> (w3733:refnum<k34>)
                n2168 = Greater?(x=w3736, y=2.0) -> (0:w3735:bool)
                n2169 = And(x=w3731, y=w3735) -> (x .and. y?=w3749:bool)
                n2170 = Unbundle(w3741) -> ("T-RISE deg C"=w3738:dbl)  [unwired: 4 out]
                n2171 = Subtract(x=w3745, y=w3743) -> (x-y=w3740:dbl)
                n2172 = And(x=w3751, y=w3749) -> (x .and. y?=w3750:bool)
                n2173 = Subtract(x=w3744, y=w3742) -> (x-y=w3739:dbl)
                n2174 = case shown="True" w3750 {
                  tunnel: w3747 -> [_ w3768]
                  tunnel: w3740 -> [_ w3762]
                  tunnel: w3739 -> [_ w3761]
                  tunnel: w3738 -> [_ w3760]
                  tunnel: w3733 -> [_ w3753]
                  tunnel: w3730 -> [_ w3752]
                  frame False {
                  }
                  frame True {
                    # "check for amps & t-rise fail"
                    n2175 = Less?(x=w3768, y=w3752) -> (x < y?=w3755:bool)
                    n2176 = Greater?(x=w3762, y=w3760) -> (0:w3765:bool)
                    n2177 = Greater?(x=w3761, y=w3760) -> (0:w3766:bool)
                    n2178 = Or(x=w3765, y=w3766) -> (x .or. y?=w3754:bool)
                    n2179 = Select(t="AMPS LO", s=w3755, f="") -> (s? t:f=w3756:string)
                    n2180 = Select(t="T-RISE HI", s=w3754, f="") -> (s? t:f=w3757:string)
                    n2181 = Or(x=w3755, y=w3754) -> (x .or. y?=w3767:bool)
                    n2182 = case shown="True" w3767 {
                      tunnel: w3757 -> [_ w3771]
                      tunnel: w3756 -> [_ w3770]
                      tunnel: w3753 -> [_ w3769]
                      frame False {
                      }
                      frame True {
                        n2183 = stacked-sequence {
                          tunnel: w3771 -> [w3774 _]
                          tunnel: w3770 -> [w3773 _]
                          tunnel: w3769 -> [w3772 _]
                          frame #0 {
                            n2184 = Build Array(w3773, w3774) -> (w3776:string[])
                            n2185 = TDMS Write(0:w3772, 5:"TEST RESULT", 7:"T-RISE FAIL ", 9:w3776) -> (15:w3778:errorcluster)  [unwired: 2 in, 3 out]
                            n2186 = local write "data file error"(w3778) -> ()
                          }
                          frame #1 {
                            n2187 = local read "LAB04-1 (DISP)"() -> (w3782:T4)
                            n2188 = Bundle(cluster=w3782, "STATUS"="STOP") -> (w3781:T4)  [unwired: 2 in]
                            n2189 = local write "LAB04-1 (RESULT)"(FALSE) -> ()
                            n2190 = local write "LAB04-1 (DISP)"(w3781) -> ()
                          }
                        }
                      }
                    }
                  }
                }
              }
              frame #7 {
                # "LAB04-2"
                n2191 = local read "LAB04-2 (TEMP START)"() -> (w3802:cluster{"TL":dbl, "TN":dbl})
                n2192 = local read "LAB04-2 (SIG)"() -> (w3804:T2)
                n2193 = local read "LAB04-2 (DISP)"() -> (w3793:T4)
                n2194 = case shown="\"T-RISE TEST\"" w3788 {
                  tunnel: [FALSE FALSE TRUE] -> w3807
                  frame "TEST SET UP", Default {
                  }
                  frame "CYCLE TEST" {
                  }
                  frame "T-RISE TEST" {
                  }
                }
                n2195 = local read "LAB04-2 (SET)"() -> (w3797:T5)
                n2196 = Unbundle(w3804) -> ("AMPS"=w3803:dbl, "Tmp Live"=w3801:dbl, "Tmp Neut"=w3800:dbl)  [unwired: 2 out]
                n2197 = Unbundle(w3793) -> ("CYCLE"=w3792:dbl)  [unwired: 2 out]
                n2198 = Unbundle(w3802) -> ("TL"=w3799:dbl, "TN"=w3798:dbl)
                n2199 = local read "LAB04-2 (TDMS)"() -> (w3789:refnum<k34>)
                n2200 = Greater?(x=w3792, y=2.0) -> (0:w3791:bool)
                n2201 = And(x=w3787, y=w3791) -> (x .and. y?=w3805:bool)
                n2202 = Unbundle(w3797) -> ("T-RISE deg C"=w3794:dbl)  [unwired: 4 out]
                n2203 = Subtract(x=w3801, y=w3799) -> (x-y=w3796:dbl)
                n2204 = And(x=w3807, y=w3805) -> (x .and. y?=w3806:bool)
                n2205 = Subtract(x=w3800, y=w3798) -> (x-y=w3795:dbl)
                n2206 = case shown="True" w3806 {
                  tunnel: w3803 -> [_ w3824]
                  tunnel: w3796 -> [_ w3818]
                  tunnel: w3795 -> [_ w3817]
                  tunnel: w3794 -> [_ w3816]
                  tunnel: w3789 -> [_ w3809]
                  tunnel: w3786 -> [_ w3808]
                  frame False {
                  }
                  frame True {
                    # "check for amps & t-rise fail"
                    n2207 = Less?(x=w3824, y=w3808) -> (x < y?=w3811:bool)
                    n2208 = Greater?(x=w3818, y=w3816) -> (0:w3821:bool)
                    n2209 = Greater?(x=w3817, y=w3816) -> (0:w3822:bool)
                    n2210 = Or(x=w3821, y=w3822) -> (x .or. y?=w3810:bool)
                    n2211 = Select(t="AMPS LO", s=w3811, f="") -> (s? t:f=w3812:string)
                    n2212 = Select(t="T-RISE HI", s=w3810, f="") -> (s? t:f=w3813:string)
                    n2213 = Or(x=w3811, y=w3810) -> (x .or. y?=w3823:bool)
                    n2214 = case shown="True" w3823 {
                      tunnel: w3813 -> [_ w3827]
                      tunnel: w3812 -> [_ w3826]
                      tunnel: w3809 -> [_ w3825]
                      frame False {
                      }
                      frame True {
                        n2215 = stacked-sequence {
                          tunnel: w3827 -> [w3830 _]
                          tunnel: w3826 -> [w3829 _]
                          tunnel: w3825 -> [w3828 _]
                          frame #0 {
                            n2216 = Build Array(w3829, w3830) -> (w3832:string[])
                            n2217 = TDMS Write(0:w3828, 5:"TEST RESULT", 7:"T-RISE FAIL ", 9:w3832) -> (15:w3834:errorcluster)  [unwired: 2 in, 3 out]
                            n2218 = local write "data file error"(w3834) -> ()
                          }
                          frame #1 {
                            n2219 = local read "LAB04-2 (DISP)"() -> (w3838:T4)
                            n2220 = Bundle(cluster=w3838, "STATUS"="STOP") -> (w3837:T4)  [unwired: 2 in]
                            n2221 = local write "LAB04-2 (RESULT)"(FALSE) -> ()
                            n2222 = local write "LAB04-2 (DISP)"(w3837) -> ()
                          }
                        }
                      }
                    }
                  }
                }
              }
              frame #8 {
                # "LAB05-1"
                n2223 = local read "LAB05-1 (TEMP START)"() -> (w3858:cluster{"TL":dbl, "TN":dbl})
                n2224 = local read "LAB05-1 (SIG)"() -> (w3860:T2)
                n2225 = local read "LAB05-1 (DISP)"() -> (w3849:T4)
                n2226 = case shown="\"T-RISE TEST\"" w3844 {
                  tunnel: [FALSE FALSE TRUE] -> w3863
                  frame "TEST SET UP", Default {
                  }
                  frame "CYCLE TEST" {
                  }
                  frame "T-RISE TEST" {
                  }
                }
                n2227 = local read "LAB05-1 (SET)"() -> (w3853:T5)
                n2228 = Unbundle(w3860) -> ("AMPS"=w3859:dbl, "Tmp Live"=w3857:dbl, "Tmp Neut"=w3856:dbl)  [unwired: 2 out]
                n2229 = Unbundle(w3849) -> ("CYCLE"=w3848:dbl)  [unwired: 2 out]
                n2230 = Unbundle(w3858) -> ("TL"=w3855:dbl, "TN"=w3854:dbl)
                n2231 = local read "LAB05-1 (TDMS)"() -> (w3845:refnum<k34>)
                n2232 = Greater?(x=w3848, y=2.0) -> (0:w3847:bool)
                n2233 = And(x=w3843, y=w3847) -> (x .and. y?=w3861:bool)
                n2234 = Unbundle(w3853) -> ("T-RISE deg C"=w3850:dbl)  [unwired: 4 out]
                n2235 = Subtract(x=w3857, y=w3855) -> (x-y=w3852:dbl)
                n2236 = And(x=w3863, y=w3861) -> (x .and. y?=w3862:bool)
                n2237 = Subtract(x=w3856, y=w3854) -> (x-y=w3851:dbl)
                n2238 = case shown="True" w3862 {
                  tunnel: w3859 -> [_ w3880]
                  tunnel: w3852 -> [_ w3874]
                  tunnel: w3851 -> [_ w3873]
                  tunnel: w3850 -> [_ w3872]
                  tunnel: w3845 -> [_ w3865]
                  tunnel: w3842 -> [_ w3864]
                  frame False {
                  }
                  frame True {
                    # "check for amps & t-rise fail"
                    n2239 = Less?(x=w3880, y=w3864) -> (x < y?=w3867:bool)
                    n2240 = Greater?(x=w3874, y=w3872) -> (0:w3877:bool)
                    n2241 = Greater?(x=w3873, y=w3872) -> (0:w3878:bool)
                    n2242 = Or(x=w3877, y=w3878) -> (x .or. y?=w3866:bool)
                    n2243 = Select(t="AMPS LO", s=w3867, f="") -> (s? t:f=w3868:string)
                    n2244 = Select(t="T-RISE HI", s=w3866, f="") -> (s? t:f=w3869:string)
                    n2245 = Or(x=w3867, y=w3866) -> (x .or. y?=w3879:bool)
                    n2246 = case shown="True" w3879 {
                      tunnel: w3869 -> [_ w3883]
                      tunnel: w3868 -> [_ w3882]
                      tunnel: w3865 -> [_ w3881]
                      frame False {
                      }
                      frame True {
                        n2247 = stacked-sequence {
                          tunnel: w3883 -> [w3886 _]
                          tunnel: w3882 -> [w3885 _]
                          tunnel: w3881 -> [w3884 _]
                          frame #0 {
                            n2248 = Build Array(w3885, w3886) -> (w3888:string[])
                            n2249 = TDMS Write(0:w3884, 5:"TEST RESULT", 7:"T-RISE FAIL ", 9:w3888) -> (15:w3890:errorcluster)  [unwired: 2 in, 3 out]
                            n2250 = local write "data file error"(w3890) -> ()
                          }
                          frame #1 {
                            n2251 = local read "LAB05-1 (DISP)"() -> (w3894:T4)
                            n2252 = Bundle(cluster=w3894, "STATUS"="STOP") -> (w3893:T4)  [unwired: 2 in]
                            n2253 = local write "LAB05-1 (RESULT)"(FALSE) -> ()
                            n2254 = local write "LAB05-1 (DISP)"(w3893) -> ()
                          }
                        }
                      }
                    }
                  }
                }
              }
              frame #9 {
                # "LAB05-2"
                n2255 = local read "LAB05-2 (TEMP START)"() -> (w3914:cluster{"TL":dbl, "TN":dbl})
                n2256 = local read "LAB05-2 (DISP)"() -> (w3905:T4)
                n2257 = local read "LAB05-2 (SIG)"() -> (w3916:T2)
                n2258 = case shown="\"T-RISE TEST\"" w3900 {
                  tunnel: [FALSE FALSE TRUE] -> w3919
                  frame "TEST SET UP", Default {
                  }
                  frame "CYCLE TEST" {
                  }
                  frame "T-RISE TEST" {
                  }
                }
                n2259 = local read "LAB05-2 (SET)"() -> (w3909:T5)
                n2260 = Unbundle(w3905) -> ("CYCLE"=w3904:dbl)  [unwired: 2 out]
                n2261 = Unbundle(w3916) -> ("AMPS"=w3915:dbl, "Tmp Live"=w3913:dbl, "Tmp Neut"=w3912:dbl)  [unwired: 2 out]
                n2262 = Unbundle(w3914) -> ("TL"=w3911:dbl, "TN"=w3910:dbl)
                n2263 = Greater?(x=w3904, y=2.0) -> (0:w3903:bool)
                n2264 = local read "LAB05-2 (TDMS)"() -> (w3901:refnum<k34>)
                n2265 = And(x=w3899, y=w3903) -> (x .and. y?=w3917:bool)
                n2266 = Unbundle(w3909) -> ("T-RISE deg C"=w3906:dbl)  [unwired: 4 out]
                n2267 = Subtract(x=w3913, y=w3911) -> (x-y=w3908:dbl)
                n2268 = And(x=w3919, y=w3917) -> (x .and. y?=w3918:bool)
                n2269 = Subtract(x=w3912, y=w3910) -> (x-y=w3907:dbl)
                n2270 = case shown="True" w3918 {
                  tunnel: w3915 -> [_ w3936]
                  tunnel: w3908 -> [_ w3930]
                  tunnel: w3907 -> [_ w3929]
                  tunnel: w3906 -> [_ w3928]
                  tunnel: w3901 -> [_ w3921]
                  tunnel: w3898 -> [_ w3920]
                  frame False {
                  }
                  frame True {
                    # "check for amps & t-rise fail"
                    n2271 = Less?(x=w3936, y=w3920) -> (x < y?=w3923:bool)
                    n2272 = Greater?(x=w3930, y=w3928) -> (0:w3933:bool)
                    n2273 = Greater?(x=w3929, y=w3928) -> (0:w3934:bool)
                    n2274 = Or(x=w3933, y=w3934) -> (x .or. y?=w3922:bool)
                    n2275 = Select(t="AMPS LO", s=w3923, f="") -> (s? t:f=w3924:string)
                    n2276 = Select(t="T-RISE HI", s=w3922, f="") -> (s? t:f=w3925:string)
                    n2277 = Or(x=w3923, y=w3922) -> (x .or. y?=w3935:bool)
                    n2278 = case shown="True" w3935 {
                      tunnel: w3925 -> [_ w3939]
                      tunnel: w3924 -> [_ w3938]
                      tunnel: w3921 -> [_ w3937]
                      frame False {
                      }
                      frame True {
                        n2279 = stacked-sequence {
                          tunnel: w3939 -> [w3942 w3948]
                          tunnel: w3938 -> [w3941 w3949]
                          tunnel: w3937 -> [w3940 _]
                          frame #0 {
                            n2280 = Build Array(w3941, w3942) -> (w3944:string[])
                            n2281 = TDMS Write(0:w3940, 5:"TEST RESULT", 7:"T-RISE FAIL ", 9:w3944) -> (15:w3946:errorcluster)  [unwired: 2 in, 3 out]
                            n2282 = local write "data file error"(w3946) -> ()
                          }
                          frame #1 {
                            (unwired) "STOP"
                            n2283 = local read "LAB05-2 (DISP)"() -> (w3952:T4)
                            n2284 = Concatenate Strings(w3949, w3948) -> (w3947:string)
                            n2285 = Bundle(cluster=w3952, "STATUS"=w3947) -> (w3951:T4)  [unwired: 2 in]
                            n2286 = local write "LAB05-2 (RESULT)"(FALSE) -> ()
                            n2287 = local write "LAB05-2 (DISP)"(w3951) -> ()
                          }
                        }
                      }
                    }
                  }
                }
              }
            }
          }
          frame #15 {
            # "run calibration routine"
            n2288 = local read "CALIBRATE"() -> (w3956:bool)
            n2289 = case shown="True" w3956 {
              frame False {
              }
              frame True {
                n2290 = stacked-sequence {
                  seq-local: [w3957 _ _] -> [_ w3959 _]
                  frame #0 {
                    n2291 = call "CALIBRATION PASSWORD"() -> ("PASSWORD"=w3957:string)  [unwired: 17 in, 2 out]
                  }
                  frame #1 {
                    n2292 = Equal?(x=w3959, y="7777") -> (x = y?=w3958:bool)
                    n2293 = case shown="True" w3958 {
                      frame False {
                      }
                      frame True {
                        n2294 = stacked-sequence {
                          frame #0 {
                            n2295 = call "sub vi - calibration v1.vi"() -> ()  [unwired: 12 in]
                          }
                          frame #1 {
                            n2296 = call "sub vi - get calibration values v1.vi"() -> ("LAB01 (CAL)"=w3965:T6, "LAB02 (CAL)"=w3964:T7, "LAB03 (CAL)"=w3963:T6, "LAB04 (CAL)"=w3962:T6, "calibration file error out"=w3966:errorcluster, "LAB05 (CAL)"=w3961:T6)  [unwired: 10 in]
                            n2297 = local write "calibration file error out"(w3966) -> ()
                            n2298 = local write "LAB04 (CAL)"(w3962) -> ()
                            n2299 = local write "LAB05 (CAL)"(w3961) -> ()
                            n2300 = local write "LAB01 (CAL)"(w3965) -> ()
                            n2301 = local write "LAB02 (CAL)"(w3964) -> ()
                            n2302 = local write "LAB03 (CAL)"(w3963) -> ()
                          }
                        }
                      }
                    }
                  }
                  frame #2 {
                    n2303 = local write "CALIBRATE"(FALSE) -> ()
                  }
                }
              }
            }
          }
        }
        n2304 = node-c288() -> ()  [unwired: 1 in, 1 out]
        "loops" <- w33
      }
      n2305 = node-c288(w10) -> ()  [unwired: 1 out]
    }
  }
